vi "Q14070-Z060A.vi"() -> ()   [LabVIEW 2013]
uses:
  <vilib>/Utility/error.llb/whitespace.ctl
  <vilib>/Utility/file.llb/Read From Spreadsheet File (string).vi
  <vilib>/express/express arith-compare/Formula/XNode/ExpressFormulaBlockNode.xnode
  PCI8622_32.dll
  <vilib>/printing/EasyPrintingControls.llb/contents.ctl
  <vilib>/Utility/NIReport.llb/NI_ReportGenerationCore.lvlib
  <vilib>/printing/EasyPrintingControls.llb/report_type.ctl
  <vilib>/Utility/NIReport.llb/NI_report.lvclass
  <vilib>/printing/EasyPrinting.llb/Easy Print VI Panel or Documentation (path).vi
panel:
  in  "截取百分比":dbl=0.05
  in  "半行程":dbl=70.0
  in  "是否取消放行按钮":bool
  in  "齿条传动比":dbl=47.34 format="%#_13g"
  in  "机械间隙值":dbl=3.5
  out "最大轴向力标准(N)":dbl=200.0 caption="L+Lmax(mm)" format="%#.3f"
  out "右平均轴向力(N)":dbl caption="L+Lmax(mm)" format="%#.3f"
  out "左平均轴向力(N)":dbl caption="最大位移偏离Lmax(mm)" format="%#.3f"
  out "员工ID":string
  out "急停":bool
  out "报警":dbl
  out "报警提示":string
  out "DeviceHandle":u32
  in  "设定轴向力调整次数":dbl=6.0
  out "出支线工步号":u32
  in  "最小间隙(mm)":dbl=0.001 format="%#.3f"
  in  "测头气缸右移":bool
  in  "测头气缸左移":bool
  in  "轴向力已做次数":dbl
  out "全行程间隙及轴向力合格":bool
  out "轴向力启动":bool
  out "间隙启动":bool
  in  "夹头松开":bool
  in  "夹头夹紧":bool
  out "找帽扭矩":dbl=10.0 caption="压力传感器" format="%#.2f"
  out "error out":errorcluster
  out "型号数量":i32
  out "error out 4":errorcluster
  in  "设定间隙调整次数":dbl=6.0
  out "读取产品ID":string
  out "下工位备料":bool
  out "下工位测试":bool
  out "下工位自动":bool
  out "下工位备料H":bool
  out "下工位测试H":bool
  out "下工位自动H":bool
  out "FGCS":string
  out "KSJJ":string
  out "Z060ARFID":string
  out "轴向力Y":dbl[](array[numeric])
  out "轴向力X":dbl[](array[numeric])
  out "间隙X数组":dbl[](array[numeric])
  out "间隙Y数组":dbl[](array[numeric])
  out "error out 3":errorcluster caption="错误输出"
  out "rfid工步号":u32
  out "芯片ID":string="201209190001"
  out "rfid完成":bool
  out "rfid触发":bool
  out "本序已做":bool
  in  "回零完成":bool
  in  "电动缸回零":bool
  in  "已调试次数":dbl
  in  "需调整角度(度)":dbl
  in  "转向器中心":dbl
  out "扭矩到达":bool
  out "黄灯":bool
  out "红灯":bool
  in  "基准位移":dbl caption="压力传感器" format="%#.3f"
  out "上序不合格":bool
  out "单点间隙合格":bool
  out "上序合格":bool
  out "测头机构电机":u32
  out "复位":bool
  in  "型号选择":u16(ring)=1 items=["J709", "J728", "J706"]
  in  "联线按钮":bool
  in  "工步号":u32
  in  "产品ID":string="201209190001"
  out "间隙位移(mm)":dbl caption="压力传感器" format="%#.3f"
  out "齿条推拉力(N)":dbl format="%#.2f"
  out "齿条扭矩(Nm)":dbl format="%#.2f"
  out "通讯状态":bool
  out "员工姓名":string
  out "工步提示":string
  out "ADODB._Connection Out 2":refnum<k7>
  out "旋转齿条电机":u32
  out "电动缸电机":u32
  in  "停止":bool
  in  "参数加载":bool
  in  "选项卡控件":T1(tab)
  out "扭动曲线":cluster{"Y":dbl[], "Y":dbl[]}[](graph) caption="压球涨堵头1"
  out "中间位置间隙":dbl caption="间隙值L(mm)" format="%_2f"
  out "中间间隙标准(mm)":dbl=0.07 format="%#.3f"
  in  "找帽OK":bool
  out "全行程180°外间隙标准(mm)":dbl=0.1 format="%#.3f"
  out "右180°外全行程间隙":dbl caption="正向最大间隙L1(mm)" format="%_2f"
  out "左180°外全行程间隙":dbl caption="正向最大间隙L1(mm)" format="%_2f"
  out "右180°内全行程间隙":dbl caption="正向最大间隙L1(mm)" format="%_2f"
  out "左180°内全行程间隙":dbl caption="正向最大间隙L1(mm)" format="%_2f"
  out "全行程180°内间隙标准(mm)":dbl=0.07 format="%_1f"
  out "左全行程间隙":dbl caption="正向最大间隙L1(mm)" format="%#.3f"
  out "右全行程间隙":dbl caption="正向最大间隙L1(mm)" format="%#.3f"
  out "总圈数最大值":dbl format="%_3g"
  out "总圈数标准":dbl format="%_3g"
  out "总行程最大值":dbl
  out "总行程标准(mm)":dbl
  out "平均轴向力MAX(N)":dbl=200.0 caption="L+Lmax(mm)" format="%#.3f"
  out "力波动标准(N)":dbl=60.0 caption="L+Lmax(mm)" format="%#.3f"
  out "轴向力标准(N)":dbl=100.0 caption="L+Lmax(mm)" format="%#.3f"
  out "右最大轴向力(N)":dbl caption="L+Lmax(mm)" format="%#_5f"
  out "左轴向力波动(N)":dbl caption="最大位移偏离Lmax(mm)" format="%#_4f"
  out "左最大轴向力(N)":dbl caption="最大位移偏离Lmax(mm)" format="%#_5f"
  out "行程跳动曲线":cluster{"Y":dbl[], "Y":dbl[]}[](graph) caption="压球涨堵头1"
  out "右轴向力波动(N)":dbl format="%#_4f"
  out "总行程(mm)":dbl format="%#_5f"
  out "总圈数":dbl format="%.3g"
  in  "不合格品":bool
  in  "扭矩停止值":dbl=16.0
  in  "齿条右极限":dbl=-70.0 caption="压力传感器" format="%#.2f"
  in  "齿条左极限":dbl=-262.0 caption="压力传感器" format="%#.2f"
  in  "齿条移动速度":dbl=5.0 caption="压力传感器" format="%#.2f"
  in  "旋转伺服找帽转速":dbl=5.0 caption="压力传感器" format="%#.2f"
  in  "测量点扭矩":dbl=4.0 caption="压力传感器" format="%#.2f"
  in  "旋转伺服测量转速":dbl caption="压力传感器" format="%#.2f"
  in  "测头机构轴后退位":dbl=30.0 caption="压力传感器" format="%#.2f"
  in  "测头机构轴待检位":dbl caption="压力传感器" format="%#.2f"
  in  "测头机构轴检测位":dbl caption="压力传感器" format="%#.2f"
  in  "测头机构轴移动速度":dbl caption="压力传感器" format="%#.2f"
  out "点胶":bool
  in  "夹头松开":bool
  in  "夹头夹紧":bool
  in  "测头气缸右移":bool
  in  "测头气缸左移":bool
  in  "支线下降":bool
  in  "支线顶升":bool
  in  "出支线":bool
  in  "进支线":bool
  in  "主线下降":bool
  in  "主线顶升":bool
  in  "下阻挡器放行":bool
  in  "上阻挡器放行":bool
  out "夹头夹紧位":bool
  out "测头左位":bool
  out "测头右位":bool
  out "夹头松开":bool
  out "记号笔":bool
  in  "测头机构轴使能":bool
  in  "测头机构轴后退":bool
  in  "测头机构轴前进":bool
  in  "电动缸速度(mm/s)":dbl=10.0 format="%#.3f"
  out "电动缸位置(mm)":dbl=10000.0 format="%#.3f"
  in  "旋转伺服速度(°/s)":dbl=10.0 format="%#.3f"
  out "旋转伺服位置(°)":dbl=10000.0 format="%#.3f"
  in  "测头机构轴速度(mm/s)":dbl=10.0 format="%#.3f"
  out "测头机构轴位置(mm)":dbl=10000.0 format="%#.3f"
  in  "旋转齿条轴右转":bool
  in  "旋转齿条轴左转":bool
  in  "旋转齿条轴使能":bool
  in  "电动缸后退":bool
  in  "电动缸使能":bool
  in  "电动缸前进":bool
  in  "齿条扭矩比例偏移":dbl=1.0 format="%#.2f"
  in  "齿条扭矩零点偏移":dbl format="%#.2f"
  in  "齿条推拉力比例偏移":dbl=1.0 format="%#.2f"
  in  "齿条推拉力零点偏移":dbl format="%#.2f"
  in  "间隙位移比例偏移":dbl=1.0 format="%#.2f"
  in  "间隙位移零点偏移":dbl format="%#.2f"
  in  "传感器参数保存":bool
  in  "参数修改":bool
  in  "参数查询":bool
  in  "参数浏览表":string[][](table)
  # "芜湖机械转向器装配线"
  # "间隙及轴向力检测"
  # "Q14070机械转向器装配线"
  # "湖北唯思凌科装备制造有限公司 设计开发 (C)2015"
  # "≤"
  # "间隙测量判定值"
  # "间隙测量结果"
  # "≤"
  # "≤"
  # "≤"
  # "轴向力测量结果"
  # "轴向力测量标准"
  # "≤"
  # "≥"
  # "≤"
  # "≥"
  # "≤"
  # "≥"
  # "≤"
  # "不得大于20NM"
  # "传感器校验区"
  # "关于传感器校验：\n1、传感器校验需要由具备资质的单位或部门进行校验。\n2、具备权限的用户才能够修改传感器校验参数和试验参数。\n3、修改校验参数方法：先将比例偏移置为1，修改零点偏移，使零点值与校验的传感器一致；然后根据增幅调整比例偏移。"
  # "注意：\n具备权限的用户才能够修改传感器校验参数和试验参数！"
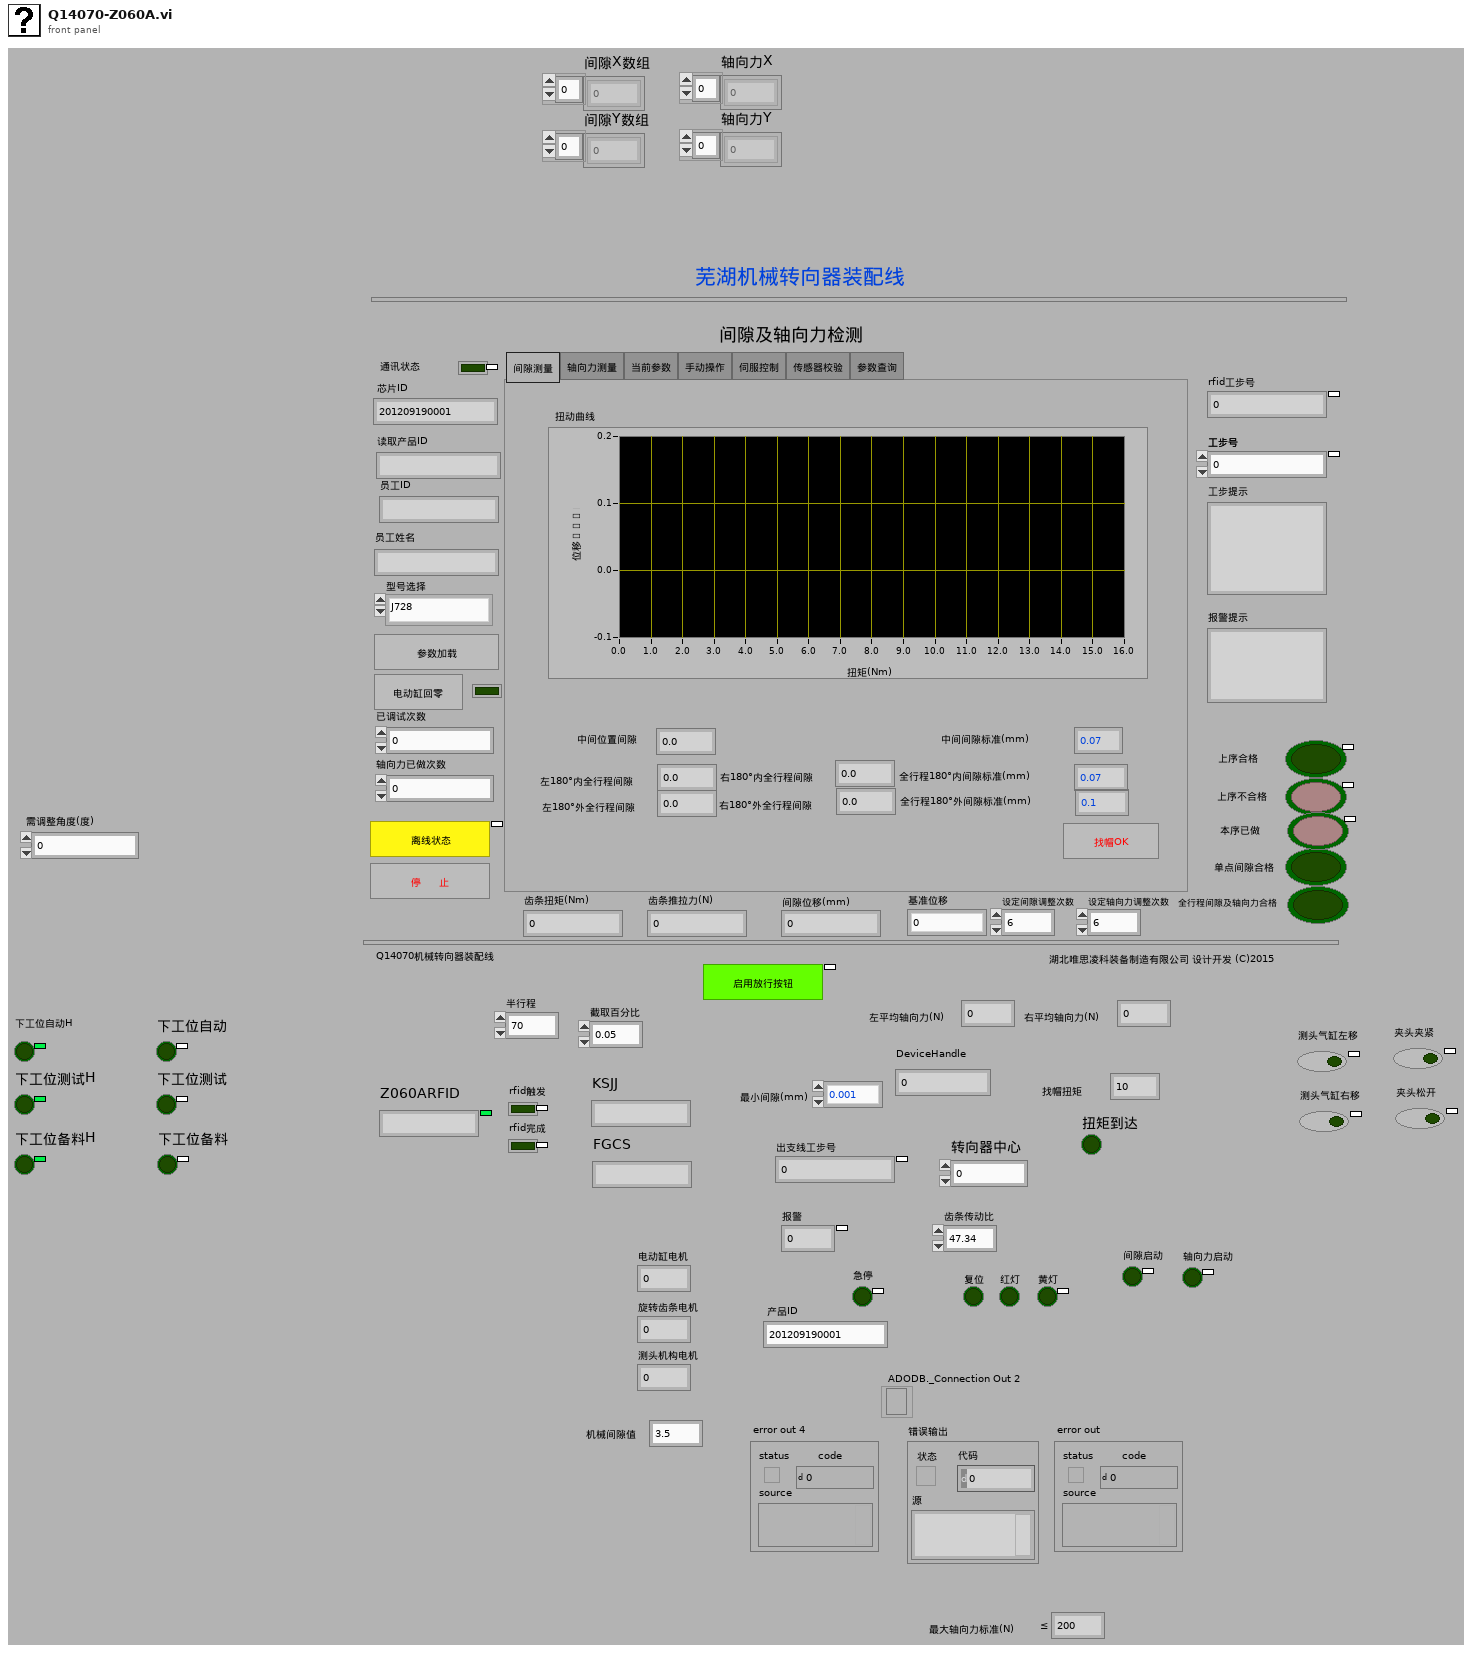
[diagram p1: front panel]
types:
  T1 = enum32{"间隙测量", "轴向力测量", "当前参数", "手动操作", "伺服控制", "传感器校验", "参数查询"}
  T2 = typedef "NI_ReportGenerationCore.lvlib/report_type.ctl" = u16
  T3 = typedef "NI_ReportGenerationCore.lvlib/contents.ctl" = u16
  T4 = typedef "imagedata.ctl" = cluster{"image type":i32, "image depth":i32, "image":u8[], "mask":u8[], "colors":u32[], "Rectangle":cluster{"left":i16, "top":i16, "right":i16, "bottom":i16}}
  T5 = enum8{"Enabled", "Disabled", "Disabled and Grayed Out"}
  T6 = typedef "whitespace.ctl" = u16
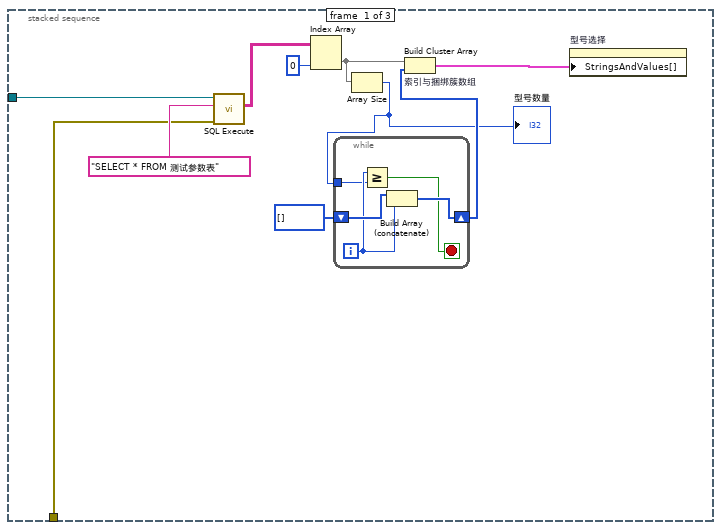
[diagram p4: hidden frame]
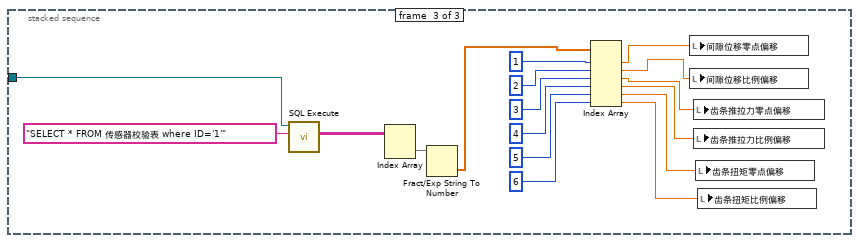
[diagram p5: hidden frame]
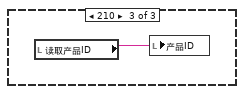
[diagram p7: hidden frame]
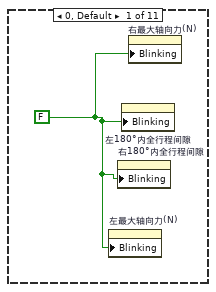
[diagram p8: hidden frame]
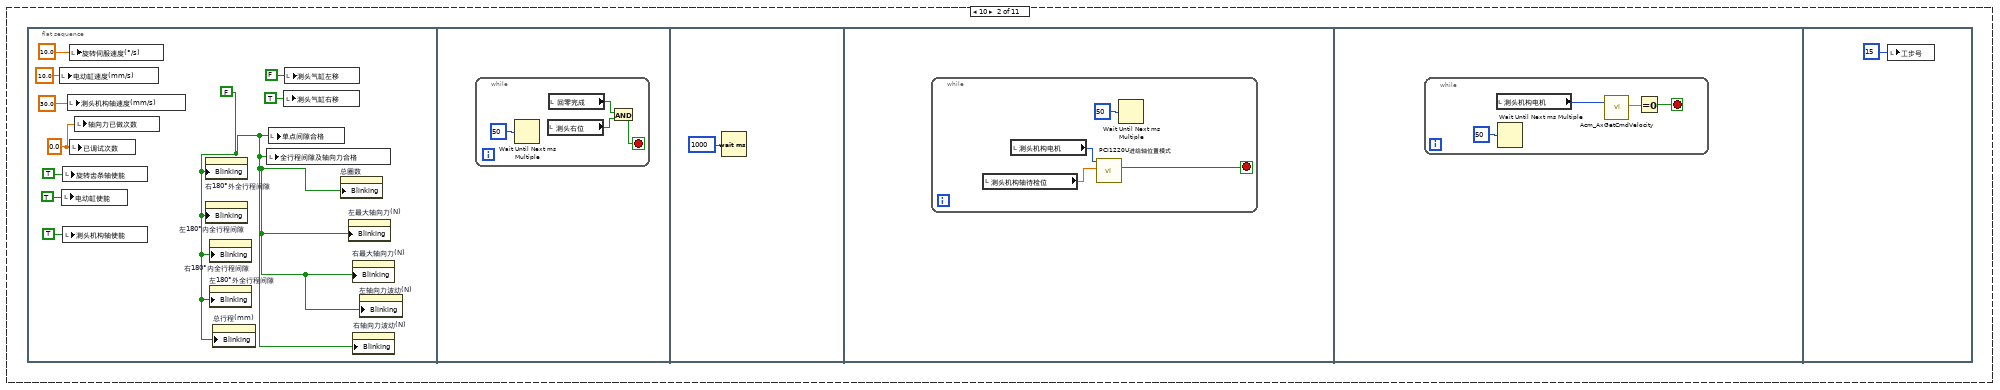
[diagram p9: hidden frame]
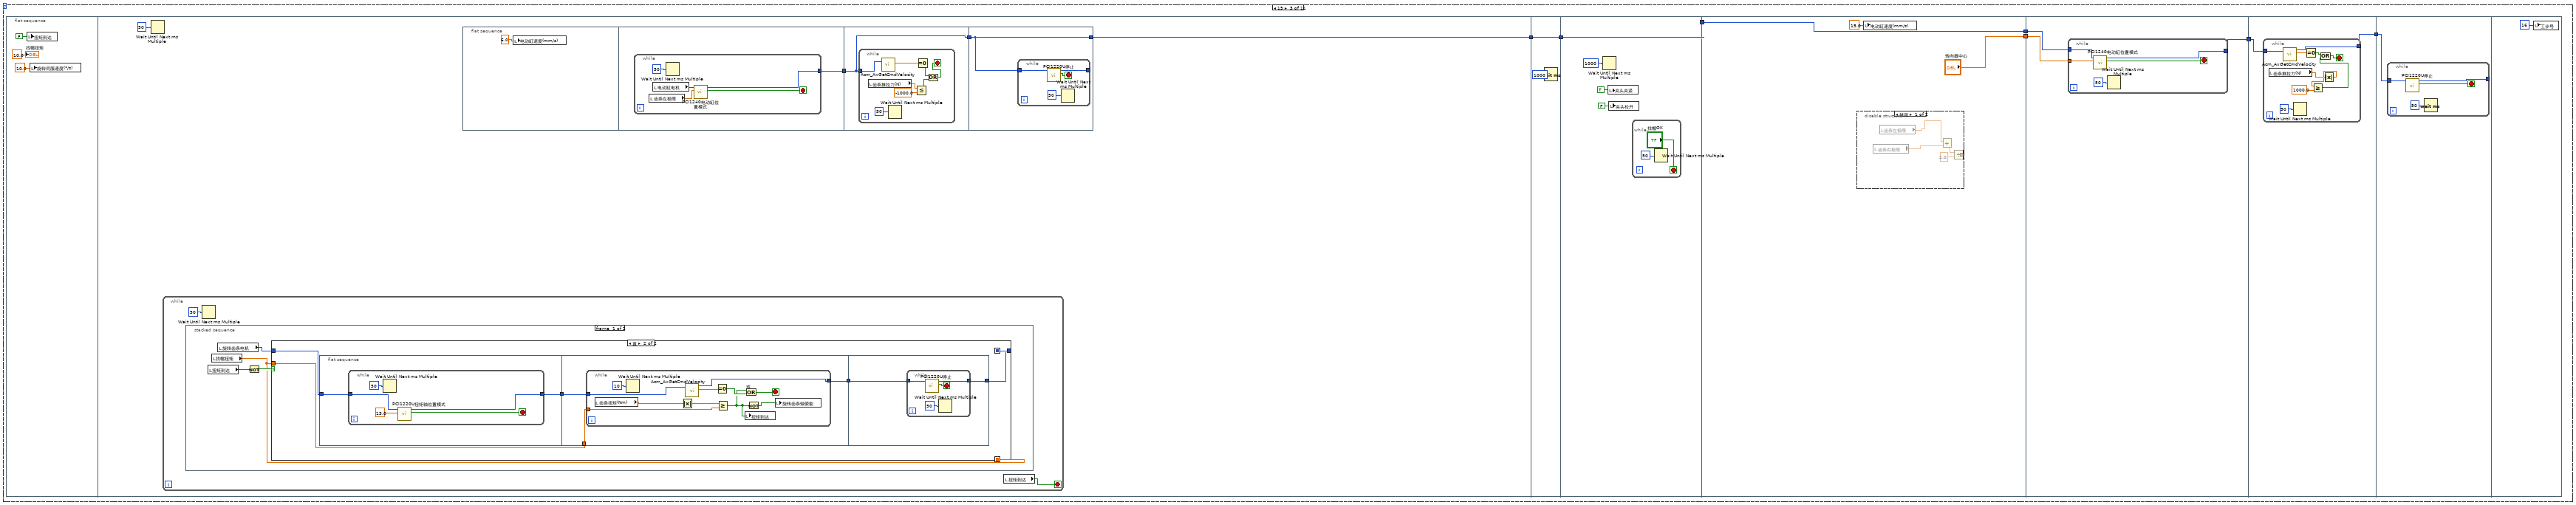
[diagram p10: hidden frame]
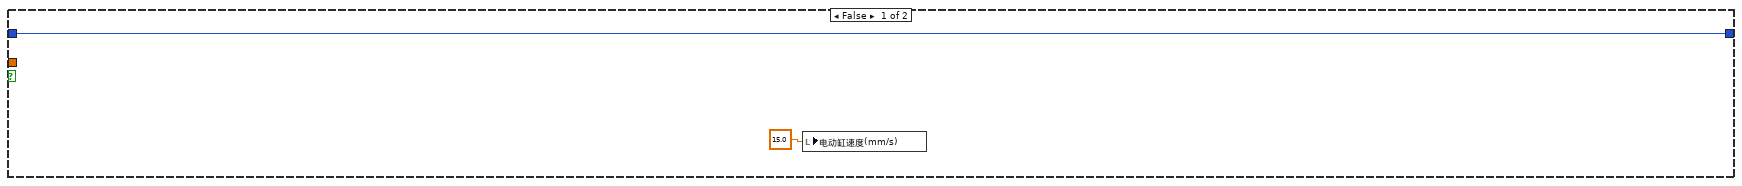
[diagram p11: hidden frame]
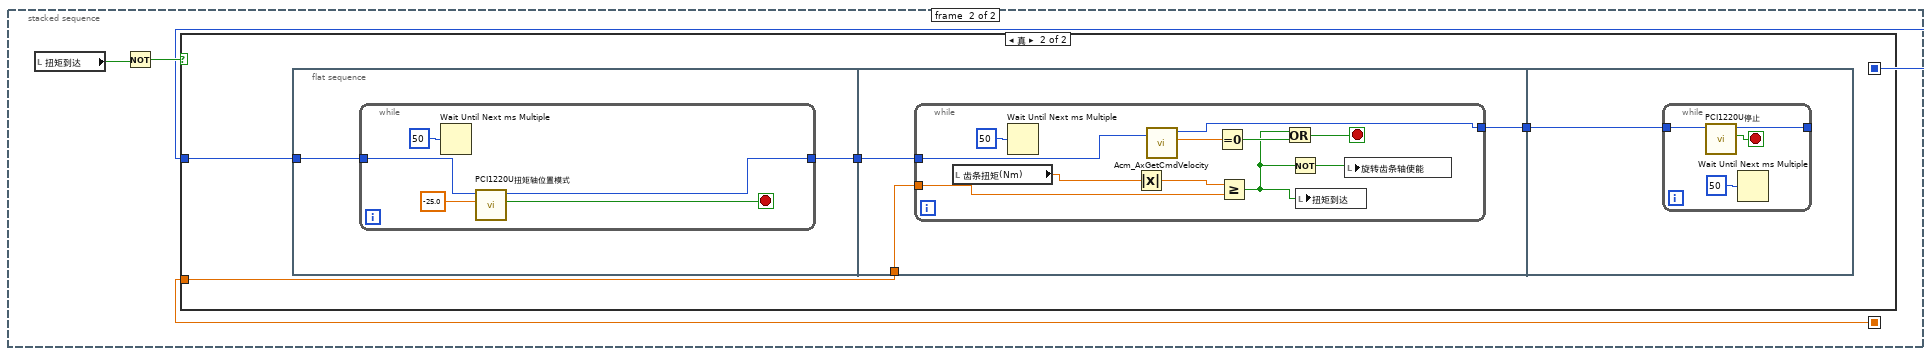
[diagram p12: hidden frame]
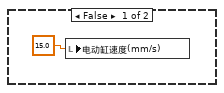
[diagram p13: hidden frame]
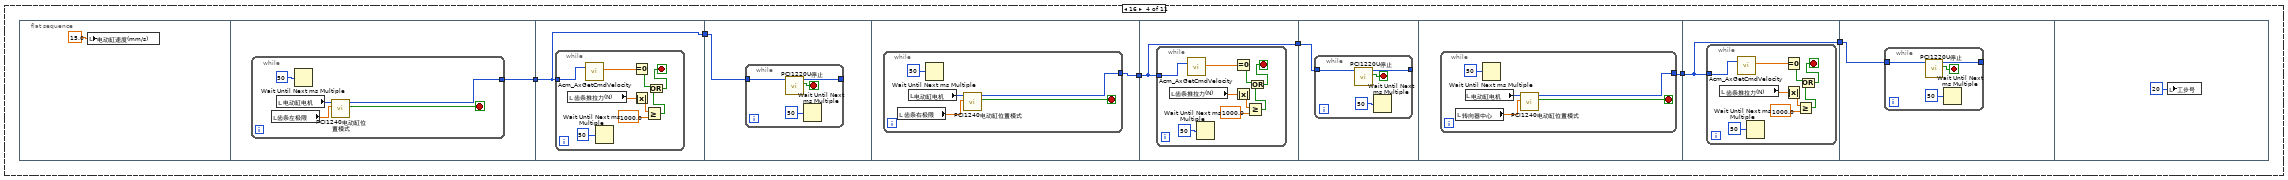
[diagram p15: hidden frame]
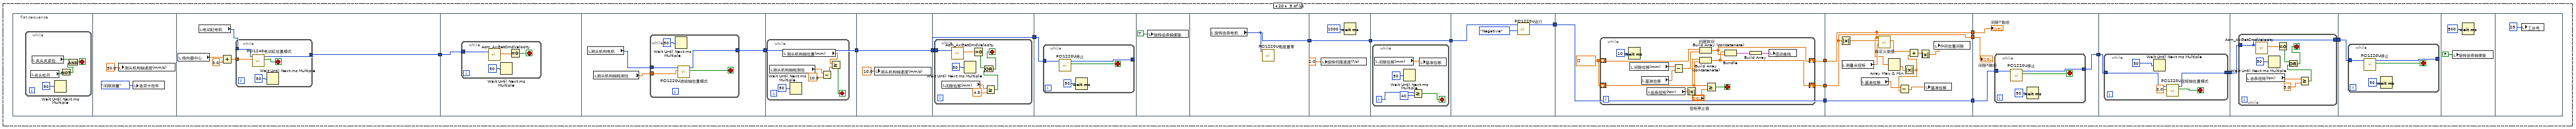
[diagram p16: hidden frame]
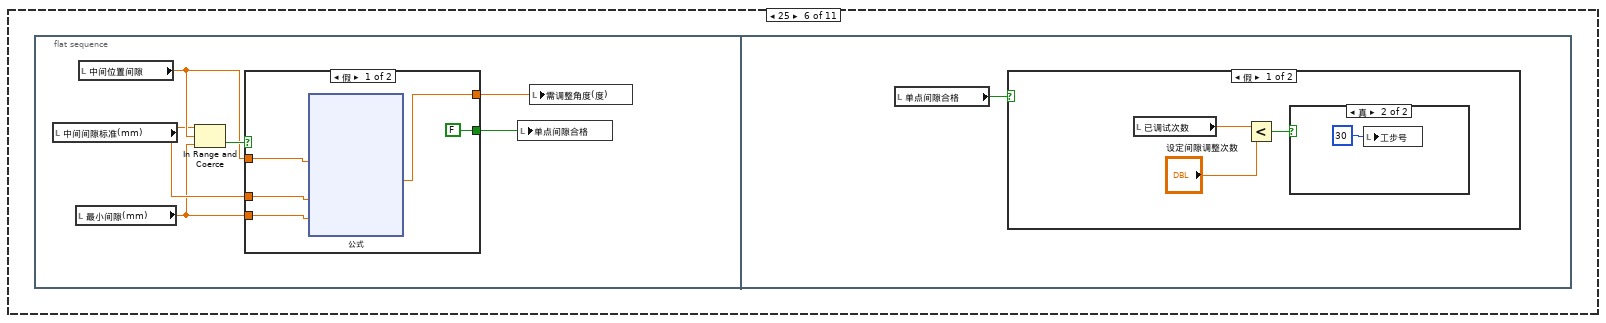
[diagram p17: hidden frame]
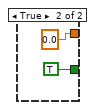
[diagram p18: hidden frame]
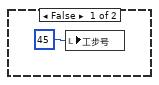
[diagram p19: hidden frame]
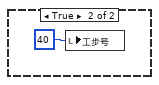
[diagram p20: hidden frame]
diagram:
  n1 = while {
    stop <- w7 stop-if-true
    n2 = local read "工步号"() -> (w5:u32)
    n3 = case shown="40" w5 {
      frame 0, Default {
        w8 = FALSE ("闪烁")
        n4 = property on="左最大轴向力(N)" class="DigNum (严格)"("Blinking"=w8) -> ()  [unwired: 2 in, 2 out]
        n5 = property on="右180°内全行程间隙" class="DigNum (严格)"("Blinking"=w8) -> ()  [unwired: 2 in, 2 out]
        n6 = property on="左180°内全行程间隙" class="DigNum (严格)"("Blinking"=w8) -> ()  [unwired: 2 in, 2 out]
        n7 = property on="右最大轴向力(N)" class="DigNum (严格)"("Blinking"=w8) -> ()  [unwired: 2 in, 2 out]
      }
      frame 10 {
        n8 = flat-sequence {
          frame #0 {
            w9 = FALSE ("单点间隙合格")
            w10 = 0.0 ("已调试次数")
            n9 = local write "电动缸速度(mm/s)"(10.0 ("电动缸速度(mm/s)")) -> ()
            n10 = local write "电动缸使能"(TRUE ("电动缸使能")) -> ()
            n11 = local write "旋转齿条轴使能"(TRUE ("旋转齿条轴使能")) -> ()
            n12 = local write "测头机构轴使能"(TRUE ("调整机构轴使能")) -> ()
            n13 = local write "测头机构轴速度(mm/s)"(30.0 ("调整机构轴速度(mm/s)")) -> ()
            n14 = local write "旋转伺服速度(°/s)"(10.0 ("旋转齿条轴速度(°/s)")) -> ()
            n15 = local write "已调试次数"(w10) -> ()
            n16 = local write "轴向力已做次数"(w10) -> ()
            n17 = property on="右180°外全行程间隙" class="DigNum (严格)"("Blinking"=w9) -> ()  [unwired: 2 in, 2 out]
            n18 = property on="左180°内全行程间隙" class="DigNum (严格)"("Blinking"=w9) -> ()  [unwired: 2 in, 2 out]
            n19 = property on="右180°内全行程间隙" class="DigNum (严格)"("Blinking"=w9) -> ()  [unwired: 2 in, 2 out]
            n20 = property on="左180°外全行程间隙" class="DigNum (严格)"("Blinking"=w9) -> ()  [unwired: 2 in, 2 out]
            n21 = property on="总行程(mm)" class="DigNum (严格)"("Blinking"=w9) -> ()  [unwired: 2 in, 2 out]
            n22 = local write "全行程间隙及轴向力合格"(w9) -> ()
            n23 = local write "单点间隙合格"(w9) -> ()
            n24 = local write "测头气缸右移"(TRUE ("测头气缸右移")) -> ()
            n25 = local write "测头气缸左移"(FALSE ("测头气缸左移")) -> ()
            n26 = property on="总圈数" class="DigNum (严格)"("Blinking"=w9) -> ()  [unwired: 2 in, 2 out]
            n27 = property on="左最大轴向力(N)" class="DigNum (严格)"("Blinking"=w9) -> ()  [unwired: 2 in, 2 out]
            n28 = property on="右最大轴向力(N)" class="DigNum (严格)"("Blinking"=w9) -> ()  [unwired: 2 in, 2 out]
            n29 = property on="右轴向力波动(N)" class="DigNum (严格)"("Blinking"=w9) -> ()  [unwired: 2 in, 2 out]
            n30 = property on="左轴向力波动(N)" class="DigNum (严格)"("Blinking"=w9) -> ()  [unwired: 2 in, 2 out]
          }
          frame #1 {
            n31 = while {
              stop <- w19 stop-if-true
              n32 = Wait Until Next ms Multiple(millisecond multiple=u32 50 ("毫秒倍数")) -> ()  [unwired: 1 out]
              n33 = local read "测头右位"() -> (w20:bool)
              n34 = local read "回零完成"() -> (w21:bool)
              n35 = And(x=w21, y=w20) -> (x .and. y?=w19:bool)
            }
          }
          frame #2 {
            n36 = Wait (ms)(milliseconds to wait=u32 1000 ("等待时间（毫秒）")) -> ()  [unwired: 1 out]
          }
          frame #3 {
            n37 = while {
              stop <- w27 stop-if-true
              n38 = local read "测头机构轴待检位"() -> (w24:dbl)
              n39 = local read "测头机构电机"() -> (w25:u32)
              n40 = call "PCI1220U进给轴位置模式.vi"("Distance"=w24, "AxisHandle IN"=w25) -> ("AbsSuccess"=w27:bool)  [unwired: 8 in, 1 out]
              n41 = Wait Until Next ms Multiple(millisecond multiple=u32 50 ("毫秒倍数")) -> ()  [unwired: 1 out]
            }
          }
          frame #4 {
            n42 = while {
              stop <- w30 stop-if-true
              n43 = local read "测头机构电机"() -> (w28:u32)
              n44 = Wait Until Next ms Multiple(millisecond multiple=u32 50 ("毫秒倍数")) -> ()  [unwired: 1 out]
              n45 = call <userlib>:"Acm_AxGetCmdVelocity.vi"("AxisHandle"=w28) -> ("Velocity"=w31:dbl)  [unwired: 1 in, 3 out]
              n46 = Equal To 0?(x=w31) -> (x = 0?=w30:bool)
            }
          }
          frame #5 {
            n47 = local write "工步号"(u32 15 ("工步号")) -> ()
          }
        }
      }
      frame 15 {
        n48 = flat-sequence {
          tunnel: [w44] -> w34
          tunnel: w34 -> [w145]
          tunnel: [w145] -> w33
          tunnel: w33 -> [w148]
          tunnel: [w148] -> w36
          tunnel: [w153] -> w39
          tunnel: ["转向器中心"] -> w38
          tunnel: w36 -> [w153]
          tunnel: w39 -> [w162]
          tunnel: w38 -> [w161]
          tunnel: [w160] -> w37
          tunnel: w37 -> [w169]
          tunnel: [w168] -> w35
          tunnel: w35 -> [w180]
          frame #0 {
            n49 = local write "扭矩到达"(FALSE ("扭矩到达")) -> ()
            n50 = local write "旋转伺服速度(°/s)"(10.0 ("旋转齿条轴速度(°/s)")) -> ()
            "找帽扭矩" <- 10.0 ("找帽扭矩")
          }
          frame #1 {
            n51 = Wait Until Next ms Multiple(millisecond multiple=u32 50 ("毫秒倍数")) -> ()  [unwired: 1 out]
            n52 = while {
              stop <- w47 stop-if-true
              n53 = stacked-sequence {
                seq-local: [w49 _] -> [_ w90]
                seq-local: [w53 _] -> [_ w89]
                frame #0 {
                  n54 = local read "扭矩到达"() -> (w51:bool)
                  n55 = local read "找帽扭矩"() -> (w49:dbl)
                  n56 = local read "旋转齿条电机"() -> (w50:u32)
                  n57 = Not(x=w51) -> (.not. x?=w52:bool)
                  n58 = case shown="真" w52 {
                    tunnel: [w55 w56] -> w53
                    tunnel: w50 -> [w55 w60]
                    tunnel: w49 -> [_ w58]
                    frame False {
                      n59 = local write "电动缸速度(mm/s)"(15.0 ("电动缸速度(mm/s)")) -> ()
                    }
                    frame True {
                      n60 = flat-sequence {
                        tunnel: w60 -> [w62]
                        tunnel: [w61] -> w59
                        tunnel: w59 -> [w70]
                        tunnel: w58 -> [w69]
                        tunnel: [w68] -> w57
                        tunnel: w57 -> [w83]
                        tunnel: [w82] -> w56
                        frame #0 {
                          n61 = while {
                            tunnel: [w66] -> w61
                            tunnel: w62 -> [w63]
                            stop <- w65 stop-if-true
                            n62 = Wait Until Next ms Multiple(millisecond multiple=u32 50 ("毫秒倍数")) -> ()  [unwired: 1 out]
                            n63 = call "PCI1220U扭矩轴位置模式.vi"("Distance"=13.0, "AxisHandle IN"=w63) -> ("AbsSuccess"=w65:bool, "AxisHandle OUT"=w66:u32)  [unwired: 8 in]
                          }
                        }
                        frame #1 {
                          n64 = while {
                            tunnel: w70 -> [w80]
                            tunnel: w69 -> [w75]
                            tunnel: [w74] -> w68
                            stop <- w76 stop-if-true
                            n65 = local read "齿条扭矩(Nm)"() -> (w73:dbl)
                            n66 = Wait Until Next ms Multiple(millisecond multiple=u32 10 ("毫秒倍数")) -> ()  [unwired: 1 out]
                            n67 = Absolute Value(x=w73) -> (abs(x)=w78:dbl)
                            n68 = call <userlib>:"Acm_AxGetCmdVelocity.vi"("AxisHandle"=w80) -> ("Velocity"=w79:dbl, "AxisHandle"=w74:u32)  [unwired: 1 in, 2 out]
                            n69 = Equal To 0?(x=w79) -> (x = 0?=w77:bool)
                            n70 = Greater Or Equal?(x=w78, y=w75) -> (x >= y?=w72:bool)
                            n71 = Or "或"(x=w72, y=w77) -> (x .or. y?=w76:bool)
                            n72 = local write "扭矩到达"(w72) -> ()
                            n73 = Not(x=w72) -> (.not. x?=w71:bool)
                            n74 = local write "旋转齿条轴使能"(w71) -> ()
                          }
                        }
                        frame #2 {
                          n75 = while {
                            tunnel: w83 -> [w87]
                            tunnel: [w84] -> w82
                            stop <- w86 stop-if-true
                            n76 = call "PCI1220U停止.vi"("AxisHandle IN"=w87) -> ("完成"=w86:bool, "AxisHandle OUT"=w84:u32)  [unwired: 9 in]
                            n77 = Wait Until Next ms Multiple(millisecond multiple=u32 50 ("毫秒倍数")) -> ()  [unwired: 1 out]
                          }
                        }
                      }
                    }
                  }
                }
                frame #1 {
                  n78 = local read "扭矩到达"() -> (w88:bool)
                  n79 = Not(x=w88) -> (.not. x?=w91:bool)
                  n80 = case shown="真" w91 {
                    tunnel: w89 -> [_ w96]
                    tunnel: w90 -> [_ w94]
                    frame False {
                      n81 = local write "电动缸速度(mm/s)"(15.0 ("电动缸速度(mm/s)")) -> ()
                    }
                    frame True {
                      n82 = flat-sequence {
                        tunnel: w96 -> [w97]
                        tunnel: [w98] -> w95
                        tunnel: w95 -> [w106]
                        tunnel: w94 -> [w105]
                        tunnel: [w104] -> w93
                        tunnel: w93 -> [w118]
                        frame #0 {
                          n83 = while {
                            tunnel: [w102] -> w98
                            tunnel: w97 -> [w99]
                            stop <- w101 stop-if-true
                            n84 = Wait Until Next ms Multiple(millisecond multiple=u32 50 ("毫秒倍数")) -> ()  [unwired: 1 out]
                            n85 = call "PCI1220U扭矩轴位置模式.vi"("Distance"=-25.0, "AxisHandle IN"=w99) -> ("AbsSuccess"=w101:bool, "AxisHandle OUT"=w102:u32)  [unwired: 8 in]
                          }
                        }
                        frame #1 {
                          n86 = while {
                            tunnel: w106 -> [w116]
                            tunnel: [w111] -> w104
                            tunnel: w105 -> [w110]
                            stop <- w112 stop-if-true
                            n87 = local read "齿条扭矩(Nm)"() -> (w109:dbl)
                            n88 = Wait Until Next ms Multiple(millisecond multiple=u32 50 ("毫秒倍数")) -> ()  [unwired: 1 out]
                            n89 = Absolute Value(x=w109) -> (abs(x)=w114:dbl)
                            n90 = call <userlib>:"Acm_AxGetCmdVelocity.vi"("AxisHandle"=w116) -> ("Velocity"=w115:dbl, "AxisHandle"=w111:u32)  [unwired: 1 in, 2 out]
                            n91 = Equal To 0?(x=w115) -> (x = 0?=w113:bool)
                            n92 = Greater Or Equal?(x=w114, y=w110) -> (x >= y?=w107:bool)
                            n93 = Or(x=w107, y=w113) -> (x .or. y?=w112:bool)
                            n94 = Not(x=w107) -> (.not. x?=w108:bool)
                            n95 = local write "扭矩到达"(w107) -> ()
                            n96 = local write "旋转齿条轴使能"(w108) -> ()
                          }
                        }
                        frame #2 {
                          n97 = while {
                            tunnel: w118 -> [w122]
                            tunnel: [w119] -> _
                            stop <- w121 stop-if-true
                            n98 = call "PCI1220U停止.vi"("AxisHandle IN"=w122) -> ("完成"=w121:bool, "AxisHandle OUT"=w119:u32)  [unwired: 9 in]
                            n99 = Wait Until Next ms Multiple(millisecond multiple=u32 50 ("毫秒倍数")) -> ()  [unwired: 1 out]
                          }
                        }
                      }
                    }
                  }
                }
              }
              n100 = Wait Until Next ms Multiple(millisecond multiple=u32 50 ("毫秒倍数")) -> ()  [unwired: 1 out]
              n101 = local read "扭矩到达"() -> (w47:bool)
            }
            n102 = flat-sequence {
              tunnel: [w124] -> w46
              tunnel: w46 -> [w130]
              tunnel: [w130] -> w43
              tunnel: [w139] -> w44
              tunnel: w43 -> [w139]
              frame #0 {
                n103 = local write "电动缸速度(mm/s)"(6.0 ("电动缸速度(mm/s)")) -> ()
              }
              frame #1 {
                n104 = while {
                  tunnel: [w128] -> w124
                  stop <- w127 stop-if-true
                  n105 = local read "齿条左极限"() -> (w125:dbl)
                  n106 = local read "电动缸电机"() -> (w129:u32)
                  n107 = Wait Until Next ms Multiple(millisecond multiple=u32 50 ("毫秒倍数")) -> ()  [unwired: 1 out]
                  n108 = call "PCI1240电动缸位置模式 .vi"("Distance"=w125, "AxisHandle IN"=w129) -> ("AbsSuccess"=w127:bool, "AxisHandle OUT"=w128:u32)  [unwired: 8 in]
                }
              }
              frame #2 {
                n109 = while {
                  tunnel: w130 -> [w137]
                  stop <- w134 stop-if-true
                  n110 = local read "齿条推拉力(N)"() -> (w133:dbl)
                  n111 = call <userlib>:"Acm_AxGetCmdVelocity.vi"("AxisHandle"=w137) -> ("Velocity"=w138:dbl)  [unwired: 1 in, 3 out]
                  n112 = Wait Until Next ms Multiple(millisecond multiple=u32 50 ("毫秒倍数")) -> ()  [unwired: 1 out]
                  n113 = Less Or Equal?(x=w133, y=-1000.0) -> (x <= y?=w131:bool)
                  n114 = Equal To 0?(x=w138) -> (x = 0?=w135:bool)
                  n115 = Or(x=w135, y=w131) -> (x .or. y?=w134:bool)
                }
              }
              frame #3 {
                n116 = while {
                  tunnel: w139 -> [w143]
                  tunnel: [w140] -> _
                  stop <- w142 stop-if-true
                  n117 = call "PCI1220U停止.vi"("AxisHandle IN"=w143) -> ("完成"=w142:bool, "AxisHandle OUT"=w140:u32)  [unwired: 9 in]
                  n118 = Wait Until Next ms Multiple(millisecond multiple=u32 50 ("毫秒倍数")) -> ()  [unwired: 1 out]
                }
              }
            }
          }
          frame #2 {
            n119 = Wait (ms)(milliseconds to wait=u32 1000 ("等待时间（毫秒）")) -> ()  [unwired: 1 out]
          }
          frame #3 {
            n120 = Wait Until Next ms Multiple(millisecond multiple=u32 1000 ("毫秒倍数")) -> ()  [unwired: 1 out]
            n121 = local write "夹头夹紧"(TRUE ("夹头夹紧")) -> ()
            n122 = local write "夹头松开"(FALSE ("夹头松开")) -> ()
            n123 = while {
              stop <- "找帽OK" stop-if-true
              n124 = Wait Until Next ms Multiple(millisecond multiple=u32 50 ("毫秒倍数")) -> ()  [unwired: 1 out]
            }
          }
          frame #4 {
            n125 = disable-structure shown="禁用" {
              disable-tunnel: [w157 _] -> _
              frame Disabled {
                n126 = local read "齿条右极限"() -> (w155:dbl)
                n127 = local read "齿条左极限"() -> (w156:dbl)
                n128 = Add(x=w156, y=w155) -> (x+y=w159:dbl)
                n129 = Divide(x=w159, y=2.0) -> (x/y=w157:dbl)
              }
              frame Enabled {
              }
            }
            n130 = local write "电动缸速度(mm/s)"(15.0 ("电动缸轴移动速度")) -> ()
          }
          frame #5 {
            n131 = while {
              tunnel: w162 -> [w167]
              tunnel: w161 -> [w166]
              tunnel: [w163] -> w160
              stop <- w165 stop-if-true
              n132 = call "PCI1240电动缸位置模式 .vi"("Distance"=w166, "AxisHandle IN"=w167) -> ("AbsSuccess"=w165:bool, "AxisHandle OUT"=w163:u32)  [unwired: 8 in]
              n133 = Wait Until Next ms Multiple(millisecond multiple=u32 50 ("毫秒倍数")) -> ()  [unwired: 1 out]
            }
          }
          frame #6 {
            n134 = while {
              tunnel: w169 -> [w179]
              tunnel: [w170] -> w168
              stop <- w171 stop-if-true
              n135 = local read "齿条推拉力(N)"() -> (w176:dbl)
              n136 = call <userlib>:"Acm_AxGetCmdVelocity.vi"("AxisHandle"=w179) -> ("Velocity"=w178:dbl, "AxisHandle"=w170:u32)  [unwired: 1 in, 2 out]
              n137 = Wait Until Next ms Multiple(millisecond multiple=u32 50 ("毫秒倍数")) -> ()  [unwired: 1 out]
              n138 = Equal To 0?(x=w178) -> (x = 0?=w173:bool)
              n139 = Absolute Value(x=w176) -> (abs(x)=w175:dbl)
              n140 = Greater Or Equal?(x=w175, y=1000.0) -> (x >= y?=w172:bool)
              n141 = Or(x=w173, y=w172) -> (x .or. y?=w171:bool)
            }
          }
          frame #7 {
            n142 = while {
              tunnel: w180 -> [w184]
              tunnel: [w183] -> _
              stop <- w182 stop-if-true
              n143 = call "PCI1220U停止.vi"("AxisHandle IN"=w184) -> ("完成"=w182:bool, "AxisHandle OUT"=w183:u32)  [unwired: 9 in]
              n144 = Wait (ms)(milliseconds to wait=u32 50 ("毫秒倍数")) -> ()  [unwired: 1 out]
            }
          }
          frame #8 {
            n145 = local write "工步号"(u32 16 ("工步号")) -> ()
          }
        }
      }
      frame 16 {
        n146 = flat-sequence {
          tunnel: [w193] -> w191
          tunnel: w191 -> [w199]
          tunnel: [w199] -> w190
          tunnel: w190 -> [w209]
          tunnel: [w214] -> w189
          tunnel: w189 -> [w220]
          tunnel: [w220] -> w188
          tunnel: w188 -> [w230]
          tunnel: [w235] -> w187
          tunnel: w187 -> [w241]
          tunnel: [w241] -> w186
          tunnel: w186 -> [w251]
          frame #0 {
            n147 = local write "电动缸速度(mm/s)"(15.0 ("电动缸速度(mm/s)")) -> ()
          }
          frame #1 {
            n148 = while {
              tunnel: [w197] -> w193
              stop <- w196 stop-if-true
              n149 = local read "齿条左极限"() -> (w194:dbl)
              n150 = local read "电动缸电机"() -> (w198:u32)
              n151 = Wait Until Next ms Multiple(millisecond multiple=u32 50 ("毫秒倍数")) -> ()  [unwired: 1 out]
              n152 = call "PCI1240电动缸位置模式 .vi"("Distance"=w194, "AxisHandle IN"=w198) -> ("AbsSuccess"=w196:bool, "AxisHandle OUT"=w197:u32)  [unwired: 8 in]
            }
          }
          frame #2 {
            n153 = while {
              tunnel: w199 -> [w207]
              stop <- w204 stop-if-true
              n154 = local read "齿条推拉力(N)"() -> (w203:dbl)
              n155 = call <userlib>:"Acm_AxGetCmdVelocity.vi"("AxisHandle"=w207) -> ("Velocity"=w208:dbl)  [unwired: 1 in, 3 out]
              n156 = Wait Until Next ms Multiple(millisecond multiple=u32 50 ("毫秒倍数")) -> ()  [unwired: 1 out]
              n157 = Equal To 0?(x=w208) -> (x = 0?=w205:bool)
              n158 = Absolute Value(x=w203) -> (abs(x)=w202:dbl)
              n159 = Greater Or Equal?(x=w202, y=1000.0) -> (x >= y?=w200:bool)
              n160 = Or(x=w205, y=w200) -> (x .or. y?=w204:bool)
            }
          }
          frame #3 {
            n161 = while {
              tunnel: w209 -> [w213]
              tunnel: [w210] -> _
              stop <- w212 stop-if-true
              n162 = call "PCI1220U停止.vi"("AxisHandle IN"=w213) -> ("完成"=w212:bool, "AxisHandle OUT"=w210:u32)  [unwired: 9 in]
              n163 = Wait Until Next ms Multiple(millisecond multiple=u32 50 ("毫秒倍数")) -> ()  [unwired: 1 out]
            }
          }
          frame #4 {
            n164 = while {
              tunnel: [w218] -> w214
              stop <- w217 stop-if-true
              n165 = local read "齿条右极限"() -> (w215:dbl)
              n166 = local read "电动缸电机"() -> (w219:u32)
              n167 = Wait Until Next ms Multiple(millisecond multiple=u32 50 ("毫秒倍数")) -> ()  [unwired: 1 out]
              n168 = call "PCI1240电动缸位置模式 .vi"("Distance"=w215, "AxisHandle IN"=w219) -> ("AbsSuccess"=w217:bool, "AxisHandle OUT"=w218:u32)  [unwired: 8 in]
            }
          }
          frame #5 {
            n169 = while {
              tunnel: w220 -> [w228]
              stop <- w225 stop-if-true
              n170 = local read "齿条推拉力(N)"() -> (w224:dbl)
              n171 = call <userlib>:"Acm_AxGetCmdVelocity.vi"("AxisHandle"=w228) -> ("Velocity"=w229:dbl)  [unwired: 1 in, 3 out]
              n172 = Wait Until Next ms Multiple(millisecond multiple=u32 50 ("毫秒倍数")) -> ()  [unwired: 1 out]
              n173 = Equal To 0?(x=w229) -> (x = 0?=w226:bool)
              n174 = Absolute Value(x=w224) -> (abs(x)=w223:dbl)
              n175 = Greater Or Equal?(x=w223, y=1000.0) -> (x >= y?=w221:bool)
              n176 = Or(x=w226, y=w221) -> (x .or. y?=w225:bool)
            }
          }
          frame #6 {
            n177 = while {
              tunnel: w230 -> [w234]
              tunnel: [w231] -> _
              stop <- w233 stop-if-true
              n178 = call "PCI1220U停止.vi"("AxisHandle IN"=w234) -> ("完成"=w233:bool, "AxisHandle OUT"=w231:u32)  [unwired: 9 in]
              n179 = Wait Until Next ms Multiple(millisecond multiple=u32 50 ("毫秒倍数")) -> ()  [unwired: 1 out]
            }
          }
          frame #7 {
            n180 = while {
              tunnel: [w239] -> w235
              stop <- w238 stop-if-true
              n181 = local read "转向器中心"() -> (w236:dbl)
              n182 = local read "电动缸电机"() -> (w240:u32)
              n183 = Wait Until Next ms Multiple(millisecond multiple=u32 50 ("毫秒倍数")) -> ()  [unwired: 1 out]
              n184 = call "PCI1240电动缸位置模式 .vi"("Distance"=w236, "AxisHandle IN"=w240) -> ("AbsSuccess"=w238:bool, "AxisHandle OUT"=w239:u32)  [unwired: 8 in]
            }
          }
          frame #8 {
            n185 = while {
              tunnel: w241 -> [w249]
              stop <- w246 stop-if-true
              n186 = local read "齿条推拉力(N)"() -> (w245:dbl)
              n187 = call <userlib>:"Acm_AxGetCmdVelocity.vi"("AxisHandle"=w249) -> ("Velocity"=w250:dbl)  [unwired: 1 in, 3 out]
              n188 = Wait Until Next ms Multiple(millisecond multiple=u32 50 ("毫秒倍数")) -> ()  [unwired: 1 out]
              n189 = Equal To 0?(x=w250) -> (x = 0?=w247:bool)
              n190 = Absolute Value(x=w245) -> (abs(x)=w244:dbl)
              n191 = Greater Or Equal?(x=w244, y=1000.0) -> (x >= y?=w242:bool)
              n192 = Or(x=w247, y=w242) -> (x .or. y?=w246:bool)
            }
          }
          frame #9 {
            n193 = while {
              tunnel: w251 -> [w255]
              tunnel: [w252] -> _
              stop <- w254 stop-if-true
              n194 = call "PCI1220U停止.vi"("AxisHandle IN"=w255) -> ("完成"=w254:bool, "AxisHandle OUT"=w252:u32)  [unwired: 9 in]
              n195 = Wait Until Next ms Multiple(millisecond multiple=u32 50 ("毫秒倍数")) -> ()  [unwired: 1 out]
            }
          }
          frame #10 {
            n196 = local write "工步号"(u32 20 ("工步号")) -> ()
          }
        }
      }
      frame 20 {
        n197 = flat-sequence {
          tunnel: [w286] -> w267
          tunnel: w267 -> [w292]
          tunnel: [w298] -> w259
          tunnel: w259 -> [w305]
          tunnel: [w305] -> w258
          tunnel: w258 -> [w313]
          tunnel: [w313] -> w257
          tunnel: w257 -> [w314]
          tunnel: [w314] -> w266
          tunnel: w266 -> [w323]
          tunnel: [w329] -> w264
          tunnel: [w331] -> w265
          tunnel: w264 -> [w331]
          tunnel: [w333] -> w260
          tunnel: w265 -> [w333]
          tunnel: w260 -> [w340]
          tunnel: [w339] -> w271
          tunnel: [w344] -> w270
          tunnel: [w343] -> w269
          tunnel: w271 -> [w342]
          tunnel: [w342] -> w268
          tunnel: [w371] -> w274
          tunnel: [w368] -> w273
          tunnel: w270 -> [w368]
          tunnel: [w367] -> w272
          tunnel: w269 -> [w367]
          tunnel: w268 -> [w371]
          tunnel: w274 -> [w375]
          tunnel: [w374] -> w263
          tunnel: w273 -> [w372]
          tunnel: w272 -> [w373]
          tunnel: w263 -> [w381]
          tunnel: [w380] -> w262
          tunnel: w262 -> [w388]
          tunnel: [w387] -> w261
          tunnel: w261 -> [w397]
          frame #0 {
            n198 = while {
              stop <- w277 stop-if-true
              n199 = local read "夹头松开"() -> (w278:bool)
              n200 = local read "夹头夹紧位"() -> (w276:bool)
              n201 = Wait Until Next ms Multiple(millisecond multiple=u32 50 ("毫秒倍数")) -> ()  [unwired: 1 out]
              n202 = Not(x=w278) -> (.not. x?=w275:bool)
              n203 = And(x=w276, y=w275) -> (x .and. y?=w277:bool)
            }
          }
          frame #1 {
            n204 = local write "测头机构轴速度(mm/s)"(30.0 ("测头机构轴速度(mm/s)")) -> ()
            n205 = local write "选项卡控件"(T1."间隙测量" ("选项卡控件")) -> ()
          }
          frame #2 {
            n206 = local read "转向器中心"() -> (w284:dbl)
            n207 = local read "电动缸电机"() -> (w285:u32)
            n208 = Add(x=w284, y=0.0) -> (x+y=w283:dbl)
            n209 = while {
              tunnel: w285 -> [w291]
              tunnel: w283 -> [w290]
              tunnel: [w287] -> w286
              stop <- w289 stop-if-true
              n210 = call "PCI1240电动缸位置模式 .vi"("Distance"=w290, "AxisHandle IN"=w291) -> ("AbsSuccess"=w289:bool, "AxisHandle OUT"=w287:u32)  [unwired: 8 in]
              n211 = Wait Until Next ms Multiple(millisecond multiple=u32 50 ("毫秒倍数")) -> ()  [unwired: 1 out]
            }
          }
          frame #3 {
            n212 = while {
              tunnel: w292 -> [w296]
              stop <- w294 stop-if-true
              n213 = call <userlib>:"Acm_AxGetCmdVelocity.vi"("AxisHandle"=w296) -> ("Velocity"=w295:dbl)  [unwired: 1 in, 3 out]
              n214 = Wait Until Next ms Multiple(millisecond multiple=u32 50 ("毫秒倍数")) -> ()  [unwired: 1 out]
              n215 = Equal To 0?(x=w295) -> (x = 0?=w294:bool)
            }
          }
          frame #4 {
            n216 = local read "测头机构电机"() -> (w299:u32)
            n217 = local read "测头机构轴检测位"() -> (w297:dbl)
            n218 = while {
              tunnel: w299 -> [w302]
              tunnel: w297 -> [w301]
              tunnel: [w300] -> w298
              stop <- w304 stop-if-true
              n219 = Wait Until Next ms Multiple(millisecond multiple=u32 50 ("毫秒倍数")) -> ()  [unwired: 1 out]
              n220 = call "PCI1220U进给轴位置模式.vi"("Distance"=w301, "AxisHandle IN"=w302) -> ("AbsSuccess"=w304:bool, "AxisHandle OUT"=w300:u32)  [unwired: 8 in]
            }
          }
          frame #5 {
            n221 = while {
              stop <- w306 stop-if-true
              n222 = local read "测头机构轴检测位"() -> (w310:dbl)
              n223 = local read "测头机构轴位置(mm)"() -> (w309:dbl)
              n224 = Wait Until Next ms Multiple(millisecond multiple=u32 50 ("毫秒倍数")) -> ()  [unwired: 1 out]
              n225 = Subtract(x=w310, y=10.0) -> (x-y=w307:dbl)
              n226 = Greater Or Equal?(x=w309, y=w307) -> (x >= y?=w306:bool)
            }
          }
          frame #6 {
            n227 = local write "测头机构轴速度(mm/s)"(10.0 ("测头机构轴速度(mm/s)")) -> ()
          }
          frame #7 {
            n228 = while {
              tunnel: w314 -> [w322]
              stop <- w316 stop-if-true
              n229 = local read "间隙位移(mm)"() -> (w319:dbl)
              n230 = call <userlib>:"Acm_AxGetCmdVelocity.vi"("AxisHandle"=w322) -> ("Velocity"=w321:dbl)  [unwired: 1 in, 3 out]
              n231 = Wait Until Next ms Multiple(millisecond multiple=u32 50 ("毫秒倍数")) -> ()  [unwired: 1 out]
              n232 = Equal To 0?(x=w321) -> (x = 0?=w317:bool)
              n233 = Greater Or Equal?(x=w319, y=4.5) -> (x >= y?=w315:bool)
              n234 = Or(x=w317, y=w315) -> (x .or. y?=w316:bool)
            }
          }
          frame #8 {
            n235 = while {
              tunnel: w323 -> [w327]
              tunnel: [w326] -> _
              stop <- w325 stop-if-true
              n236 = call "PCI1220U停止.vi"("AxisHandle IN"=w327) -> ("完成"=w325:bool, "AxisHandle OUT"=w326:u32)  [unwired: 9 in]
              n237 = Wait (ms)(milliseconds to wait=u32 50 ("毫秒倍数")) -> ()  [unwired: 1 out]
            }
          }
          frame #9 {
            n238 = local write "旋转齿条轴使能"(TRUE ("旋转齿条轴使能")) -> ()
          }
          frame #10 {
            n239 = local read "旋转齿条电机"() -> (w329:u32)
            n240 = call "PCI1220U角度置零.vi"("AxisHandle IN"=w329) -> ()  [unwired: 10 in, 1 out]
          }
          frame #11 {
            n241 = local write "旋转伺服速度(°/s)"(1.0 ("旋转齿条轴速度(°/s)")) -> ()
            n242 = Wait (ms)(milliseconds to wait=u32 1000 ("毫秒倍数")) -> ()  [unwired: 1 out]
          }
          frame #12 {
            n243 = while {
              i -> [w337]
              stop <- w334 stop-if-true
              n244 = local read "间隙位移(mm)"() -> (w338:dbl)
              n245 = Wait Until Next ms Multiple(millisecond multiple=u32 50 ("毫秒倍数")) -> ()  [unwired: 1 out]
              n246 = Greater Or Equal?(x=w337, y=40) -> (x >= y?=w334:bool)
              n247 = local write "基准位移"(w338) -> ()
            }
          }
          frame #13 {
            n248 = call "PCI1220U运行.vi"("方向"=enum32{"Negative", "Positive"}."Negative" ("Direction"), "AxisHandle IN"=w340) -> ("AxisHandle OUT"=w339:u32)  [unwired: 9 in]
          }
          frame #14 {
            w345 = dbl[] []
            n249 = while {
              shift-right: [w356] -> w344
              shift-left: w345 -> [w358]
              shift-right: [w355] -> w343
              shift-left: w345 -> [w357]
              stop <- w348 stop-if-true
              n250 = Wait (ms)(milliseconds to wait=u32 10 ("毫秒倍数")) -> ()  [unwired: 1 out]
              n251 = local read "间隙位移(mm)"() -> (w351:dbl)
              n252 = local read "基准位移"() -> (w349:dbl)
              n253 = local read "齿条扭矩(Nm)"() -> (w352:dbl)
              n254 = Subtract(x=w351, y=w349) -> (x-y=w350:dbl)
              n255 = Absolute Value(x=w352) -> (abs(x)=w347:dbl)
              n256 = Build Array (concatenate) "创建数组"(w357, w350) -> (w355:dbl[])
              n257 = Build Array (concatenate) ("创建数组")(w358, w347) -> (w356:dbl[])
              n258 = Greater Or Equal?(x=w347, y="扭矩停止值") -> (x >= y?=w348:bool)
              n259 = Bundle ("捆绑")(w356, w355) -> (w353:cluster{dbl[], dbl[]})  [unwired: 1 in]
              n260 = Build Array ("创建数组")(w353) -> (w354:cluster{dbl[], dbl[]}[])
              n261 = local write "扭动曲线"(w354) -> ()
            }
          }
          frame #15 {
            n262 = Absolute Value(x=w368) -> (abs(x)=w369:dbl[])
            n263 = local read "测量点扭矩"() -> (w370:dbl)
            n264 = local read "基准位移"() -> (w364:dbl)
            n265 = call "自定义插值.vi"("压力"=w370, "扭矩数组"=w369, "位移数组"=w367) -> ("扭矩值"=w365:dbl)  [unwired: 8 in]
            n266 = Array Max & Min(array=w367) -> (min value=w366:dbl)  [unwired: 3 out]
            n267 = Absolute Value(x=w366) -> (abs(x)=w363:dbl)
            n268 = Subtract(x=w364, y=w363) -> (x-y=w362:dbl)
            n269 = Add(x=w365, y=w363) -> (x+y=w361:dbl)
            n270 = Absolute Value(x=w361) -> (abs(x)=w360:dbl)
            n271 = local write "基准位移"(w362) -> ()
            n272 = local write "中间位置间隙"(w360) -> ()
          }
          frame #16 {
            n273 = while {
              tunnel: w375 -> [w379]
              tunnel: [w378] -> w374
              stop <- w377 stop-if-true
              n274 = call "PCI1220U停止.vi"("AxisHandle IN"=w379) -> ("完成"=w377:bool, "AxisHandle OUT"=w378:u32)  [unwired: 9 in]
              n275 = Wait (ms)(milliseconds to wait=u32 50 ("毫秒倍数")) -> ()  [unwired: 1 out]
            }
            "间隙Y数组" <- w373
            "间隙X数组" <- w372
          }
          frame #17 {
            n276 = while {
              tunnel: [w386] -> w380
              tunnel: w381 -> [w383]
              stop <- w385 stop-if-true
              n277 = Wait Until Next ms Multiple(millisecond multiple=u32 50 ("毫秒倍数")) -> ()  [unwired: 1 out]
              n278 = call "PCI1220U扭矩轴位置模式.vi"("Distance"=0.0, "AxisHandle IN"=w383) -> ("AbsSuccess"=w385:bool, "AxisHandle OUT"=w386:u32)  [unwired: 8 in]
            }
          }
          frame #18 {
            n279 = while {
              tunnel: w388 -> [w390]
              tunnel: [w390] -> w387
              stop <- w393 stop-if-true
              n280 = local read "齿条扭矩(Nm)"() -> (w389:dbl)
              n281 = call <userlib>:"Acm_AxGetCmdVelocity.vi"("AxisHandle"=w390) -> ("Velocity"=w396:dbl)  [unwired: 1 in, 3 out]
              n282 = Wait Until Next ms Multiple(millisecond multiple=u32 50 ("毫秒倍数")) -> ()  [unwired: 1 out]
              n283 = Equal To 0?(x=w396) -> (x = 0?=w394:bool)
              n284 = Greater Or Equal?(x=w389, y=3.0) -> (x >= y?=w391:bool)
              n285 = Or(x=w394, y=w391) -> (x .or. y?=w393:bool)
            }
          }
          frame #19 {
            n286 = while {
              tunnel: w397 -> [w401]
              tunnel: [w400] -> _
              stop <- w399 stop-if-true
              n287 = call "PCI1220U停止.vi"("AxisHandle IN"=w401) -> ("完成"=w399:bool, "AxisHandle OUT"=w400:u32)  [unwired: 9 in]
              n288 = Wait (ms)(milliseconds to wait=u32 50 ("毫秒倍数")) -> ()  [unwired: 1 out]
            }
          }
          frame #20 {
            n289 = local write "旋转齿条轴使能"(FALSE ("旋转齿条轴使能")) -> ()
            n290 = Wait (ms)(milliseconds to wait=u32 500 ("毫秒倍数")) -> ()  [unwired: 1 out]
          }
          frame #21 {
            n291 = local write "工步号"(u32 25 ("工步号")) -> ()
          }
        }
      }
      frame 25 {
        n292 = flat-sequence {
          frame #0 {
            n293 = local read "中间间隙标准(mm)"() -> (w406:dbl)
            n294 = local read "最小间隙(mm)"() -> (w405:dbl)
            n295 = local read "中间位置间隙"() -> (w407:dbl)
            n296 = In Range and Coerce(upper limit=w406, x=w407, lower limit=w405) -> (In Range?=w410:bool)  [unwired: 1 out]
            n297 = case shown="假" w410 {
              tunnel: [FALSE ("本序合格") TRUE ("本序合格")] -> w409
              tunnel: [w415 0.0 ("需调整角度(度)")] -> w408
              tunnel: w407 -> [w413 _]
              tunnel: w406 -> [w412 _]
              tunnel: w405 -> [w411 _]
              frame False {
                n298 = xnode "公式"("X"=w413, "Xmax"=w412, "Xmin"=w411) -> ("结果"=w415:dbl)  [unwired: 1 in, 1 out]
              }
              frame True {
              }
            }
            n299 = local write "单点间隙合格"(w409) -> ()
            n300 = local write "需调整角度(度)"(w408) -> ()
          }
          frame #1 {
            n301 = local read "单点间隙合格"() -> (w430:bool)
            n302 = case shown="假" w430 {
              frame False {
                n303 = local read "已调试次数"() -> (w433:dbl)
                n304 = Less?(x=w433, y="设定间隙调整次数") -> (x < y?=w432:bool)
                n305 = case shown="真" w432 {
                  frame False {
                    n306 = local write "工步号"(u32 45 ("变更工步号")) -> ()
                  }
                  frame True {
                    n307 = local write "工步号"(u32 30 ("变更工步号")) -> ()
                  }
                }
              }
              frame True {
                n308 = local write "工步号"(u32 40 ("变更工步号")) -> ()
              }
            }
          }
        }
      }
      frame 30 {
        # "人工调整"
        n309 = flat-sequence {
          tunnel: [w439] -> w437
          tunnel: w437 -> [w446]
          frame #0 {
            n310 = local write "测头机构轴速度(mm/s)"(30.0 ("测头机构轴速度(mm/s)")) -> ()
          }
          frame #1 {
            n311 = local read "测头机构电机"() -> (w440:u32)
            n312 = while {
              tunnel: w440 -> [w443]
              tunnel: [w442] -> w439
              stop <- w445 stop-if-true
              n313 = local read "测头机构轴待检位"() -> (w441:dbl)
              n314 = call "PCI1220U进给轴位置模式.vi"("Distance"=w441, "AxisHandle IN"=w443) -> ("AbsSuccess"=w445:bool, "AxisHandle OUT"=w442:u32)  [unwired: 8 in]
              n315 = Wait Until Next ms Multiple(millisecond multiple=u32 50 ("毫秒倍数")) -> ()  [unwired: 1 out]
            }
          }
          frame #2 {
            n316 = while {
              tunnel: w446 -> [w450]
              stop <- w448 stop-if-true
              n317 = call <userlib>:"Acm_AxGetCmdVelocity.vi"("AxisHandle"=w450) -> ("Velocity"=w449:dbl)  [unwired: 1 in, 3 out]
              n318 = Wait Until Next ms Multiple(millisecond multiple=u32 50 ("毫秒倍数")) -> ()  [unwired: 1 out]
              n319 = Equal To 0?(x=w449) -> (x = 0?=w448:bool)
            }
          }
          frame #3 {
            n320 = while {
              stop <- w452 stop-if-true
              n321 = local read "测头机构轴位置(mm)"() -> (w454:dbl)
              n322 = Wait Until Next ms Multiple(millisecond multiple=u32 50 ("毫秒倍数")) -> ()  [unwired: 1 out]
              n323 = Less Or Equal?(x=w454, y=35.0) -> (x <= y?=w452:bool)
            }
          }
          frame #4 {
            n324 = local write "测头气缸左移"(TRUE ("测头气缸左移")) -> ()
            n325 = local write "测头气缸右移"(FALSE ("测头气缸右移")) -> ()
          }
          frame #5 {
            n326 = while {
              stop <- w457 stop-if-true
              # "等待启动"
              n327 = local read "间隙启动"() -> (w457:bool)
              n328 = Wait Until Next ms Multiple(millisecond multiple=u32 50 ("毫秒倍数")) -> ()  [unwired: 1 out]
            }
          }
          frame #6 {
            n329 = local read "不合格品"() -> (w459:bool)
            n330 = case shown="假" w459 {
              frame False {
                n331 = flat-sequence {
                  frame #0 {
                    n332 = local read "已调试次数"() -> (w462:dbl)
                    n333 = local write "测头气缸左移"(FALSE ("测头气缸左移")) -> ()
                    n334 = local write "测头气缸右移"(TRUE ("测头气缸左移")) -> ()
                    n335 = Add(x=w462, y=1.0 ("已调试次数")) -> (x+y=w464:dbl)
                    n336 = local write "已调试次数"(w464) -> ()
                  }
                  frame #1 {
                    n337 = while {
                      stop <- w465 stop-if-true
                      n338 = Wait Until Next ms Multiple(millisecond multiple=u32 50 ("毫秒倍数")) -> ()  [unwired: 1 out]
                      n339 = local read "测头右位"() -> (w465:bool)
                    }
                  }
                  frame #2 {
                    n340 = local write "工步号"(u32 20 ("工步号")) -> ()
                  }
                }
              }
              frame True {
                n341 = local write "工步号"(u32 45 ("工步号")) -> ()
              }
            }
          }
        }
      }
      frame 40 {
        n342 = flat-sequence {
          tunnel: [w638] -> w634
          tunnel: w634 -> [w640]
          tunnel: [w639] -> w553
          tunnel: w553 -> [w646]
          tunnel: [w646] -> w552
          tunnel: w552 -> [w657]
          tunnel: [w657] -> w555
          tunnel: w555 -> [w658]
          tunnel: [w659] -> w554
          tunnel: w554 -> [w665]
          tunnel: [w665] -> w630
          tunnel: w630 -> [w674]
          tunnel: [w674] -> w629
          tunnel: w629 -> [w681]
          tunnel: [w681] -> w632
          tunnel: w632 -> [w683]
          tunnel: [w684] -> w551
          tunnel: [w682] -> w549
          tunnel: w551 -> [w693]
          tunnel: [w693] -> w550
          tunnel: w549 -> [w694]
          tunnel: [w694] -> w548
          tunnel: [w692] -> w545
          tunnel: [w691] -> w542
          tunnel: [w690] -> w539
          tunnel: w550 -> [w733]
          tunnel: [w733] -> w557
          tunnel: w548 -> [w732]
          tunnel: [w732] -> w556
          tunnel: [w730] -> w546
          tunnel: w545 -> [w730]
          tunnel: [w729] -> w543
          tunnel: w542 -> [w729]
          tunnel: [w728] -> w540
          tunnel: w539 -> [w728]
          tunnel: w557 -> [w739]
          tunnel: [w739] -> w559
          tunnel: w556 -> [w735]
          tunnel: [w734] -> w558
          tunnel: [w738] -> w547
          tunnel: w546 -> [w738]
          tunnel: [w737] -> w544
          tunnel: w543 -> [w737]
          tunnel: [w736] -> w541
          tunnel: w540 -> [w736]
          tunnel: [w753] -> w480
          tunnel: [w752] -> w478
          tunnel: [w751] -> w476
          tunnel: w559 -> [w750]
          tunnel: [w750] -> w474
          tunnel: [w749] -> w472
          tunnel: w558 -> [w748]
          tunnel: w547 -> [w747]
          tunnel: w544 -> [w746]
          tunnel: w541 -> [w745]
          tunnel: w480 -> [w791]
          tunnel: [w791] -> w479
          tunnel: w478 -> [w786]
          tunnel: [w786] -> w477
          tunnel: w476 -> [w790]
          tunnel: [w790] -> w475
          tunnel: w474 -> [w789]
          tunnel: [w789] -> w473
          tunnel: w472 -> [w788]
          tunnel: [w788] -> w471
          tunnel: [w787] -> w470
          tunnel: [w786] -> w469
          tunnel: w479 -> [w803]
          tunnel: [w803] -> w609
          tunnel: w477 -> [w808]
          tunnel: [w808] -> w607
          tunnel: w475 -> [w806]
          tunnel: [w806] -> w605
          tunnel: w473 -> [w807]
          tunnel: [w807] -> w603
          tunnel: [w805] -> w601
          tunnel: w471 -> [w805]
          tunnel: [w795] -> w599
          tunnel: [w797] -> w597
          tunnel: [w804] -> w595
          tunnel: [w798] -> w593
          tunnel: [w802] -> w591
          tunnel: [w801] -> w589
          tunnel: [w799] -> w588
          tunnel: [w800] -> w587
          tunnel: [w796] -> w564
          tunnel: w470 -> [w795]
          tunnel: w469 -> [w794]
          tunnel: w609 -> [w832]
          tunnel: [w832] -> w608
          tunnel: w607 -> [w831]
          tunnel: [w831] -> w606
          tunnel: w605 -> [w830]
          tunnel: [w830] -> w604
          tunnel: w603 -> [w829]
          tunnel: [w829] -> w602
          tunnel: w601 -> [w828]
          tunnel: [w828] -> w600
          tunnel: w599 -> [w827]
          tunnel: [w827] -> w598
          tunnel: w597 -> [w826]
          tunnel: [w826] -> w596
          tunnel: w595 -> [w825]
          tunnel: [w825] -> w594
          tunnel: w593 -> [w824]
          tunnel: [w824] -> w592
          tunnel: w591 -> [w823]
          tunnel: [w823] -> w590
          tunnel: w589 -> [w818]
          tunnel: w588 -> [w820]
          tunnel: w587 -> [w819]
          tunnel: w564 -> [w817]
          tunnel: [w815] -> w498
          tunnel: [w814] -> w481
          tunnel: w608 -> [w851]
          tunnel: [w851] -> w534
          tunnel: w606 -> [w850]
          tunnel: [w850] -> w533
          tunnel: w604 -> [w849]
          tunnel: [w849] -> w532
          tunnel: w602 -> [w848]
          tunnel: [w848] -> w531
          tunnel: [w847] -> w530
          tunnel: w600 -> [w847]
          tunnel: [w846] -> w529
          tunnel: w598 -> [w846]
          tunnel: w596 -> [w842]
          tunnel: w594 -> [w845]
          tunnel: w592 -> [w843]
          tunnel: w590 -> [w844]
          tunnel: [w844] -> w528
          tunnel: [w836] -> w527
          tunnel: [w835] -> w526
          tunnel: w498 -> [w834]
          tunnel: [w834] -> w497
          tunnel: [w833] -> w482
          tunnel: w481 -> [w833]
          tunnel: w534 -> [w866]
          tunnel: w533 -> [w865]
          tunnel: w532 -> [w864]
          tunnel: w531 -> [w859]
          tunnel: w530 -> [w863]
          tunnel: w529 -> [w870]
          tunnel: [w870] -> w525
          tunnel: w528 -> [w869]
          tunnel: [w869] -> w523
          tunnel: w527 -> [w868]
          tunnel: [w868] -> w521
          tunnel: w526 -> [w867]
          tunnel: [w867] -> w519
          tunnel: [w862] -> w516
          tunnel: [w861] -> w513
          tunnel: [w860] -> w510
          tunnel: [w859] -> w507
          tunnel: [w858] -> w503
          tunnel: w497 -> [w857]
          tunnel: [w857] -> w496
          tunnel: [w856] -> w483
          tunnel: w482 -> [w856]
          tunnel: w525 -> [w916]
          tunnel: [w916] -> w524
          tunnel: w523 -> [w915]
          tunnel: [w915] -> w522
          tunnel: w521 -> [w914]
          tunnel: [w914] -> w520
          tunnel: w519 -> [w913]
          tunnel: [w913] -> w518
          tunnel: [w911] -> w517
          tunnel: w516 -> [w911]
          tunnel: [w910] -> w514
          tunnel: w513 -> [w910]
          tunnel: [w909] -> w511
          tunnel: w510 -> [w909]
          tunnel: [w908] -> w508
          tunnel: w507 -> [w908]
          tunnel: [w907] -> w504
          tunnel: w503 -> [w907]
          tunnel: w496 -> [w906]
          tunnel: [w906] -> w495
          tunnel: [w905] -> w484
          tunnel: w483 -> [w905]
          tunnel: w524 -> [w927]
          tunnel: [w927] -> w538
          tunnel: w522 -> [w926]
          tunnel: [w926] -> w537
          tunnel: w520 -> [w925]
          tunnel: [w925] -> w536
          tunnel: w518 -> [w924]
          tunnel: [w924] -> w535
          tunnel: w517 -> [w921]
          tunnel: [w923] -> w515
          tunnel: w514 -> [w923]
          tunnel: [w922] -> w512
          tunnel: w511 -> [w922]
          tunnel: [w921] -> w509
          tunnel: w508 -> [w920]
          tunnel: [w920] -> w506
          tunnel: [w919] -> w505
          tunnel: w504 -> [w919]
          tunnel: w495 -> [w918]
          tunnel: [w918] -> w494
          tunnel: [w917] -> w485
          tunnel: w484 -> [w917]
          tunnel: [w946] -> w628
          tunnel: [w945] -> w627
          tunnel: [w944] -> w625
          tunnel: w538 -> [w942]
          tunnel: [w943] -> w623
          tunnel: [w942] -> w621
          tunnel: w537 -> [w941]
          tunnel: [w941] -> w612
          tunnel: w536 -> [w940]
          tunnel: w535 -> [w939]
          tunnel: [w940] -> w577
          tunnel: [w939] -> w576
          tunnel: w515 -> [w938]
          tunnel: w512 -> [w937]
          tunnel: w509 -> [w936]
          tunnel: w506 -> [w935]
          tunnel: w505 -> [w934]
          tunnel: w494 -> [w933]
          tunnel: [w933] -> w493
          tunnel: [w932] -> w486
          tunnel: w485 -> [w932]
          tunnel: w628 -> [w986]
          tunnel: w627 -> [w994]
          tunnel: [w994] -> w626
          tunnel: w625 -> [w991]
          tunnel: [w991] -> w624
          tunnel: w623 -> [w993]
          tunnel: [w993] -> w622
          tunnel: w621 -> [w992]
          tunnel: [w992] -> w620
          tunnel: [w988] -> w614
          tunnel: [w987] -> w613
          tunnel: w612 -> [w985]
          tunnel: [w986] -> w611
          tunnel: [w985] -> w610
          tunnel: w577 -> [w984]
          tunnel: w576 -> [w983]
          tunnel: [w984] -> w572
          tunnel: [w983] -> w569
          tunnel: w493 -> [w982]
          tunnel: [w982] -> w492
          tunnel: [w981] -> w487
          tunnel: w486 -> [w981]
          tunnel: w626 -> [w1000]
          tunnel: [w1044] -> w633
          tunnel: w624 -> [w1044]
          tunnel: w622 -> [w1043]
          tunnel: w620 -> [w999]
          tunnel: [w1042] -> w619
          tunnel: w614 -> [w1041]
          tunnel: w613 -> [w1040]
          tunnel: w611 -> [w1024]
          tunnel: w610 -> [w1023]
          tunnel: [w1032] -> w586
          tunnel: [w1031] -> w575
          tunnel: [w1030] -> w573
          tunnel: w572 -> [w1030]
          tunnel: [w1029] -> w570
          tunnel: w569 -> [w1029]
          tunnel: [w1028] -> w567
          tunnel: [w1027] -> w565
          tunnel: [w1010] -> w562
          tunnel: [w1011] -> w560
          tunnel: [w1009] -> w502
          tunnel: [w1008] -> w500
          tunnel: w492 -> [w1006]
          tunnel: [w1006] -> w491
          tunnel: [w1005] -> w488
          tunnel: w487 -> [w1005]
          tunnel: w633 -> [w1069]
          tunnel: [w1069] -> w585
          tunnel: [w1065] -> w583
          tunnel: w619 -> [w1067]
          tunnel: [w1064] -> w581
          tunnel: w586 -> [w1063]
          tunnel: [w1051] -> w579
          tunnel: [w1061] -> w578
          tunnel: w575 -> [w1060]
          tunnel: [w1055] -> w574
          tunnel: w573 -> [w1055]
          tunnel: [w1054] -> w571
          tunnel: w570 -> [w1054]
          tunnel: [w1053] -> w568
          tunnel: w567 -> [w1053]
          tunnel: [w1052] -> w566
          tunnel: w565 -> [w1052]
          tunnel: [w1050] -> w563
          tunnel: w562 -> [w1050]
          tunnel: [w1049] -> w561
          tunnel: w560 -> [w1049]
          tunnel: w502 -> [w1048]
          tunnel: [w1048] -> w501
          tunnel: w500 -> [w1047]
          tunnel: [w1047] -> w499
          tunnel: w491 -> [w1046]
          tunnel: [w1046] -> w490
          tunnel: [w1045] -> w489
          tunnel: w488 -> [w1045]
          tunnel: w585 -> [w1086]
          tunnel: [w1086] -> w584
          tunnel: w583 -> [w1085]
          tunnel: [w1085] -> w582
          tunnel: w581 -> [w1084]
          tunnel: [w1084] -> w580
          tunnel: w579 -> [w1080]
          tunnel: w578 -> [w1076]
          tunnel: w574 -> [w1079]
          tunnel: w571 -> [w1078]
          tunnel: w568 -> [w1082]
          tunnel: w566 -> [w1081]
          tunnel: w563 -> [w1075]
          tunnel: w561 -> [w1074]
          tunnel: w501 -> [w1073]
          tunnel: w499 -> [w1072]
          tunnel: w490 -> [w1071]
          tunnel: w489 -> [w1070]
          tunnel: w584 -> [w1090]
          tunnel: [w1089] -> w631
          tunnel: w582 -> [w1088]
          tunnel: [w1087] -> w615
          tunnel: w580 -> [w1087]
          tunnel: w631 -> [w1097]
          tunnel: [w1097] -> w618
          tunnel: [w1096] -> w616
          tunnel: w615 -> [w1096]
          tunnel: w618 -> [w1104]
          tunnel: [w1103] -> w617
          tunnel: w616 -> [w1102]
          tunnel: w617 -> [w1110]
          frame #0 {
            n343 = local write "电动缸速度(mm/s)"(15.0 ("电动缸速度(mm/s)")) -> ()
            n344 = local write "已调试次数"(0.0 ("已调试次数")) -> ()
            n345 = local write "选项卡控件"(T1."轴向力测量" ("选项卡控件")) -> ()
            n346 = local read "电动缸电机"() -> (w638:u32)
          }
          frame #1 {
            n347 = while {
              tunnel: w640 -> [w645]
              tunnel: [w644] -> w639
              stop <- w643 stop-if-true
              n348 = local read "齿条左极限"() -> (w641:dbl)
              n349 = Wait (ms)(milliseconds to wait=u32 50 ("毫秒倍数")) -> ()  [unwired: 1 out]
              n350 = call "PCI1240电动缸位置模式 .vi"("Distance"=w641, "AxisHandle IN"=w645) -> ("AbsSuccess"=w643:bool, "AxisHandle OUT"=w644:u32)  [unwired: 8 in]
            }
          }
          frame #2 {
            n351 = while {
              tunnel: w646 -> [w654]
              stop <- w647 stop-if-true
              n352 = local read "齿条推拉力(N)"() -> (w651:dbl)
              n353 = call <userlib>:"Acm_AxGetCmdVelocity.vi"("AxisHandle"=w654) -> ("Velocity"=w653:dbl)  [unwired: 1 in, 3 out]
              n354 = Wait (ms)(milliseconds to wait=u32 50 ("毫秒倍数")) -> ()  [unwired: 1 out]
              n355 = Equal To 0?(x=w653) -> (x = 0?=w649:bool)
              n356 = Less Or Equal?(x=w651, y=-500.0) -> (x <= y?=w648:bool)
              n357 = Or ("或")(x=w649, y=w648) -> (x .or. y?=w647:bool)
            }
          }
          frame #3 {
            n358 = local write "电动缸速度(mm/s)"(1.0 ("电动缸速度(mm/s)")) -> ()
            n359 = Wait Until Next ms Multiple(millisecond multiple=50 ("毫秒倍数")) -> ()  [unwired: 1 out]
          }
          frame #4 {
            n360 = while {
              tunnel: [w663] -> w659
              tunnel: w658 -> [w662]
              stop <- w664 stop-if-true
              n361 = Wait (ms)(milliseconds to wait=u32 50 ("毫秒倍数")) -> ()  [unwired: 1 out]
              n362 = call "PCI1240电动缸位置模式 .vi"("Distance"=118.0, "AxisHandle IN"=w662) -> ("AbsSuccess"=w664:bool, "AxisHandle OUT"=w663:u32)  [unwired: 8 in]
            }
          }
          frame #5 {
            n363 = while {
              tunnel: w665 -> [w673]
              stop <- w666 stop-if-true
              n364 = local read "齿条推拉力(N)"() -> (w670:dbl)
              n365 = call <userlib>:"Acm_AxGetCmdVelocity.vi"("AxisHandle"=w673) -> ("Velocity"=w672:dbl)  [unwired: 1 in, 3 out]
              n366 = Wait (ms)(milliseconds to wait=u32 50 ("毫秒倍数")) -> ()  [unwired: 1 out]
              n367 = Equal To 0?(x=w672) -> (x = 0?=w668:bool)
              n368 = Less Or Equal?(x=w670, y=-500.0) -> (x <= y?=w667:bool)
              n369 = Or ("或")(x=w668, y=w667) -> (x .or. y?=w666:bool)
            }
          }
          frame #6 {
            n370 = while {
              tunnel: w674 -> [w678]
              tunnel: [w677] -> _
              stop <- w676 stop-if-true
              n371 = call "PCI1220U停止.vi"("AxisHandle IN"=w678) -> ("完成"=w676:bool, "AxisHandle OUT"=w677:u32)  [unwired: 9 in]
              n372 = Wait (ms)(milliseconds to wait=u32 50 ("毫秒倍数")) -> ()  [unwired: 1 out]
            }
          }
          frame #7 {
            n373 = Wait Until Next ms Multiple(millisecond multiple=u32 50 ("毫秒倍数")) -> ()  [unwired: 1 out]
            n374 = local write "电动缸速度(mm/s)"(5.0 ("电动缸速度(mm/s)")) -> ()
          }
          frame #8 {
            n375 = while {
              tunnel: w683 -> [w689]
              tunnel: [w686] -> w682
              stop <- w687 stop-if-true
              n376 = local read "齿条右极限"() -> (w685:dbl)
              n377 = Wait (ms)(milliseconds to wait=u32 50 ("毫秒倍数")) -> ()  [unwired: 1 out]
              n378 = call "PCI1240电动缸位置模式 .vi"("Distance"=w685, "AxisHandle IN"=w689) -> ("AbsSuccess"=w687:bool, "AxisHandle OUT"=w686:u32)  [unwired: 8 in]
            }
            n379 = local read "转向器中心"() -> (w684:dbl)
          }
          frame #9 {
            w695 = dbl[] []
            n380 = while {
              shift-right: [w716] -> w691
              shift-left: w695 -> [w726]
              shift-right: [w724] -> w692
              shift-left: w695 -> [w725]
              tunnel: w694 -> [w721]
              tunnel: [w721] -> _
              tunnel: w693 -> [w719]
              shift-right: [w715] -> w690
              shift-left: w695 -> [w717]
              stop <- w709 stop-if-true
              n381 = local read "中间位置间隙"() -> (w706:dbl)
              n382 = local read "基准位移"() -> (w722:dbl)
              n383 = local read "间隙位移(mm)"() -> (w705:dbl)
              n384 = call <userlib>:"Acm_AxGetCmdVelocity.vi"("AxisHandle"=w721) -> ("Velocity"=w714:dbl)  [unwired: 1 in, 3 out]
              n385 = Wait (ms)(milliseconds to wait=u32 50 ("毫秒倍数")) -> ()  [unwired: 1 out]
              n386 = local read "齿条推拉力(N)"() -> (w712:dbl)
              n387 = call "PCI1240电动缸读取位置.vi"("AxisHandle IN"=w721) -> ("位置"=w720:dbl)  [unwired: 9 in, 1 out]
              n388 = Subtract(x=w705, y=w722) -> (x-y=w708:dbl)
              n389 = Subtract(x=w720, y=w719) -> (x-y=w699:dbl)
              n390 = Add(x=w708, y=w706) -> (x+y=w707:dbl)
              n391 = Multiply(x=w699, y=1.0) -> (x*y=w697:dbl)
              n392 = Build Array (concatenate) ("创建数组")(w725, w707) -> (w724:dbl[])
              n393 = Build Array (concatenate) ("创建数组")(w726, w697) -> (w716:dbl[])
              n394 = Build Array (concatenate) ("创建数组")(w717, w712) -> (w715:dbl[])
              n395 = Greater Or Equal?(x=w712, y=500.0) -> (x >= y?=w710:bool)
              n396 = Less Or Equal?(x=w705, y=0.0) -> (x <= y?=w704:bool)
              n397 = Greater Or Equal?(x=w705, y=4.0) -> (x >= y?=w703:bool)
              n398 = Equal To 0?(x=w714) -> (x = 0?=w711:bool)
              n399 = Or(x=w703, y=w704) -> (x .or. y?=w702:bool)
              n400 = Bundle ("捆绑")(w716, w724) -> (w696:cluster{dbl[], dbl[]})  [unwired: 1 in]
              n401 = Or(x=w711, y=w710) -> (x .or. y?=w709:bool)
              n402 = Bundle ("捆绑")(w716, w715) -> (w718:cluster{dbl[], dbl[]})  [unwired: 1 in]
              n403 = property on="间隙位移(mm)" class="DigNum (严格)"("Blinking"=w702) -> ()  [unwired: 2 in, 2 out]
              n404 = Build Array ("创建数组")(w696, w718) -> (w723:cluster{dbl[], dbl[]}[])
              n405 = local write "行程跳动曲线"(w723) -> ()
            }
          }
          frame #10 {
            n406 = local write "电动缸速度(mm/s)"(1.0 ("电动缸速度(mm/s)")) -> ()
          }
          frame #11 {
            n407 = while {
              tunnel: w735 -> [w742]
              tunnel: [w741] -> w734
              stop <- w744 stop-if-true
              n408 = Wait Until Next ms Multiple(millisecond multiple=u32 50 ("毫秒倍数")) -> ()  [unwired: 1 out]
              n409 = call "PCI1240电动缸位置模式 .vi"("Distance"=-50.0, "AxisHandle IN"=w742) -> ("AbsSuccess"=w744:bool, "AxisHandle OUT"=w741:u32)  [unwired: 8 in]
            }
          }
          frame #12 {
            n410 = while {
              shift-right: [w774] -> w752
              shift-left: w746 -> [w784]
              shift-right: [w782] -> w753
              shift-left: w747 -> [w783]
              tunnel: w748 -> [w779]
              tunnel: [w779] -> w751
              tunnel: w750 -> [w777]
              shift-right: [w773] -> w749
              shift-left: w745 -> [w775]
              stop <- w767 stop-if-true
              n411 = local read "中间位置间隙"() -> (w764:dbl)
              n412 = local read "基准位移"() -> (w780:dbl)
              n413 = local read "间隙位移(mm)"() -> (w763:dbl)
              n414 = call <userlib>:"Acm_AxGetCmdVelocity.vi"("AxisHandle"=w779) -> ("Velocity"=w772:dbl)  [unwired: 1 in, 3 out]
              n415 = Wait (ms)(milliseconds to wait=u32 45 ("毫秒倍数")) -> ()  [unwired: 1 out]
              n416 = local read "齿条推拉力(N)"() -> (w770:dbl)
              n417 = call "PCI1240电动缸读取位置.vi"("AxisHandle IN"=w779) -> ("位置"=w778:dbl)  [unwired: 9 in, 1 out]
              n418 = Subtract(x=w763, y=w780) -> (x-y=w766:dbl)
              n419 = Subtract(x=w778, y=w777) -> (x-y=w757:dbl)
              n420 = Add(x=w766, y=w764) -> (x+y=w765:dbl)
              n421 = Multiply(x=w757, y=1.0) -> (x*y=w755:dbl)
              n422 = Build Array (concatenate) ("创建数组")(w783, w765) -> (w782:dbl[])
              n423 = Build Array (concatenate) ("创建数组")(w784, w755) -> (w774:dbl[])
              n424 = Build Array (concatenate) ("创建数组")(w775, w770) -> (w773:dbl[])
              n425 = Greater Or Equal?(x=w770, y=500.0) -> (x >= y?=w768:bool)
              n426 = Less Or Equal?(x=w763, y=0.0) -> (x <= y?=w762:bool)
              n427 = Greater Or Equal?(x=w763, y=4.0) -> (x >= y?=w761:bool)
              n428 = Equal To 0?(x=w772) -> (x = 0?=w769:bool)
              n429 = Or(x=w761, y=w762) -> (x .or. y?=w760:bool)
              n430 = Bundle ("捆绑")(w774, w782) -> (w754:cluster{dbl[], dbl[]})  [unwired: 1 in]
              n431 = Or(x=w769, y=w768) -> (x .or. y?=w767:bool)
              n432 = Bundle ("捆绑")(w774, w773) -> (w776:cluster{dbl[], dbl[]})  [unwired: 1 in]
              n433 = property on="间隙位移(mm)" class="DigNum (严格)"("Blinking"=w760) -> ()  [unwired: 2 in, 2 out]
              n434 = Build Array ("创建数组")(w754, w776) -> (w781:cluster{dbl[], dbl[]}[])
              n435 = local write "行程跳动曲线"(w781) -> ()
            }
          }
          frame #13 {
            n436 = Array Size(array=w788) -> (size(s)=w787:i32)
          }
          frame #14 {
            n437 = while {
              tunnel: w806 -> [w813]
              tunnel: [w812] -> _
              stop <- w811 stop-if-true
              n438 = call "PCI1220U停止.vi"("AxisHandle IN"=w813) -> ("完成"=w811:bool, "AxisHandle OUT"=w812:u32)  [unwired: 9 in]
              n439 = Wait (ms)(milliseconds to wait=u32 50 ("毫秒倍数")) -> ()  [unwired: 1 out]
            }
            n440 = call "间隙计算.vi"("扭矩数组"=w803) -> ("峰值间隙1"=w799:dbl, "峰值间隙2"=w800:dbl)  [unwired: 6 in, 3 out]
            n441 = call "功能计算_何 截取位移左.vi"("位移数组"=w794, "拉压力数组"=w805, "半行程"="半行程", "截取百分比"="截取百分比") -> ("峰值扭矩"=w797:dbl, "平均扭矩"=w804:dbl, "扭差"=w798:dbl)  [unwired: 12 in, 1 out]
            n442 = Array Size(array=w803) -> (size(s)=w802:i32)
            n443 = disable-structure shown="禁用" {
              frame Disabled {
                n444 = Wait Until Next ms Multiple(millisecond multiple=u32 500 ("毫秒倍数")) -> ()  [unwired: 1 out]
              }
              frame Enabled {
              }
            }
            n445 = local read "全行程180°外间隙标准(mm)"() -> (w796:dbl)
            n446 = local read "全行程180°内间隙标准(mm)"() -> (w801:dbl)
            n447 = local write "左180°内全行程间隙"(w799) -> ()
            n448 = local write "左180°外全行程间隙"(w800) -> ()
            n449 = local write "左最大轴向力(N)"(w797) -> ()
            n450 = local write "左平均轴向力(N)"(w804) -> ()
            n451 = local write "左轴向力波动(N)"(w798) -> ()
          }
          frame #15 {
            n452 = Less?(x=w819, y=w817) -> (x < y?=w821:bool)
            n453 = Less?(x=w820, y=w818) -> (x < y?=w822:bool)
            n454 = Not(x=w821) -> (.not. x?=w814:bool)
            n455 = local write "电动缸速度(mm/s)"(5.0 ("电动缸速度(mm/s)")) -> ()
            n456 = Not(x=w822) -> (.not. x?=w815:bool)
            n457 = property on="左180°外全行程间隙" class="DigNum (严格)"("Blinking"=w814) -> ()  [unwired: 2 in, 2 out]
            n458 = property on="左180°内全行程间隙" class="DigNum (严格)"("Blinking"=w815) -> ()  [unwired: 2 in, 2 out]
          }
          frame #16 {
            n459 = local read "最大轴向力标准(N)"() -> (w840:dbl)
            n460 = while {
              tunnel: w849 -> [w855]
              tunnel: w848 -> [_]
              stop <- w854 stop-if-true
              n461 = local read "齿条左极限"() -> (w852:dbl)
              n462 = Wait Until Next ms Multiple(millisecond multiple=u32 50 ("毫秒倍数")) -> ()  [unwired: 1 out]
              n463 = call "PCI1240电动缸位置模式 .vi"("Distance"=w852, "AxisHandle IN"=w855) -> ("AbsSuccess"=w854:bool)  [unwired: 8 in, 1 out]
            }
            n464 = local read "轴向力标准(N)"() -> (w839:dbl)
            n465 = local read "平均轴向力MAX(N)"() -> (w838:dbl)
            n466 = local read "力波动标准(N)"() -> (w837:dbl)
            n467 = call "判断.vi"("y 3"=w837, "y2-2"=w838, "y2-1"=w839, "y"=w840, "x 3"=w843, "x 2"=w845, "x"=w842) -> ("非x? 3"=w835:bool, "非x? 2"=w841:bool, "非x?"=w836:bool)  [unwired: 2 in]
            n468 = property on="左最大轴向力(N)" class="DigNum (严格)"("Blinking"=w836) -> ()  [unwired: 2 in, 2 out]
            n469 = property on="左轴向力波动(N)" class="DigNum (严格)"("Blinking"=w835) -> ()  [unwired: 2 in, 2 out]
            n470 = property on="左平均轴向力(N)" class="DigNum (严格)"("Blinking"=w841) -> ()  [unwired: 2 in, 2 out]
          }
          frame #17 {
            n471 = while {
              shift-right: [w875] -> w860
              shift-left: w865 -> [w903]
              shift-right: [w901] -> w861
              shift-left: w866 -> [w902]
              tunnel: w864 -> [w898]
              tunnel: [w898] -> w862
              tunnel: w859 -> [w897]
              shift-right: [w894] -> w858
              shift-left: w863 -> [w895]
              stop <- w889 stop-if-true
              n472 = local read "间隙位移(mm)"() -> (w881:dbl)
              n473 = call <userlib>:"Acm_AxGetCmdVelocity.vi"("AxisHandle"=w898) -> ("Velocity"=w887:dbl)  [unwired: 1 in, 3 out]
              n474 = local read "基准位移"() -> (w899:dbl)
              n475 = Wait (ms)(milliseconds to wait=u32 50 ("毫秒倍数")) -> ()  [unwired: 1 out]
              n476 = local read "中间位置间隙"() -> (w886:dbl)
              n477 = local read "齿条推拉力(N)"() -> (w893:dbl)
              n478 = call "PCI1240电动缸读取位置.vi"("AxisHandle IN"=w898) -> ("位置"=w873:dbl)  [unwired: 9 in, 1 out]
              n479 = Subtract(x=w881, y=w899) -> (x-y=w900:dbl)
              n480 = Subtract(x=w873, y=2.7) -> (x-y=w871:dbl)
              n481 = Subtract(x=w871, y=w897) -> (x-y=w879:dbl)
              n482 = Add(x=w900, y=w886) -> (x+y=w888:dbl)
              n483 = Less Or Equal?(x=w893, y=-500.0) -> (x <= y?=w890:bool)
              n484 = Equal To 0?(x=w887) -> (x = 0?=w891:bool)
              n485 = Multiply(x=w879, y=1.0) -> (x*y=w877:dbl)
              n486 = Build Array (concatenate) ("创建数组")(w903, w877) -> (w875:dbl[])
              n487 = Build Array (concatenate) ("创建数组")(w895, w893) -> (w894:dbl[])
              n488 = Build Array (concatenate) ("创建数组")(w902, w888) -> (w901:dbl[])
              n489 = Or(x=w891, y=w890) -> (x .or. y?=w889:bool)
              n490 = Bundle ("捆绑")(w875, w901) -> (w876:cluster{dbl[], dbl[]})  [unwired: 1 in]
              n491 = Bundle ("捆绑")(w875, w894) -> (w896:cluster{dbl[], dbl[]})  [unwired: 1 in]
              n492 = Build Array ("创建数组")(w876, w896) -> (w874:cluster{dbl[], dbl[]}[])
              n493 = Less Or Equal?(x=w881, y=0.0) -> (x <= y?=w885:bool)
              n494 = Greater Or Equal?(x=w881, y=4.0) -> (x >= y?=w884:bool)
              n495 = Or(x=w884, y=w885) -> (x .or. y?=w880:bool)
              n496 = local write "行程跳动曲线"(w874) -> ()
              n497 = property on="间隙位移(mm)" class="DigNum (严格)"("Blinking"=w880) -> ()  [unwired: 2 in, 2 out]
            }
          }
          frame #18 {
            n498 = local write "电动缸速度(mm/s)"(1.0 ("电动缸速度(mm/s)")) -> ()
          }
          frame #19 {
            n499 = while {
              tunnel: w921 -> [w931]
              stop <- w930 stop-if-true
              n500 = Wait Until Next ms Multiple(millisecond multiple=u32 50 ("毫秒倍数")) -> ()  [unwired: 1 out]
              n501 = call "PCI1240电动缸位置模式 .vi"("Distance"=130.0, "AxisHandle IN"=w931) -> ("AbsSuccess"=w930:bool)  [unwired: 8 in, 1 out]
            }
          }
          frame #20 {
            n502 = while {
              shift-right: [w951] -> w945
              shift-left: w937 -> [w979]
              shift-right: [w977] -> w946
              shift-left: w938 -> [w978]
              tunnel: w936 -> [w974]
              tunnel: [w974] -> w944
              tunnel: w935 -> [w973]
              shift-right: [w970] -> w943
              shift-left: w934 -> [w971]
              stop <- w965 stop-if-true
              n503 = local read "间隙位移(mm)"() -> (w957:dbl)
              n504 = call <userlib>:"Acm_AxGetCmdVelocity.vi"("AxisHandle"=w974) -> ("Velocity"=w963:dbl)  [unwired: 1 in, 3 out]
              n505 = local read "基准位移"() -> (w975:dbl)
              n506 = Wait (ms)(milliseconds to wait=u32 45 ("毫秒倍数")) -> ()  [unwired: 1 out]
              n507 = local read "中间位置间隙"() -> (w962:dbl)
              n508 = local read "齿条推拉力(N)"() -> (w969:dbl)
              n509 = call "PCI1240电动缸读取位置.vi"("AxisHandle IN"=w974) -> ("位置"=w949:dbl)  [unwired: 9 in, 1 out]
              n510 = Subtract(x=w957, y=w975) -> (x-y=w976:dbl)
              n511 = Subtract(x=w949, y=2.7) -> (x-y=w947:dbl)
              n512 = Subtract(x=w947, y=w973) -> (x-y=w955:dbl)
              n513 = Add(x=w976, y=w962) -> (x+y=w964:dbl)
              n514 = Multiply(x=w955, y=1.0) -> (x*y=w953:dbl)
              n515 = Less Or Equal?(x=w969, y=-500.0) -> (x <= y?=w966:bool)
              n516 = Build Array (concatenate) ("创建数组")(w979, w953) -> (w951:dbl[])
              n517 = Build Array (concatenate) ("创建数组")(w971, w969) -> (w970:dbl[])
              n518 = Equal To 0?(x=w963) -> (x = 0?=w967:bool)
              n519 = Build Array (concatenate) ("创建数组")(w978, w964) -> (w977:dbl[])
              n520 = Bundle ("捆绑")(w951, w970) -> (w972:cluster{dbl[], dbl[]})  [unwired: 1 in]
              n521 = Or(x=w967, y=w966) -> (x .or. y?=w965:bool)
              n522 = Bundle ("捆绑")(w951, w977) -> (w952:cluster{dbl[], dbl[]})  [unwired: 1 in]
              n523 = Build Array ("创建数组")(w952, w972) -> (w950:cluster{dbl[], dbl[]}[])
              n524 = Less Or Equal?(x=w957, y=0.0) -> (x <= y?=w961:bool)
              n525 = Greater Or Equal?(x=w957, y=4.0) -> (x >= y?=w960:bool)
              n526 = Or(x=w960, y=w961) -> (x .or. y?=w956:bool)
              n527 = local write "行程跳动曲线"(w950) -> ()
              n528 = property on="间隙位移(mm)" class="DigNum (严格)"("Blinking"=w956) -> ()  [unwired: 2 in, 2 out]
            }
          }
          frame #21 {
            n529 = while {
              tunnel: w991 -> [w998]
              tunnel: [w997] -> _
              stop <- w996 stop-if-true
              n530 = call "PCI1220U停止.vi"("AxisHandle IN"=w998) -> ("完成"=w996:bool, "AxisHandle OUT"=w997:u32)  [unwired: 9 in]
              n531 = Wait (ms)(milliseconds to wait=u32 50 ("毫秒倍数")) -> ()  [unwired: 1 out]
            }
            n532 = Array Max & Min(array=w986) -> (max value=w990:dbl, min value=w989:dbl)  [unwired: 2 out]
            n533 = Absolute Value(x=w990) -> (abs(x)=w988:dbl)
            n534 = Absolute Value(x=w989) -> (abs(x)=w987:dbl)
            n535 = local write "右全行程间隙"(w987) -> ()
            n536 = local write "左全行程间隙"(w988) -> ()
          }
          frame #22 {
            (unwired) 46.996 ("y")
            n537 = local read "半行程"() -> (w1003:dbl)
            n538 = local read "全行程180°外间隙标准(mm)"() -> (w1039:dbl)
            n539 = Split 1D Array(array=w1000, index=w999) -> (second subarray=w1001:dbl[])  [unwired: 1 out]
            n540 = local read "截取百分比"() -> (w1002:dbl)
            n541 = local read "全行程180°外间隙标准(mm)"() -> (w1020:dbl)
            n542 = Split 1D Array(array=w1043, index=w999) -> (second subarray=w1004:dbl[])  [unwired: 1 out]
            n543 = local read "全行程180°内间隙标准(mm)"() -> (w1021:dbl)
            n544 = Array Max & Min(array=w1000) -> (max value=w1035:dbl, min value=w1034:dbl)  [unwired: 2 out]
            n545 = local read "总行程标准(mm)"() -> (w1015:dbl)
            n546 = call "功能计算_何 截取位移右.vi"("位移数组"=w1001, "拉压力数组"=w1004, "半行程"=w1003, "截取百分比"=w1002) -> ("峰值扭矩"=w1032:dbl, "平均扭矩"=w1042:dbl, "扭差"=w1031:dbl)  [unwired: 12 in, 1 out]
            n547 = Split 1D Array(array=w1024, index=w1023) -> (second subarray=w1022:dbl[])  [unwired: 1 out]
            n548 = Subtract(x=w1035, y=w1034) -> (x-y=w1026:dbl)
            n549 = Subtract(x=w1026, y="机械间隙值") -> (x-y=w1007:dbl)
            n550 = local write "总行程(mm)"(w1007) -> ()
            n551 = local write "右最大轴向力(N)"(w1032) -> ()
            n552 = Greater?(x=w1041, y=w1039) -> (0:w1028:bool)
            n553 = call "间隙计算.vi"("扭矩数组"=w1022) -> ("峰值间隙1"=w1038:dbl, "峰值间隙2"=w1037:dbl)  [unwired: 6 in, 3 out]
            n554 = Greater?(x=w1040, y=w1039) -> (0:w1027:bool)
            n555 = local write "右轴向力波动(N)"(w1031) -> ()
            n556 = local write "右平均轴向力(N)"(w1042) -> ()
            n557 = local read "总行程最大值"() -> (w1016:dbl)
            n558 = In Range and Coerce "判定范围并强制转换"(upper limit=w1016, x=w1007, lower limit=w1015) -> (In Range?=w1013:bool)  [unwired: 1 out]
            n559 = Less?(x=w1037, y=w1020) -> (x < y?=w1014:bool)
            n560 = Less?(x=w1038, y=w1021) -> (x < y?=w1036:bool)
            n561 = local write "右180°外全行程间隙"(w1037) -> ()
            n562 = local read "总圈数最大值"() -> (w1017:dbl)
            n563 = local write "右180°内全行程间隙"(w1038) -> ()
            n564 = property on="左全行程间隙" class="DigNum (严格)"("Blinking"=w1028) -> ()  [unwired: 2 in, 2 out]
            n565 = property on="右全行程间隙" class="DigNum (严格)"("Blinking"=w1027) -> ()  [unwired: 2 in, 2 out]
            n566 = Divide(x=w1007, y="齿条传动比") -> (x/y=w1019:dbl)
            n567 = Not(x=w1036) -> (.not. x?=w1009:bool)
            n568 = Not(x=w1014) -> (.not. x?=w1008:bool)
            n569 = property on="右180°外全行程间隙" class="DigNum (严格)"("Blinking"=w1008) -> ()  [unwired: 2 in, 2 out]
            n570 = local read "总圈数标准"() -> (w1018:dbl)
            n571 = In Range and Coerce(upper limit=w1017, x=w1019, lower limit=w1018) -> (In Range?=w1012:bool)  [unwired: 1 out]
            n572 = Not(x=w1013) -> (.not. x?=w1011:bool)
            n573 = local write "总圈数"(w1019) -> ()
            n574 = Not(x=w1012) -> (.not. x?=w1010:bool)
            n575 = property on="总行程(mm)" class="DigNum (严格)"("Blinking"=w1011) -> ()  [unwired: 2 in, 2 out]
            n576 = property on="右180°内全行程间隙" class="DigNum (严格)"("Blinking"=w1009) -> ()  [unwired: 2 in, 2 out]
            n577 = property on="总圈数" class="DigNum (严格)"("Blinking"=w1010) -> ()  [unwired: 2 in, 2 out]
            "轴向力X" <- w1000
            "轴向力Y" <- w1043
          }
          frame #23 {
            n578 = local read "最大轴向力标准(N)"() -> (w1059:dbl)
            n579 = local read "转向器中心"() -> (w1064:dbl)
            n580 = local read "平均轴向力MAX(N)"() -> (w1057:dbl)
            n581 = local read "轴向力标准(N)"() -> (w1058:dbl)
            n582 = local read "力波动标准(N)"() -> (w1056:dbl)
            n583 = call "判断.vi"("y 3"=w1056, "y2-2"=w1057, "y2-1"=w1058, "y"=w1059, "x 3"=w1060, "x 2"=w1067, "x"=w1063) -> ("非x? 3"=w1061:bool, "非x? 2"=w1062:bool, "非x?"=w1051:bool)  [unwired: 2 in]
            n584 = local write "电动缸速度(mm/s)"(15.0 ("电动缸速度(mm/s)")) -> ()
            n585 = property on="右最大轴向力(N)" class="DigNum (严格)"("Blinking"=w1051) -> ()  [unwired: 2 in, 2 out]
            n586 = property on="右平均轴向力(N)" class="DigNum (严格)"("Blinking"=w1062) -> ()  [unwired: 2 in, 2 out]
            n587 = Add(x=w1064, y=-10.0) -> (x+y=w1065:dbl)
          }
          frame #24 {
            n588 = Compound Arithmetic op=OR(w1075, w1082, w1081, w1080, w1073, w1072, w1076, w1079, w1078, w1074, w1071, w1070) -> (w1077:bool)
            n589 = property on="右轴向力波动(N)" class="DigNum (严格)"("Blinking"=w1076) -> ()  [unwired: 2 in, 2 out]
            n590 = Not(x=w1077) -> (.not. x?=w1083:bool)
            n591 = local write "全行程间隙及轴向力合格"(w1083) -> ()
          }
          frame #25 {
            n592 = while {
              tunnel: w1090 -> [w1094]
              tunnel: [w1092] -> w1089
              tunnel: w1088 -> [w1091]
              stop <- w1093 stop-if-true
              n593 = call "PCI1240电动缸位置模式 .vi"("Distance"=w1091, "AxisHandle IN"=w1094) -> ("AbsSuccess"=w1093:bool, "AxisHandle OUT"=w1092:u32)  [unwired: 8 in]
              n594 = Wait (ms)(milliseconds to wait=u32 50 ("毫秒倍数")) -> ()  [unwired: 1 out]
            }
          }
          frame #26 {
            n595 = while {
              tunnel: w1097 -> [w1101]
              stop <- w1099 stop-if-true
              n596 = call <userlib>:"Acm_AxGetCmdVelocity.vi"("AxisHandle"=w1101) -> ("Velocity"=w1100:dbl)  [unwired: 1 in, 3 out]
              n597 = Wait Until Next ms Multiple(millisecond multiple=u32 50 ("毫秒倍数")) -> ()  [unwired: 1 out]
              n598 = Equal To 0?(x=w1100) -> (x = 0?=w1099:bool)
            }
          }
          frame #27 {
            n599 = while {
              tunnel: w1104 -> [w1108]
              tunnel: [w1106] -> w1103
              tunnel: w1102 -> [w1105]
              stop <- w1107 stop-if-true
              n600 = call "PCI1240电动缸位置模式 .vi"("Distance"=w1105, "AxisHandle IN"=w1108) -> ("AbsSuccess"=w1107:bool, "AxisHandle OUT"=w1106:u32)  [unwired: 8 in]
              n601 = Wait (ms)(milliseconds to wait=u32 50 ("毫秒倍数")) -> ()  [unwired: 1 out]
            }
          }
          frame #28 {
            n602 = while {
              tunnel: w1110 -> [w1114]
              stop <- w1112 stop-if-true
              n603 = call <userlib>:"Acm_AxGetCmdVelocity.vi"("AxisHandle"=w1114) -> ("Velocity"=w1113:dbl)  [unwired: 1 in, 3 out]
              n604 = Wait Until Next ms Multiple(millisecond multiple=u32 50 ("毫秒倍数")) -> ()  [unwired: 1 out]
              n605 = Equal To 0?(x=w1113) -> (x = 0?=w1112:bool)
            }
          }
          frame #29 {
            n606 = local read "轴向力已做次数"() -> (w1117:dbl)
            n607 = Add(x=w1117, y=1.0) -> (x+y=w1115:dbl)
            n608 = local write "轴向力已做次数"(w1115) -> ()
          }
          frame #30 {
            n609 = local read "全行程间隙及轴向力合格"() -> (w1118:bool)
            n610 = case shown="假" w1118 {
              frame False {
                n611 = Less?(x="轴向力已做次数", y="设定轴向力调整次数") -> (x < y?=w1120:bool)
                n612 = case shown="真" w1120 {
                  frame False {
                    n613 = local write "工步号"(u32 45 ("工步号")) -> ()
                  }
                  frame True {
                    n614 = local write "工步号"(u32 30 ("工步号")) -> ()
                  }
                }
              }
              frame True {
                n615 = local write "工步号"(u32 45 ("工步号")) -> ()
              }
            }
          }
        }
      }
      frame 45 {
        # "测头退回"
        n616 = flat-sequence {
          tunnel: [w1128] -> w1125
          tunnel: w1125 -> [w1135]
          frame #0 {
            n617 = local write "测头机构轴速度(mm/s)"(30.0 ("测头机构轴速度(mm/s)")) -> ()
          }
          frame #1 {
            n618 = local read "测头机构轴后退位"() -> (w1127:dbl)
            n619 = local read "测头机构电机"() -> (w1129:u32)
            n620 = while {
              tunnel: w1129 -> [w1133]
              tunnel: w1127 -> [w1132]
              tunnel: [w1131] -> w1128
              stop <- w1134 stop-if-true
              n621 = Wait Until Next ms Multiple(millisecond multiple=u32 50 ("毫秒倍数")) -> ()  [unwired: 1 out]
              n622 = call "PCI1220U进给轴位置模式.vi"("Distance"=w1132, "AxisHandle IN"=w1133) -> ("AbsSuccess"=w1134:bool, "AxisHandle OUT"=w1131:u32)  [unwired: 8 in]
            }
          }
          frame #2 {
            n623 = while {
              tunnel: w1135 -> [w1139]
              stop <- w1137 stop-if-true
              n624 = call <userlib>:"Acm_AxGetCmdVelocity.vi"("AxisHandle"=w1139) -> ("Velocity"=w1138:dbl)  [unwired: 1 in, 3 out]
              n625 = Wait Until Next ms Multiple(millisecond multiple=u32 50 ("毫秒倍数")) -> ()  [unwired: 1 out]
              n626 = Equal To 0?(x=w1138) -> (x = 0?=w1137:bool)
            }
          }
          frame #3 {
            n627 = while {
              stop <- w1140 stop-if-true
              n628 = local read "测头机构轴位置(mm)"() -> (w1142:dbl)
              n629 = Wait Until Next ms Multiple(millisecond multiple=u32 50 ("毫秒倍数")) -> ()  [unwired: 1 out]
              n630 = Less Or Equal?(x=w1142, y=35.0) -> (x <= y?=w1140:bool)
            }
          }
          frame #4 {
            n631 = local write "测头气缸左移"(TRUE ("测头气缸左移")) -> ()
            n632 = local write "测头气缸右移"(FALSE ("测头气缸右移")) -> ()
          }
          frame #5 {
            n633 = Wait Until Next ms Multiple(millisecond multiple=u32 500 ("毫秒倍数")) -> ()  [unwired: 1 out]
          }
          frame #6 {
            n634 = local write "工步号"(u32 50 ("工步号")) -> ()
          }
        }
      }
      frame 50 {
        n635 = flat-sequence {
          tunnel: [w1169] -> w1158
          tunnel: w1158 -> [w1176]
          tunnel: [w1175] -> w1156
          tunnel: w1156 -> [w1187]
          tunnel: [w1194] -> w1150
          tunnel: [w1198] -> w1151
          tunnel: w1150 -> [w1198]
          tunnel: [w1201] -> w1153
          tunnel: w1151 -> [w1200]
          tunnel: w1153 -> [w1208]
          tunnel: [w1207] -> w1152
          tunnel: w1152 -> [w1210]
          tunnel: [w1209] -> w1148
          tunnel: [w1215] -> w1149
          tunnel: w1148 -> [w1215]
          tunnel: [w1218] -> w1157
          tunnel: w1149 -> [w1217]
          tunnel: w1157 -> [w1224]
          tunnel: [w1225] -> w1155
          tunnel: w1155 -> [w1234]
          tunnel: [w1233] -> w1154
          tunnel: w1154 -> [w1244]
          frame #0 {
            n636 = local write "旋转伺服速度(°/s)"(15.0 ("调整螺塞轴速度(°/s)")) -> ()
            n637 = local write "测头机构轴速度(mm/s)"(15.0 ("调整机构轴速度(mm/s)")) -> ()
            n638 = local write "电动缸速度(mm/s)"(15.0 ("电动缸速度(mm/s)")) -> ()
            n639 = local write "夹头松开"(TRUE ("夹头松开")) -> ()
            n640 = local write "夹头夹紧"(FALSE ("夹头夹紧")) -> ()
          }
          frame #1 {
            n641 = while {
              stop <- w1164 stop-if-true
              n642 = local read "夹头夹紧位"() -> (w1167:bool)
              n643 = local read "夹头松开"() -> (w1165:bool)
              n644 = Wait Until Next ms Multiple(millisecond multiple=u32 50 ("毫秒倍数")) -> ()  [unwired: 1 out]
              n645 = Not(x=w1167) -> (.not. x?=w1166:bool)
              n646 = And(x=w1166, y=w1165) -> (x .and. y?=w1164:bool)
            }
          }
          frame #2 {
            n647 = while {
              tunnel: [w1172] -> w1169
              stop <- w1171 stop-if-true
              n648 = local read "电动缸电机"() -> (w1173:u32)
              n649 = Wait Until Next ms Multiple(millisecond multiple=u32 50 ("毫秒倍数")) -> ()  [unwired: 1 out]
              n650 = local read "齿条右极限"() -> (w1170:dbl)
              n651 = call "PCI1240电动缸位置模式 .vi"("Distance"=w1170, "AxisHandle IN"=w1173) -> ("AbsSuccess"=w1171:bool, "AxisHandle OUT"=w1172:u32)  [unwired: 8 in]
            }
          }
          frame #3 {
            n652 = while {
              tunnel: w1176 -> [w1185]
              tunnel: [w1177] -> w1175
              stop <- w1178 stop-if-true
              n653 = local read "齿条推拉力(N)"() -> (w1183:dbl)
              n654 = Wait Until Next ms Multiple(millisecond multiple=u32 50 ("毫秒倍数")) -> ()  [unwired: 1 out]
              n655 = call <userlib>:"Acm_AxGetCmdVelocity.vi"("AxisHandle"=w1185) -> ("Velocity"=w1186:dbl, "AxisHandle"=w1177:u32)  [unwired: 1 in, 2 out]
              n656 = Equal To 0?(x=w1186) -> (x = 0?=w1180:bool)
              n657 = Absolute Value(x=w1183) -> (abs(x)=w1182:dbl)
              n658 = Greater Or Equal?(x=w1182, y=1000.0) -> (x >= y?=w1179:bool)
              n659 = Or(x=w1180, y=w1179) -> (x .or. y?=w1178:bool)
            }
          }
          frame #4 {
            n660 = while {
              tunnel: w1187 -> [w1191]
              tunnel: [w1190] -> _
              stop <- w1189 stop-if-true
              n661 = call "PCI1220U停止.vi"("AxisHandle IN"=w1191) -> ("完成"=w1189:bool, "AxisHandle OUT"=w1190:u32)  [unwired: 9 in]
              n662 = Wait (ms)(milliseconds to wait=u32 50 ("毫秒倍数")) -> ()  [unwired: 1 out]
            }
          }
          frame #5 {
            n663 = local write "旋转齿条轴使能"(TRUE ("旋转齿条轴使能")) -> ()
          }
          frame #6 {
            n664 = Wait Until Next ms Multiple(millisecond multiple=u32 500 ("毫秒倍数")) -> ()  [unwired: 1 out]
          }
          frame #7 {
            n665 = local read "旋转齿条电机"() -> (w1195:u32)
            n666 = call <userlib>:"Acm_AxHome.vi"("DirMode"=u32 0, "HomeMode"=u32 11, "AxisHandle"=w1195) -> ("AxisHandle"=w1194:u32)  [unwired: 1 in, 2 out]
          }
          frame #8 {
            n667 = Wait Until Next ms Multiple(millisecond multiple=u32 100 ("毫秒倍数")) -> ()  [unwired: 1 out]
          }
          frame #9 {
            n668 = while {
              tunnel: w1200 -> [w1204]
              tunnel: [w1203] -> w1201
              stop <- w1202 stop-if-true
              n669 = call <userlib>:"Acm_AxGetCmdVelocity.vi"("AxisHandle"=w1204) -> ("Velocity"=w1206:dbl, "AxisHandle"=w1203:u32)  [unwired: 1 in, 2 out]
              n670 = Equal To 0?(x=w1206) -> (x = 0?=w1202:bool)
              n671 = Wait Until Next ms Multiple(millisecond multiple=u32 50 ("毫秒倍数")) -> ()  [unwired: 1 out]
            }
          }
          frame #10 {
            n672 = call "PCI1220U角度置零.vi"("AxisHandle IN"=w1208) -> ("AxisHandle OUT"=w1207:u32)  [unwired: 10 in]
          }
          frame #11 {
            n673 = while {
              tunnel: [w1211] -> w1209
              tunnel: w1210 -> [w1211]
              stop <- w1214 stop-if-true
              n674 = Wait Until Next ms Multiple(millisecond multiple=u32 50 ("毫秒倍数")) -> ()  [unwired: 1 out]
              n675 = call "PCI1220U扭矩轴位置模式.vi"("Distance"=15.0, "AxisHandle IN"=w1211) -> ("AbsSuccess"=w1214:bool)  [unwired: 8 in, 1 out]
            }
          }
          frame #12 {
            n676 = Wait Until Next ms Multiple(millisecond multiple=u32 100 ("毫秒倍数")) -> ()  [unwired: 1 out]
          }
          frame #13 {
            n677 = while {
              tunnel: w1217 -> [w1221]
              tunnel: [w1220] -> w1218
              stop <- w1219 stop-if-true
              n678 = call <userlib>:"Acm_AxGetCmdVelocity.vi"("AxisHandle"=w1221) -> ("Velocity"=w1223:dbl, "AxisHandle"=w1220:u32)  [unwired: 1 in, 2 out]
              n679 = Equal To 0?(x=w1223) -> (x = 0?=w1219:bool)
              n680 = Wait Until Next ms Multiple(millisecond multiple=u32 50 ("毫秒倍数")) -> ()  [unwired: 1 out]
            }
          }
          frame #14 {
            n681 = call "PCI1220U角度置零.vi"("AxisHandle IN"=w1224) -> ()  [unwired: 10 in, 1 out]
          }
          frame #15 {
            n682 = while {
              tunnel: [w1230] -> w1225
              stop <- w1229 stop-if-true
              n683 = local read "电动缸电机"() -> (w1231:u32)
              n684 = Wait Until Next ms Multiple(millisecond multiple=u32 50 ("毫秒倍数")) -> ()  [unwired: 1 out]
              n685 = local read "齿条右极限"() -> (w1228:dbl)
              n686 = Add(x=w1228, y=-10.0) -> (x+y=w1226:dbl)
              n687 = call "PCI1240电动缸位置模式 .vi"("Distance"=w1226, "AxisHandle IN"=w1231) -> ("AbsSuccess"=w1229:bool, "AxisHandle OUT"=w1230:u32)  [unwired: 8 in]
            }
          }
          frame #16 {
            n688 = while {
              tunnel: w1234 -> [w1242]
              tunnel: [w1240] -> w1233
              stop <- w1235 stop-if-true
              n689 = local read "齿条推拉力(N)"() -> (w1239:dbl)
              n690 = Wait Until Next ms Multiple(millisecond multiple=u32 50 ("毫秒倍数")) -> ()  [unwired: 1 out]
              n691 = call <userlib>:"Acm_AxGetCmdVelocity.vi"("AxisHandle"=w1242) -> ("Velocity"=w1243:dbl, "AxisHandle"=w1240:u32)  [unwired: 1 in, 2 out]
              n692 = Equal To 0?(x=w1243) -> (x = 0?=w1236:bool)
              n693 = Greater Or Equal?(x=w1239, y=300.0) -> (x >= y?=w1237:bool)
              n694 = Or(x=w1236, y=w1237) -> (x .or. y?=w1235:bool)
            }
          }
          frame #17 {
            n695 = while {
              tunnel: w1244 -> [w1248]
              tunnel: [w1247] -> _
              stop <- w1246 stop-if-true
              n696 = call "PCI1220U停止.vi"("AxisHandle IN"=w1248) -> ("完成"=w1246:bool, "AxisHandle OUT"=w1247:u32)  [unwired: 9 in]
              n697 = Wait (ms)(milliseconds to wait=u32 50 ("毫秒倍数")) -> ()  [unwired: 1 out]
            }
          }
          frame #18 {
            n698 = local write "工步号"(u32 100 ("工步号")) -> ()
          }
        }
      }
      frame 100 {
        n699 = flat-sequence {
          tunnel: [w1283] -> w1273
          tunnel: [w1281] -> w1272
          tunnel: [w1275] -> w1259
          tunnel: [w1274] -> w1257
          tunnel: w1273 -> [w1290]
          tunnel: w1272 -> [w1287]
          tunnel: ["F:\\报表存储\\" ("字符串")] -> w1271
          tunnel: [w1290] -> w1260
          tunnel: w1259 -> [w1289]
          tunnel: [w1289] -> w1258
          tunnel: w1257 -> [w1288]
          tunnel: [w1288] -> w1256
          tunnel: [w1287] -> w1255
          tunnel: w1271 -> [w1301]
          tunnel: [w1309] -> w1270
          tunnel: [w1306] -> w1269
          tunnel: [w1305] -> w1268
          tunnel: [w1304] -> w1267
          tunnel: w1260 -> [w1300]
          tunnel: w1258 -> [w1299]
          tunnel: w1256 -> [w1298]
          tunnel: w1255 -> [w1292]
          tunnel: [w1294] -> w1254
          tunnel: w1270 -> [w1316]
          tunnel: [w1317] -> w1266
          tunnel: w1269 -> [w1317]
          tunnel: w1268 -> [w1315]
          tunnel: w1267 -> [w1314]
          tunnel: [w1313] -> w1265
          tunnel: [w1312] -> w1264
          tunnel: w1254 -> [w1311]
          tunnel: [w1311] -> w1253
          tunnel: [w1324] -> w1263
          tunnel: w1266 -> [w1324]
          tunnel: w1265 -> [w1323]
          tunnel: [w1323] -> w1262
          tunnel: [w1322] -> w1261
          tunnel: w1264 -> [w1322]
          tunnel: w1253 -> [w1320]
          tunnel: [w1320] -> w1252
          tunnel: w1263 -> [w1327]
          tunnel: w1262 -> [w1335]
          tunnel: w1261 -> [w1334]
          tunnel: w1252 -> [w1326]
          tunnel: [w1326] -> w1251
          tunnel: w1251 -> [w1343]
          tunnel: [w1343] -> w1250
          tunnel: w1250 -> [w1345]
          frame #0 {
            n700 = local read "产品ID"() -> (w1282:string)
            n701 = Format Date/Time String(time format string (%c)="%Y%m%d" ("时间格式字符串(%c)")) -> (date/time string=w1276:string)  [unwired: 2 in]
            n702 = String Subset(string=w1276, offset (0)=4 ("偏移量(0)"), length (rest)=2 ("长度（剩余）")) -> (substring=w1275:string)
            n703 = String Subset(string=w1276, offset (0)=6 ("偏移量(0)"), length (rest)=2 ("长度（剩余）")) -> (substring=w1274:string)
            n704 = call <vilib>:"Trim Whitespace.vi"("string"=w1282) -> ("trimmed string"=w1281:string)  [unwired: 1 in]
            n705 = String Subset(string=w1276, offset (0)=0 ("偏移量(0)"), length (rest)=4 ("长度（剩余）")) -> (substring=w1283:string)
          }
          frame #1 {
          }
          frame #2 {
            w1293 = "\\" ("字符串")
            n706 = Concatenate Strings(w1301, w1300, w1293, w1299, w1293, w1298, w1293, w1292, w1293) -> (w1296:string)
            n707 = Concatenate Strings(w1301, w1300, w1293, w1299, w1293, w1298, w1293, w1292, w1293) -> (w1310:string)
            n708 = String To Path(string=w1310) -> (path=w1309:path)
            n709 = Concatenate Strings(w1296, w1292, "间隙曲线.JPG" ("字符串")) -> (w1307:string)
            n710 = Concatenate Strings(w1296, "轴向力曲线数组.txt" ("字符串")) -> (w1304:string)
            n711 = Concatenate Strings(w1296, "扭动曲线数组.txt" ("字符串")) -> (w1305:string)
            n712 = Concatenate Strings(w1296, w1292, "轴向力曲线.JPG" ("字符串")) -> (w1297:string)
            n713 = String To Path(string=w1307) -> (path=w1306:path)
            n714 = String To Path(string=w1297) -> (path=w1294:path)
          }
          frame #3 {
            n715 = call <vilib>:"Check if File or Folder Exists.vi"("path"=w1316) -> ("file or folder exists?"=w1318:bool)  [unwired: 8 in, 2 out]
            n716 = String To Path(string=w1314) -> (path=w1312:path)
            n717 = String To Path(string=w1315) -> (path=w1313:path)
            n718 = case shown="假" w1318 {
              tunnel: w1316 -> [w1319 _]
              frame False {
                n719 = Create Folder(path (use dialog)=w1319) -> ()  [unwired: 2 in, 3 out]
              }
              frame True {
              }
            }
          }
          frame #4 {
            n720 = local write "选项卡控件"(T1."间隙测量" ("选项卡控件")) -> ()
            n721 = Wait Until Next ms Multiple(millisecond multiple=u32 1000 ("毫秒倍数")) -> ()  [unwired: 1 out]
          }
          frame #5 {
            n722 = disable-structure shown="禁用" {
              disable-tunnel: w1327 -> [w1336 _]
              frame Disabled {
                w1340 = T2 2 items=["快速打印", "标准报表", "HTML", "双字节", "Excel"] ("report type (Quick Print)")
                w1339 = T3 1 items=["完整前面板", "前面板可见部分", "图标、说明、前面板和程序框图", "说明信息: 使用前面板", "说明信息: 作为子VI使用", "说明信息: 完整", "说明信息: 自定义"] ("contents (complete front panel)")
                n723 = Current VI's Path() -> (path=w1338:path)
                n724 = call-poly <vilib>:"Easy Print VI Panel or Documentation.vi"("report type (Quick Print)"=w1340, "contents (complete front panel)"=w1339, "VI path"=w1338) -> ("error out"=w1342:errorcluster, "report out"=w1341:refnum<class "NI_report.lvclass">)  [unwired: 1 in, 6 out]
                n725 = call-dynamic "Save Report to File.vi"("report in"=w1341, "report file path"=w1336, "error in (no error)"=w1342) -> ("error out"=→"error out 3":errorcluster)  [unwired: 2 in, 10 out]
              }
              frame Enabled {
              }
            }
            n726 = local read "间隙Y数组"() -> (w1332:dbl[])
            n727 = local read "间隙X数组"() -> (w1333:dbl[])
            n728 = local read "轴向力Y"() -> (w1330:dbl[])
            n729 = local read "轴向力X"() -> (w1331:dbl[])
            n730 = call "导出曲线数组.vi"("file path (dialog if empty)"=w1335, "数组 2"=w1332, "数组"=w1333) -> ()  [unwired: 9 in]
            n731 = call "导出曲线数组.vi"("file path (dialog if empty)"=w1334, "数组 2"=w1330, "数组"=w1331) -> ()  [unwired: 9 in]
            n732 = control-ref of="本VI"() -> (w1329:refnum<vi>)
            n733 = invoke class="VI" method="FP.Get Image"(reference=w1329) -> ("image data"=w1328:T4)  [unwired: 5 in, 5 out]
            n734 = call <vilib>:"Write JPEG File.vi"("image data"=w1328, "path to JPEG file"=w1327) -> ()  [unwired: 8 in, 2 out]
          }
          frame #6 {
            n735 = local write "选项卡控件"(T1."轴向力测量" ("选项卡控件")) -> ()
          }
          frame #7 {
            n736 = control-ref of="本VI"() -> (w1346:refnum<vi>)
            n737 = invoke class="VI" method="FP.Get Image"(reference=w1346) -> ("image data"=w1347:T4)  [unwired: 5 in, 5 out]
            n738 = call <vilib>:"Write JPEG File.vi"("image data"=w1347, "path to JPEG file"=w1345) -> ()  [unwired: 8 in, 2 out]
          }
          frame #8 {
            n739 = local read "联线按钮"() -> (w1348:bool)
            n740 = case shown="真" w1348 {
              frame False {
              }
              frame True {
                n741 = flat-sequence {
                  tunnel: [w1375] -> w1349
                  tunnel: w1349 -> [w1390]
                  frame #0 {
                    w1368 = i16 3 ("精度(6)")
                    n742 = local read "全行程间隙及轴向力合格"() -> (w1370:bool)
                    n743 = local read "左180°外全行程间隙"() -> (w1367:dbl)
                    n744 = local read "右180°内全行程间隙"() -> (w1369:dbl)
                    n745 = local read "右180°外全行程间隙"() -> (w1366:dbl)
                    n746 = local read "左最大轴向力(N)"() -> (w1365:dbl)
                    n747 = local read "右最大轴向力(N)"() -> (w1364:dbl)
                    n748 = local read "左轴向力波动(N)"() -> (w1363:dbl)
                    n749 = local read "单点间隙合格"() -> (w1371:bool)
                    n750 = local read "右轴向力波动(N)"() -> (w1362:dbl)
                    n751 = local read "左180°内全行程间隙"() -> (w1378:dbl)
                    n752 = local read "总行程(mm)"() -> (w1361:dbl)
                    n753 = local read "总圈数"() -> (w1360:dbl)
                    n754 = local read "员工ID"() -> (w1350:string)
                    n755 = local read "中间位置间隙"() -> (w1380:dbl)
                    n756 = local read "FGCS"() -> (w1382:string)
                    n757 = And(x=w1371, y=w1370) -> (x .and. y?=w1372:bool)
                    n758 = local read "KSJJ"() -> (w1384:string)
                    n759 = local read "产品ID"() -> (w1387:string)
                    n760 = Boolean To (0,1)(Boolean=w1372) -> (0, 1=w1386:i16)
                    n761 = Number To Fractional String(number=w1361, precision (6)=w1368) -> (F-format string=w1352:string)  [unwired: 2 in]
                    n762 = Number To Fractional String(number=w1363, precision (6)=w1368) -> (F-format string=w1354:string)  [unwired: 2 in]
                    n763 = Number To Fractional String(number=w1362, precision (6)=w1368) -> (F-format string=w1353:string)  [unwired: 2 in]
                    n764 = Number To Fractional String(number=w1369, precision (6)=w1368) -> (F-format string=w1359:string)  [unwired: 2 in]
                    n765 = Number To Fractional String(number=w1367, precision (6)=w1368) -> (F-format string=w1358:string)  [unwired: 2 in]
                    n766 = Number To Fractional String(number=w1360, precision (6)=w1368) -> (F-format string=w1351:string)  [unwired: 2 in]
                    n767 = Number To Fractional String(number=w1378, precision (6)=w1368) -> (F-format string=w1376:string)  [unwired: 2 in]
                    n768 = Number To Fractional String(number=w1364, precision (6)=w1368) -> (F-format string=w1355:string)  [unwired: 2 in]
                    n769 = Number To Fractional String(number=w1366, precision (6)=w1368) -> (F-format string=w1357:string)  [unwired: 2 in]
                    n770 = Number To Fractional String(number=w1365, precision (6)=w1368) -> (F-format string=w1356:string)  [unwired: 2 in]
                    n771 = Number To Fractional String(number=w1380, precision (6)=i16 3 ("精度(6)")) -> (F-format string=w1377:string)  [unwired: 2 in]
                    n772 = Format Date/Time String(time format string (%c)="%Y%m%d%H%M" ("时间格式字符串(%c)")) -> (date/time string=w1383:string)  [unwired: 2 in]
                    n773 = Number To Decimal String(number=w1386, width (-)=i16 1 ("宽度(-)")) -> (decimal integer string=w1373:string)
                    n774 = Build Array(w1387, w1350, "1", w1373, w1384, w1383, w1382, "Q14070-Z060A", w1377, w1376, w1359, w1358, w1357, w1356, w1355, w1354, w1353, w1352, w1351) -> (w1375:string[])
                  }
                  frame #1 {
                    n775 = Wait (ms)(milliseconds to wait=u32 500 ("等待时间（毫秒）")) -> ()  [unwired: 1 out]
                    n776 = call "数据库更新.vi"("设备号"="06", "数据"=w1390) -> ()  [unwired: 13 in, 1 out]
                  }
                  frame #2 {
                  }
                }
              }
            }
          }
          frame #9 {
            n777 = local write "产品ID"("") -> ()
            n778 = local write "工步号"(u32 0 ("工步号")) -> ()
          }
        }
      }
    }
    n779 = Wait (ms)(milliseconds to wait=u32 50 ("毫秒倍数")) -> ()  [unwired: 1 out]
    n780 = local read "停止"() -> (w7:bool)
  }
  n781 = while {
    stop <- w1394 stop-if-true
    n782 = event shown="[3] \"参数查询\": 值改变" {
      selector: _ -> [_ _ _ _ _ _ _]
      dyn-events: _ -> [_ _ _ _ _ _ _]
      timeout: 500 -> [_ _ _ _ _ _ _]
      event Timeout {
        n783 = event-data() -> ()  [unwired: 3 out]
      }
      event "停止": Value Change {
        n784 = event-data() -> ()  [unwired: 6 out]
        n785 = flat-sequence {
          frame #0 {
            n786 = Wait (ms)(milliseconds to wait=u32 1000 ("毫秒倍数")) -> ()  [unwired: 1 out]
          }
          frame #1 {
            n787 = Quit LabVIEW(quit? (T)=TRUE ("停止？(T)")) -> ()
          }
        }
      }
      event "参数修改": Value Change {
        n788 = event-data() -> ()  [unwired: 6 out]
        n789 = while {
          i -> [w1446]
          stop <- w1445 stop-if-true
          n790 = local read "型号数量"() -> (w1447:i32)
          n791 = local read "参数浏览表"() -> (w1448:string[][])
          n792 = Greater Or Equal?(x=w1446, y=w1447) -> (x >= y?=w1445:bool)
          n793 = Wait Until Next ms Multiple(millisecond multiple=u32 50 ("毫秒倍数")) -> ()  [unwired: 1 out]
          n794 = Index Array(array=w1448, index (col)=w1446) -> (element=w1433:string[])  [unwired: 1 in]
          n795 = Index Array(array=w1433, index #1=0 ("索引"), index #2=2 ("索引"), index #3=3 ("索引"), index #4=4 ("索引"), index #5=5 ("索引"), index #6=6 ("索引"), index #7=7 ("索引"), index #8=8 ("索引"), index #9=9 ("索引"), index #10=10 ("索引"), index #11=11 ("索引"), index #12=12 ("索引"), index #13=13 ("索引"), index #14=14 ("索引"), index #15=15 ("索引"), index #16=16 ("索引"), index #17=17 ("索引"), index #18=18 ("索引"), index #19=19 ("索引"), index #20=20 ("索引")) -> (element #1=w1400:string, element #2=w1429:string, element #3=w1428:string, element #4=w1427:string, element #5=w1426:string, element #6=w1425:string, element #7=w1424:string, element #8=w1423:string, element #9=w1422:string, element #10=w1421:string, element #11=w1420:string, element #12=w1415:string, element #13=w1414:string, element #14=w1413:string, element #15=w1412:string, element #16=w1411:string, element #17=w1406:string, element #18=w1405:string, element #19=w1404:string, element #20=w1399:string)
          n796 = call "创建文本"("测头机构轴移动速度"=w1429, "测头机构轴检测位"=w1428, "测头机构轴待检位"=w1427, "测头机构轴后退位"=w1426, "齿条移动速度"=w1425, "齿条左极限"=w1424, "齿条右极限"=w1423, "旋转齿条轴找帽转速"=w1422, "旋转齿条轴测量转速"=w1421, "测量点扭矩"=w1420, "总行程最大值"=w1414, "总行程最小值"=w1415, "最大轴向力"=w1413, "轴向力波动"=w1412, "平均轴向力最小值"=w1411, "平均轴向力最大值"=w1406, "总圈数最小值"=w1405, "总圈数最大值"=w1404, "中间位置"=w1399, "产品型号"=w1400) -> ("Result"=w1419:string)  [unwired: 6 in, 1 out]
          n797 = local read "ADODB._Connection Out 2"() -> (w1418:refnum<k7>)
          n798 = call "SQL Execute.vi"("Command Text"=w1419, "ADODB._Connection In"=w1418) -> ("error out"=w1431:errorcluster, "ADODB._Connection Out"=w1432:refnum<k7>)  [unwired: 6 in, 2 out]
          n799 = call "ADO Connection Close.vi"("error in (no error)"=w1431, "ADODB._Connection In"=w1432) -> ("error out"=→"error out":errorcluster)  [unwired: 8 in, 1 out]
        }
      }
      event "参数查询": Value Change {
        n800 = event-data() -> ()  [unwired: 6 out]
        n801 = flat-sequence {
          tunnel: [w1461] -> w1454
          tunnel: [w1460] -> w1453
          tunnel: [w1459] -> w1450
          tunnel: w1454 -> [w1465]
          tunnel: w1453 -> [w1467]
          tunnel: [w1467] -> w1452
          tunnel: [w1466] -> w1451
          tunnel: w1450 -> [w1466]
          tunnel: w1452 -> [_]
          tunnel: w1451 -> [_]
          frame #0 {
            n802 = call-poly <vilib>:"Read From Spreadsheet File.vi"("file path (dialog if empty)"=path "D:/Q14070-Z060人机界面/参数/参数项.txt") -> ("first row"=w1455:string[])  [unwired: 6 in, 4 out]
            n803 = property on="参数浏览表" class="Tbl (严格)"("Row Headers[]"=w1455) -> ()  [unwired: 2 in, 2 out]
          }
          frame #1 {
            n804 = local read "ADODB._Connection Out 2"() -> (w1458:refnum<k7>)
            n805 = call "SQL Execute.vi"("Command Text"="SELECT * FROM 测试参数表;", "ADODB._Connection In"=w1458) -> ("error out"=w1459:errorcluster, "Data"=w1463:string[][], "ADODB._Connection Out"=w1460:refnum<k7>)  [unwired: 6 in, 1 out]
            n806 = Transpose 2D Array(2D array=w1463) -> (transposed array=w1461:string[][])
            n807 = Index Array(array=w1461, index (row)=0 ("索引 (行)")) -> (element=w1462:string[])  [unwired: 1 in]
            n808 = property on="参数浏览表" class="Tbl (严格)"("Column Headers[]"=w1462) -> ()  [unwired: 2 in, 2 out]
          }
          frame #2 {
            n809 = local write "参数浏览表"(w1465) -> ()
          }
          frame #3 {
          }
        }
      }
      event "传感器参数保存": Value Change {
        n810 = event-data() -> ()  [unwired: 6 out]
        n811 = flat-sequence {
          tunnel: [w1493] -> w1490
          tunnel: [w1492] -> w1489
          tunnel: [w1491] -> w1488
          tunnel: [w1499] -> w1487
          tunnel: w1490 -> [w1499]
          tunnel: [w1498] -> w1486
          tunnel: w1489 -> [w1498]
          tunnel: [w1497] -> w1485
          tunnel: w1488 -> [w1497]
          tunnel: [w1496] -> w1484
          tunnel: [w1495] -> w1483
          tunnel: [w1494] -> w1482
          tunnel: [w1500] -> w1481
          tunnel: [w1506] -> w1480
          tunnel: w1487 -> [w1506]
          tunnel: [w1505] -> w1479
          tunnel: w1486 -> [w1505]
          tunnel: w1485 -> [w1504]
          tunnel: [w1504] -> w1478
          tunnel: [w1503] -> w1477
          tunnel: w1484 -> [w1503]
          tunnel: [w1502] -> w1476
          tunnel: w1483 -> [w1502]
          tunnel: [w1501] -> w1475
          tunnel: w1482 -> [w1501]
          tunnel: w1481 -> [w1525]
          tunnel: [w1525] -> w1474
          tunnel: w1480 -> [w1524]
          tunnel: w1479 -> [w1517]
          tunnel: w1478 -> [w1516]
          tunnel: w1477 -> [w1510]
          tunnel: w1476 -> [w1509]
          tunnel: w1475 -> [w1515]
          tunnel: [w1514] -> w1473
          tunnel: [w1513] -> w1472
          tunnel: [w1512] -> w1471
          tunnel: [w1508] -> w1470
          tunnel: [w1507] -> w1469
          tunnel: [w1511] -> w1468
          tunnel: w1474 -> [w1533]
          tunnel: w1473 -> [w1532]
          tunnel: w1472 -> [w1531]
          tunnel: w1471 -> [w1530]
          tunnel: w1470 -> [w1529]
          tunnel: w1469 -> [w1528]
          tunnel: w1468 -> [w1527]
          frame #0 {
            n812 = local read "齿条推拉力零点偏移"() -> (w1492:dbl)
            n813 = local read "间隙位移零点偏移"() -> (w1493:dbl)
            n814 = local read "齿条扭矩零点偏移"() -> (w1491:dbl)
          }
          frame #1 {
            n815 = local read "齿条推拉力比例偏移"() -> (w1495:dbl)
            n816 = local read "间隙位移比例偏移"() -> (w1496:dbl)
            n817 = local read "齿条扭矩比例偏移"() -> (w1494:dbl)
          }
          frame #2 {
            n818 = local read "ADODB._Connection Out 2"() -> (w1500:refnum<k7>)
          }
          frame #3 {
            n819 = Number To Fractional String(number=w1524, precision (6)=i16 2 ("精度(6)")) -> (F-format string=w1514:string)  [unwired: 2 in]
            n820 = Number To Fractional String(number=w1516, precision (6)=i16 2 ("精度(6)")) -> (F-format string=w1512:string)  [unwired: 2 in]
            n821 = Number To Fractional String(number=w1515, precision (6)=i16 2 ("精度(6)")) -> (F-format string=w1511:string)  [unwired: 2 in]
            n822 = Number To Fractional String(number=w1517, precision (6)=i16 2 ("精度(6)")) -> (F-format string=w1513:string)  [unwired: 2 in]
            n823 = Number To Fractional String(number=w1510, precision (6)=i16 2 ("精度(6)")) -> (F-format string=w1508:string)  [unwired: 2 in]
            n824 = Number To Fractional String(number=w1509, precision (6)=i16 2 ("精度(6)")) -> (F-format string=w1507:string)  [unwired: 2 in]
          }
          frame #4 {
            n825 = call "创建文本3"("4"=w1529, "6"=w1527, "1"=w1532, "2"=w1531, "3"=w1530, "5"=w1528) -> ("Result"=w1534:string)  [unwired: 8 in, 1 out]
            n826 = call "SQL Execute.vi"("Command Text"=w1534, "ADODB._Connection In"=w1533) -> ("error out"=→"error out 4":errorcluster)  [unwired: 6 in, 3 out]
          }
        }
      }
      event "产品ID": Value Change {
        n827 = event-data() -> ()  [unwired: 7 out]
        n828 = Format Date/Time String(time format string (%c)="%Y%m%d%H%M" ("时间格式字符串(%c)")) -> (date/time string=w1535:string)  [unwired: 2 in]
        n829 = local write "KSJJ"(w1535) -> ()
      }
      event "电动缸回零": Mouse Down {
        n830 = event-data() -> ()  [unwired: 6 out]
        n831 = stacked-sequence {
          frame #0 {
            n832 = flat-sequence {
              tunnel: [w1555] -> w1544
              tunnel: [w1548] -> w1541
              tunnel: w1544 -> [w1558]
              tunnel: [w1558] -> w1543
              tunnel: [w1556] -> w1542
              tunnel: w1541 -> [w1556]
              tunnel: w1543 -> [w1560]
              tunnel: [w1560] -> w1545
              tunnel: w1542 -> [w1559]
              tunnel: [w1559] -> w1540
              tunnel: w1545 -> [w1571]
              tunnel: w1540 -> [w1570]
              tunnel: [w1569] -> w1539
              tunnel: w1539 -> [w1573]
              tunnel: [w1572] -> w1538
              tunnel: w1538 -> [w1581]
              frame #0 {
                n833 = local write "电动缸速度(mm/s)"(15.0 ("电动缸速度(mm/s)")) -> ()
                n834 = local write "测头机构轴速度(mm/s)"(10.0 ("电动缸速度(mm/s)")) -> ()
              }
              frame #1 {
                n835 = local read "测头机构电机"() -> (w1552:u32)
                n836 = local read "电动缸电机"() -> (w1549:u32)
                n837 = call <userlib>:"Acm_AxHome.vi"("DirMode"=u32 0, "HomeMode"=u32 11, "AxisHandle"=w1552) -> ("AxisHandle"=w1555:u32)  [unwired: 1 in, 2 out]
                n838 = call <userlib>:"Acm_AxHome.vi"("DirMode"=u32 1, "HomeMode"=u32 11, "AxisHandle"=w1549) -> ("AxisHandle"=w1548:u32)  [unwired: 1 in, 2 out]
              }
              frame #2 {
                n839 = Wait Until Next ms Multiple(millisecond multiple=u32 100 ("毫秒倍数")) -> ()  [unwired: 1 out]
              }
              frame #3 {
                n840 = while {
                  tunnel: w1560 -> [w1568]
                  stop <- w1566 stop-if-true
                  n841 = call <userlib>:"Acm_AxGetCmdVelocity.vi"("AxisHandle"=w1568) -> ("Velocity"=w1567:dbl)  [unwired: 1 in, 3 out]
                  n842 = Wait Until Next ms Multiple(millisecond multiple=u32 50 ("毫秒倍数")) -> ()  [unwired: 1 out]
                  n843 = Equal To 0?(x=w1567) -> (x = 0?=w1566:bool)
                }
                n844 = while {
                  tunnel: w1559 -> [w1564]
                  stop <- w1562 stop-if-true
                  n845 = call <userlib>:"Acm_AxGetCmdVelocity.vi"("AxisHandle"=w1564) -> ("Velocity"=w1563:dbl)  [unwired: 1 in, 3 out]
                  n846 = Wait Until Next ms Multiple(millisecond multiple=u32 50 ("毫秒倍数")) -> ()  [unwired: 1 out]
                  n847 = Equal To 0?(x=w1563) -> (x = 0?=w1562:bool)
                }
              }
              frame #4 {
                n848 = call "PCI1220U角度置零.vi"("AxisHandle IN"=w1571) -> ()  [unwired: 10 in, 1 out]
                n849 = call "PCI1220U角度置零.vi"("AxisHandle IN"=w1570) -> ("AxisHandle OUT"=w1569:u32)  [unwired: 10 in]
              }
              frame #5 {
                n850 = while {
                  tunnel: [w1579] -> w1572
                  tunnel: w1573 -> [w1574]
                  stop <- w1578 stop-if-true
                  n851 = Wait Until Next ms Multiple(millisecond multiple=u32 50 ("毫秒倍数")) -> ()  [unwired: 1 out]
                  n852 = local read "齿条右极限"() -> (w1577:dbl)
                  n853 = Add(x=w1577, y=-10.0) -> (x+y=w1575:dbl)
                  n854 = call "PCI1240电动缸位置模式 .vi"("Distance"=w1575, "AxisHandle IN"=w1574) -> ("AbsSuccess"=w1578:bool, "AxisHandle OUT"=w1579:u32)  [unwired: 8 in]
                }
              }
              frame #6 {
                n855 = while {
                  tunnel: w1581 -> [w1585]
                  stop <- w1583 stop-if-true
                  n856 = call <userlib>:"Acm_AxGetCmdVelocity.vi"("AxisHandle"=w1585) -> ("Velocity"=w1584:dbl)  [unwired: 1 in, 3 out]
                  n857 = Wait Until Next ms Multiple(millisecond multiple=u32 50 ("毫秒倍数")) -> ()  [unwired: 1 out]
                  n858 = Equal To 0?(x=w1584) -> (x = 0?=w1583:bool)
                }
              }
            }
          }
          frame #1 {
            n859 = flat-sequence {
              tunnel: [w1597] -> w1592
              tunnel: w1592 -> [w1599]
              tunnel: [w1599] -> w1591
              tunnel: w1591 -> [w1600]
              tunnel: [w1600] -> w1590
              tunnel: w1590 -> [w1606]
              tunnel: [w1605] -> w1587
              tunnel: w1587 -> [w1608]
              tunnel: [w1608] -> w1586
              tunnel: w1586 -> [w1610]
              tunnel: [w1609] -> w1589
              tunnel: w1589 -> [w1616]
              tunnel: [w1616] -> w1588
              tunnel: w1588 -> [w1621]
              frame #0 {
                n860 = local write "旋转伺服速度(°/s)"(5.0 ("电动缸速度(mm/s)")) -> ()
              }
              frame #1 {
                n861 = local read "旋转齿条电机"() -> (w1594:u32)
                n862 = call <userlib>:"Acm_AxHome.vi"("DirMode"=u32 0, "HomeMode"=u32 11, "AxisHandle"=w1594) -> ("AxisHandle"=w1597:u32)  [unwired: 1 in, 2 out]
              }
              frame #2 {
                n863 = Wait Until Next ms Multiple(millisecond multiple=u32 100 ("毫秒倍数")) -> ()  [unwired: 1 out]
              }
              frame #3 {
                n864 = while {
                  tunnel: w1600 -> [w1604]
                  stop <- w1602 stop-if-true
                  n865 = call <userlib>:"Acm_AxGetCmdVelocity.vi"("AxisHandle"=w1604) -> ("Velocity"=w1603:dbl)  [unwired: 1 in, 3 out]
                  n866 = Wait Until Next ms Multiple(millisecond multiple=u32 50 ("毫秒倍数")) -> ()  [unwired: 1 out]
                  n867 = Equal To 0?(x=w1603) -> (x = 0?=w1602:bool)
                }
              }
              frame #4 {
                n868 = call "PCI1220U角度置零.vi"("AxisHandle IN"=w1606) -> ("AxisHandle OUT"=w1605:u32)  [unwired: 10 in]
              }
              frame #5 {
                n869 = Wait (ms)(milliseconds to wait=u32 100 ("等待时间（毫秒）")) -> ()  [unwired: 1 out]
              }
              frame #6 {
                n870 = while {
                  tunnel: [w1614] -> w1609
                  tunnel: w1610 -> [w1611]
                  stop <- w1613 stop-if-true
                  n871 = Wait Until Next ms Multiple(millisecond multiple=u32 50 ("毫秒倍数")) -> ()  [unwired: 1 out]
                  n872 = call "PCI1220U扭矩轴位置模式.vi"("Distance"=15.0, "AxisHandle IN"=w1611) -> ("AbsSuccess"=w1613:bool, "AxisHandle OUT"=w1614:u32)  [unwired: 8 in]
                }
              }
              frame #7 {
                n873 = while {
                  tunnel: w1616 -> [w1619]
                  stop <- w1617 stop-if-true
                  n874 = call <userlib>:"Acm_AxGetCmdVelocity.vi"("AxisHandle"=w1619) -> ("Velocity"=w1620:dbl)  [unwired: 1 in, 3 out]
                  n875 = Wait Until Next ms Multiple(millisecond multiple=u32 50 ("毫秒倍数")) -> ()  [unwired: 1 out]
                  n876 = Equal To 0?(x=w1620) -> (x = 0?=w1617:bool)
                }
              }
              frame #8 {
                n877 = call "PCI1220U角度置零.vi"("AxisHandle IN"=w1621) -> ()  [unwired: 10 in, 1 out]
              }
            }
          }
          frame #2 {
            n878 = flat-sequence {
              frame #0 {
                n879 = while {
                  stop <- w1625 stop-if-true
                  n880 = local read "电动缸回零"() -> (w1626:bool)
                  n881 = local write "回零完成"(TRUE ("回零完成")) -> ()
                  n882 = local write "电动缸回零"(FALSE ("电动缸回零")) -> ()
                  n883 = Wait Until Next ms Multiple(millisecond multiple=u32 50 ("毫秒倍数")) -> ()  [unwired: 1 out]
                  n884 = Not(x=w1626) -> (.not. x?=w1625:bool)
                }
              }
            }
          }
        }
        n885 = Wait Until Next ms Multiple(millisecond multiple=u32 50 ("毫秒倍数")) -> ()  [unwired: 1 out]
      }
    }
    n886 = Wait (ms)(milliseconds to wait=u32 50 ("毫秒倍数")) -> ()  [unwired: 1 out]
    n887 = local read "停止"() -> (w1394:bool)
  }
  n888 = call "PCI1240电动缸位置模式 .vi"() -> ()  [unwired: 10 in, 2 out]
  n889 = while {
    stop <- w1628 stop-if-true
    n890 = stacked-sequence {
      frame #0 {
        n891 = flat-sequence {
          frame #0 {
          }
          frame #1 {
            n892 = First Call?() -> (First Call?: T/F=w1629:bool)
            n893 = case shown="真" w1629 {
              frame False {
              }
              frame True {
                n894 = call "员工管理测试程序.vi"() -> ("员工姓名"=w1631:string, "员工ID"=w1630:string)  [unwired: 10 in]
                n895 = local write "员工ID"(w1630) -> ()
                n896 = local write "员工姓名"(w1631) -> ()
              }
            }
          }
          frame #2 {
          }
          frame #3 {
          }
          frame #4 {
          }
          frame #5 {
          }
          frame #6 {
          }
        }
      }
      frame #1 {
        n897 = flat-sequence {
          frame #0 {
            n898 = property on="型号选择" class="Ring (严格)"() -> ("RingText.Text"=w1632:string)  [unwired: 2 in, 2 out]
            n899 = case shown="\"J706\"" w1632 {
              frame "J706" {
                w1633 = FALSE ("可见")
                w1634 = TRUE ("可见")
                n900 = property on="左180°内全行程间隙" class="DigNum (严格)"("Visible"=w1634) -> ()  [unwired: 2 in, 2 out]
                n901 = property on="左180°外全行程间隙" class="DigNum (严格)"("Visible"=w1634) -> ()  [unwired: 2 in, 2 out]
                n902 = property on="右180°外全行程间隙" class="DigNum (严格)"("Visible"=w1634) -> ()  [unwired: 2 in, 2 out]
                n903 = property on="右180°内全行程间隙" class="DigNum (严格)"("Visible"=w1634) -> ()  [unwired: 2 in, 2 out]
                n904 = property on="左全行程间隙" class="DigNum (严格)"("Visible"=w1633) -> ()  [unwired: 2 in, 2 out]
                n905 = property on="右全行程间隙" class="DigNum (严格)"("Visible"=w1633) -> ()  [unwired: 2 in, 2 out]
              }
              frame "J728" {
                w1635 = FALSE ("可见")
                w1636 = TRUE ("可见")
                n906 = property on="左180°内全行程间隙" class="DigNum (严格)"("Visible"=w1636) -> ()  [unwired: 2 in, 2 out]
                n907 = property on="左180°外全行程间隙" class="DigNum (严格)"("Visible"=w1636) -> ()  [unwired: 2 in, 2 out]
                n908 = property on="右180°外全行程间隙" class="DigNum (严格)"("Visible"=w1636) -> ()  [unwired: 2 in, 2 out]
                n909 = property on="右180°内全行程间隙" class="DigNum (严格)"("Visible"=w1636) -> ()  [unwired: 2 in, 2 out]
                n910 = property on="左全行程间隙" class="DigNum (严格)"("Visible"=w1635) -> ()  [unwired: 2 in, 2 out]
                n911 = property on="右全行程间隙" class="DigNum (严格)"("Visible"=w1635) -> ()  [unwired: 2 in, 2 out]
              }
              frame "J709", Default {
                w1637 = TRUE ("可见")
                w1638 = FALSE ("可见")
                n912 = property on="左180°内全行程间隙" class="DigNum (严格)"("Visible"=w1638) -> ()  [unwired: 2 in, 2 out]
                n913 = property on="左180°外全行程间隙" class="DigNum (严格)"("Visible"=w1638) -> ()  [unwired: 2 in, 2 out]
                n914 = property on="右180°外全行程间隙" class="DigNum (严格)"("Visible"=w1638) -> ()  [unwired: 2 in, 2 out]
                n915 = property on="右180°内全行程间隙" class="DigNum (严格)"("Visible"=w1638) -> ()  [unwired: 2 in, 2 out]
                n916 = property on="左全行程间隙" class="DigNum (严格)"("Visible"=w1637) -> ()  [unwired: 2 in, 2 out]
                n917 = property on="右全行程间隙" class="DigNum (严格)"("Visible"=w1637) -> ()  [unwired: 2 in, 2 out]
              }
            }
          }
          frame #1 {
            (unwired) string[] ["I急停按钮", "I自动旋钮", "I启动按钮", "I备用按钮", "I复位按钮", "I上阻挡器放行", "I下阻挡器放行", "I进支线按钮"] ("I0说明")
            (unwired) string[] ["I出支线按钮", "I主线顶升按钮", "I主线下降按钮", "I支线顶升按钮", "I支线下降按钮", "I气压报警", "未使用", "未使用"] ("I0说明")
            n918 = local read "间隙位移(mm)"() -> (w1641:dbl)
            n919 = Greater Or Equal?(x=w1641, y=7.0) -> (x >= y?=w1639:bool)
            n920 = case shown="真" w1639 {
              frame False {
              }
              frame True {
                n921 = local write "测头机构轴使能"(FALSE ("测头机构轴使能")) -> ()
              }
            }
          }
          frame #2 {
            (unwired) string[] ["I电动缸SRDY", "I电动缸ZSPD", "I电动缸ALRM", "I间隙进给SRDY", "I间隙进给ZSPD", "I间隙进给ALRM", "I间隙旋转SRPD", "I间隙旋转ZSPD"] ("I0说明")
            n922 = local read "测头机构轴位置(mm)"() -> (w1645:dbl)
            n923 = Greater Or Equal?(x=w1645, y=90.0) -> (x >= y?=w1643:bool)
            n924 = case shown="假" w1643 {
              frame False {
                w1646 = T5."Enabled" ("禁用")
                n925 = property on="测头气缸左移" class="Bool (严格)"("DisabledEnum"=w1646) -> ()  [unwired: 2 in, 2 out]
                n926 = property on="测头气缸右移" class="Bool (严格)"("DisabledEnum"=w1646) -> ()  [unwired: 2 in, 2 out]
                n927 = property on="测头气缸左移" class="Bool"("DisabledEnum"=w1646) -> ()  [unwired: 2 in, 2 out]
                n928 = property on="测头气缸右移" class="Bool"("DisabledEnum"=w1646) -> ()  [unwired: 2 in, 2 out]
              }
              frame True {
                w1647 = T5."Disabled" ("禁用")
                w1648 = FALSE ("测头气缸右移")
                n929 = local write "测头气缸右移"(w1648) -> ()
                n930 = local write "测头气缸左移"(w1648) -> ()
                n931 = property on="测头气缸左移" class="Bool (严格)"("DisabledEnum"=w1647) -> ()  [unwired: 2 in, 2 out]
                n932 = property on="测头气缸右移" class="Bool (严格)"("DisabledEnum"=w1647) -> ()  [unwired: 2 in, 2 out]
                n933 = property on="测头气缸左移" class="Bool"("DisabledEnum"=w1647) -> ()  [unwired: 2 in, 2 out]
                n934 = property on="测头气缸右移" class="Bool"("DisabledEnum"=w1647) -> ()  [unwired: 2 in, 2 out]
              }
            }
          }
          frame #3 {
            (unwired) string[] ["I间隙旋转ALRM", "I扭矩旋转SRPD", "I扭矩旋转ZSPD", "I扭矩旋转ALRM", "I拧紧机合格", "I拧紧机不合格", "I拧紧机报警", "未使用"] ("I0说明")
          }
        }
      }
      frame #2 {
        n935 = flat-sequence {
          frame #0 {
            (unwired) string[] ["I自制气缸进位", "I自制气缸原位", "I上工位检测", "I本工位检测", "I下工位检测", "I主线顶升上位", "I主线顶升下位", "I支线顶升上位"] ("I0说明")
          }
          frame #1 {
            (unwired) string[] ["I支线顶升下位", "I支线进到位", "I支线退到位", "I位移气缸原位", "I位移气缸进位", "I拧紧机在位", "I电动缸原位", "I电动缸进位"] ("I0说明")
          }
          frame #2 {
            (unwired) string[] ["未使用", "未使用", "未使用", "未使用", "未使用", "未使用", "未使用", "未使用"] ("I0说明")
          }
          frame #3 {
            (unwired) string[] ["未使用", "未使用", "未使用", "未使用", "未使用", "未使用", "未使用", "未使用"] ("I0说明")
          }
        }
        n936 = local read "下工位测试H"() -> (w1650:bool)
        n937 = local read "下工位备料H"() -> (w1649:bool)
        n938 = local read "下工位自动H"() -> (w1651:bool)
        n939 = local write "下工位备料"(w1649) -> ()
        n940 = local write "下工位测试"(w1650) -> ()
        n941 = local write "下工位自动"(w1651) -> ()
      }
      frame #3 {
        n942 = local read "工步号"() -> (w1655:u32)
        n943 = local read "报警"() -> (w1653:dbl)
        n944 = case shown="50" w1655 {
          tunnel: [w1666 "请取胶瓶" ("工步描述") "请取扳手加力" ("工步描述") "灵敏度测试中" ("工步描述") "有油刚度测试中" ("工步描述") "点击启动按钮进行测试" ("工步描述") "电动缸前进找中" ("工步描述") "气缸右移" ("工步描述") "电动缸前进找中" ("工步描述") "找中结束开始测间隙" ("工步描述") "力特性试验中" ("工步描述") "轴向力测试中" ("工步描述") "探头气缸左移，电动缸后退" ("工步描述") "等待放行" ("工步描述") "电动缸回零" ("工步描述") "力特性试验完成" ("工步描述") "套好输出轴把手，按启动按钮，做回正力试验" ("工步描述") "回正力试验中" ("工步描述") "试验完成，将把手拉回，取下油管，按顶升按钮" ("工步描述") "拆下锁紧螺母和输入轴万向节，按顶升按钮" ("工步描述")] -> w1654
          frame 0, Default {
            n945 = local read "联线按钮"() -> (w1665:bool)
            n946 = case shown="假" w1665 {
              tunnel: ["等待工件" ("工步描述") "等待扫描条码" ("工步描述")] -> w1666
              frame False {
              }
              frame True {
              }
            }
          }
          frame 1 {
          }
          frame 2 {
          }
          frame 3 {
          }
          frame 4 {
          }
          frame 6 {
          }
          frame 7 {
          }
          frame 10 {
          }
          frame 15 {
          }
          frame 20 {
          }
          frame 30 {
          }
          frame 40 {
          }
          frame 45 {
          }
          frame 100 {
          }
          frame 50 {
          }
          frame 55 {
          }
          frame 60 {
          }
          frame 70 {
          }
          frame 80 {
          }
          frame 56 {
          }
        }
        "工步提示" <- w1654
        n947 = case shown="9" w1653 {
          tunnel: [_ "探头气缸不在原位" "操作步骤错误请取胶瓶" "操作步骤错误请加力" "急停被按下" "气压报警" "电动缸伺服报警" "旋转伺服报警" "测头伺服报警" "操作步骤错误请点标后放行"] -> w1652
          frame 0, Default {
          }
          frame 1 {
          }
          frame 2 {
          }
          frame 3 {
          }
          frame 4 {
          }
          frame 5 {
          }
          frame 6 {
          }
          frame 7 {
          }
          frame 8 {
          }
          frame 9 {
          }
        }
        n948 = local write "报警提示"(w1652) -> ()
      }
      frame #4 {
        n949 = local read "急停"() -> (w1688:bool)
        n950 = local read "红灯"() -> (w1690:bool)
        n951 = local read "复位"() -> (w1691:bool)
        n952 = local read "复位"() -> (w1693:bool)
        n953 = local read "红灯"() -> (w1692:bool)
        n954 = case shown="真" w1688 {
          frame False {
            "红灯" <- TRUE ("红灯")
          }
          frame True {
            n955 = local write "红灯"(FALSE ("红灯")) -> ()
          }
        }
        n956 = Or(x=w1690, y=w1691) -> (x .or. y?=w1689:bool)
        n957 = case shown="真" w1689 {
          frame False {
          }
          frame True {
            n958 = local write "回零完成"(FALSE ("夹头夹紧控制")) -> ()
          }
        }
        n959 = local read "停止"() -> (w1695:bool)
        n960 = Compound Arithmetic op=OR(w1693, w1695, w1692) -> (w1694:bool)
        n961 = case shown="真" w1694 {
          frame False {
          }
          frame True {
            n962 = local read "测头机构电机"() -> (w1699:u32)
            n963 = local read "旋转齿条电机"() -> (w1700:u32)
            n964 = local read "电动缸电机"() -> (w1701:u32)
            n965 = call "PCI1220U停止.vi"("AxisHandle IN"=w1700) -> ()  [unwired: 9 in, 2 out]
            n966 = call "PCI1220U停止.vi"("AxisHandle IN"=w1701) -> ()  [unwired: 9 in, 2 out]
            n967 = call "PCI1220U停止.vi"("AxisHandle IN"=w1699) -> ()  [unwired: 9 in, 2 out]
          }
        }
      }
      frame #5 {
        n968 = local read "齿条扭矩(Nm)"() -> (w1704:dbl)
        n969 = local read "黄灯"() -> (w1702:bool)
        n970 = local read "旋转齿条轴左转"() -> (w1710:bool)
        n971 = Absolute Value(x=w1704) -> (abs(x)=w1709:dbl)
        n972 = local read "旋转齿条轴右转"() -> (w1705:bool)
        n973 = Not(x=w1710) -> (.not. x?=w1706:bool)
        n974 = Less?(x=w1709, y=20.0) -> (x < y?=w1707:bool)
        n975 = Compound Arithmetic op=AND(w1705, w1706, w1707, w1702) -> (w1703:bool)
        n976 = case shown="真" w1703 {
          frame False {
          }
          frame True {
            n977 = flat-sequence {
              tunnel: [w1714] -> w1712
              tunnel: w1712 -> [w1716]
              tunnel: [w1716] -> w1711
              tunnel: w1711 -> [w1727]
              frame #0 {
                n978 = local read "旋转齿条电机"() -> (w1713:u32)
                n979 = call "PCI1220U运行.vi"("方向"=enum32{"Negative", "Positive"}."Negative" ("Direction"), "AxisHandle IN"=w1713) -> ("AxisHandle OUT"=w1714:u32)  [unwired: 9 in]
              }
              frame #1 {
                n980 = while {
                  stop <- w1720 stop-if-true
                  n981 = Wait (ms)(milliseconds to wait=u32 50 ("毫秒倍数")) -> ()  [unwired: 1 out]
                  n982 = local read "齿条扭矩(Nm)"() -> (w1725:dbl)
                  n983 = local read "旋转齿条轴右转"() -> (w1722:bool)
                  n984 = local read "红灯"() -> (w1717:bool)
                  n985 = local read "复位"() -> (w1718:bool)
                  n986 = Absolute Value(x=w1725) -> (abs(x)=w1724:dbl)
                  n987 = Not(x=w1722) -> (.not. x?=w1719:bool)
                  n988 = Greater?(x=w1724, y=10.0) -> (0:w1721:bool)
                  n989 = Compound Arithmetic op=OR(w1721, w1719, w1718, w1717) -> (w1720:bool)
                }
              }
              frame #2 {
                n990 = call "PCI1220U停止.vi"("AxisHandle IN"=w1727) -> ()  [unwired: 9 in, 2 out]
              }
            }
          }
        }
      }
      frame #6 {
        n991 = local read "齿条扭矩(Nm)"() -> (w1732:dbl)
        n992 = local read "旋转齿条轴右转"() -> (w1736:bool)
        n993 = Absolute Value(x=w1732) -> (abs(x)=w1731:dbl)
        n994 = local read "旋转齿条轴左转"() -> (w1734:bool)
        n995 = local read "黄灯"() -> (w1728:bool)
        n996 = Not(x=w1736) -> (.not. x?=w1733:bool)
        n997 = Less?(x=w1731, y=20.0) -> (x < y?=w1729:bool)
        n998 = Compound Arithmetic op=AND(w1734, w1733, w1729, w1728) -> (w1735:bool)
        n999 = case shown="真" w1735 {
          frame False {
          }
          frame True {
            n1000 = flat-sequence {
              tunnel: [w1740] -> w1738
              tunnel: w1738 -> [w1742]
              tunnel: [w1742] -> w1737
              tunnel: w1737 -> [w1753]
              frame #0 {
                n1001 = local read "旋转齿条电机"() -> (w1739:u32)
                n1002 = call "PCI1220U运行.vi"("方向"=enum32{"Negative", "Positive"}."Positive" ("Direction"), "AxisHandle IN"=w1739) -> ("AxisHandle OUT"=w1740:u32)  [unwired: 9 in]
              }
              frame #1 {
                n1003 = while {
                  stop <- w1745 stop-if-true
                  n1004 = Wait (ms)(milliseconds to wait=u32 50 ("毫秒倍数")) -> ()  [unwired: 1 out]
                  n1005 = local read "齿条扭矩(Nm)"() -> (w1751:dbl)
                  n1006 = local read "旋转齿条轴左转"() -> (w1748:bool)
                  n1007 = local read "红灯"() -> (w1743:bool)
                  n1008 = local read "复位"() -> (w1744:bool)
                  n1009 = Absolute Value(x=w1751) -> (abs(x)=w1750:dbl)
                  n1010 = Not(x=w1748) -> (.not. x?=w1746:bool)
                  n1011 = Greater?(x=w1750, y=10.0) -> (0:w1747:bool)
                  n1012 = Compound Arithmetic op=OR(w1744, w1743, w1747, w1746) -> (w1745:bool)
                }
              }
              frame #2 {
                n1013 = call "PCI1220U停止.vi"("AxisHandle IN"=w1753) -> ()  [unwired: 9 in, 2 out]
              }
            }
          }
        }
      }
      frame #7 {
        n1014 = local read "齿条推拉力(N)"() -> (w1758:dbl)
        n1015 = local read "电动缸前进"() -> (w1755:bool)
        n1016 = local read "电动缸后退"() -> (w1754:bool)
        n1017 = Absolute Value(x=w1758) -> (abs(x)=w1762:dbl)
        n1018 = local read "黄灯"() -> (w1756:bool)
        n1019 = Not(x=w1754) -> (.not. x?=w1759:bool)
        n1020 = Less?(x=w1762, y=1000.0) -> (x < y?=w1760:bool)
        n1021 = Compound Arithmetic op=AND(w1755, w1759, w1756, w1760) -> (w1757:bool)
        n1022 = case shown="真" w1757 {
          frame False {
          }
          frame True {
            n1023 = flat-sequence {
              tunnel: [w1766] -> w1764
              tunnel: w1764 -> [w1768]
              tunnel: [w1768] -> w1763
              tunnel: w1763 -> [w1779]
              frame #0 {
                n1024 = local read "电动缸电机"() -> (w1765:u32)
                n1025 = call "PCI1220U运行.vi"("方向"=enum32{"Negative", "Positive"}."Positive" ("Direction"), "AxisHandle IN"=w1765) -> ("AxisHandle OUT"=w1766:u32)  [unwired: 9 in]
              }
              frame #1 {
                n1026 = while {
                  stop <- w1776 stop-if-true
                  n1027 = local read "电动缸前进"() -> (w1773:bool)
                  n1028 = local read "齿条推拉力(N)"() -> (w1770:dbl)
                  n1029 = Wait (ms)(milliseconds to wait=u32 50 ("毫秒倍数")) -> ()  [unwired: 1 out]
                  n1030 = Absolute Value(x=w1770) -> (abs(x)=w1772:dbl)
                  n1031 = local read "红灯"() -> (w1774:bool)
                  n1032 = local read "复位"() -> (w1775:bool)
                  n1033 = Greater?(x=w1772, y=1000.0) -> (0:w1769:bool)
                  n1034 = Not(x=w1773) -> (.not. x?=w1777:bool)
                  n1035 = Compound Arithmetic op=OR(w1775, w1774, w1777, w1769) -> (w1776:bool)
                }
              }
              frame #2 {
                n1036 = call "PCI1220U停止.vi"("AxisHandle IN"=w1779) -> ()  [unwired: 9 in, 2 out]
              }
            }
          }
        }
      }
      frame #8 {
        n1037 = local read "电动缸前进"() -> (w1780:bool)
        n1038 = local read "齿条推拉力(N)"() -> (w1784:dbl)
        n1039 = local read "电动缸后退"() -> (w1781:bool)
        n1040 = Absolute Value(x=w1784) -> (abs(x)=w1788:dbl)
        n1041 = local read "黄灯"() -> (w1782:bool)
        n1042 = Not(x=w1780) -> (.not. x?=w1785:bool)
        n1043 = Less?(x=w1788, y=1000.0) -> (x < y?=w1786:bool)
        n1044 = Compound Arithmetic op=AND(w1781, w1785, w1782, w1786) -> (w1783:bool)
        n1045 = case shown="真" w1783 {
          frame False {
          }
          frame True {
            n1046 = flat-sequence {
              tunnel: [w1792] -> w1790
              tunnel: w1790 -> [w1794]
              tunnel: [w1794] -> w1789
              tunnel: w1789 -> [w1805]
              frame #0 {
                n1047 = local read "电动缸电机"() -> (w1791:u32)
                n1048 = call "PCI1220U运行.vi"("方向"=enum32{"Negative", "Positive"}."Negative" ("Direction"), "AxisHandle IN"=w1791) -> ("AxisHandle OUT"=w1792:u32)  [unwired: 9 in]
              }
              frame #1 {
                n1049 = while {
                  stop <- w1802 stop-if-true
                  n1050 = local read "电动缸后退"() -> (w1799:bool)
                  n1051 = local read "齿条推拉力(N)"() -> (w1798:dbl)
                  n1052 = Wait (ms)(milliseconds to wait=u32 50 ("毫秒倍数")) -> ()  [unwired: 1 out]
                  n1053 = Absolute Value(x=w1798) -> (abs(x)=w1796:dbl)
                  n1054 = local read "红灯"() -> (w1801:bool)
                  n1055 = local read "复位"() -> (w1800:bool)
                  n1056 = Greater?(x=w1796, y=1000.0) -> (0:w1795:bool)
                  n1057 = Not(x=w1799) -> (.not. x?=w1803:bool)
                  n1058 = Compound Arithmetic op=OR(w1800, w1801, w1803, w1795) -> (w1802:bool)
                }
              }
              frame #2 {
                n1059 = call "PCI1220U停止.vi"("AxisHandle IN"=w1805) -> ()  [unwired: 9 in, 2 out]
              }
            }
          }
        }
      }
      frame #9 {
        n1060 = local read "测头机构轴后退"() -> (w1806:bool)
        n1061 = local read "测头机构轴前进"() -> (w1807:bool)
        n1062 = local read "黄灯"() -> (w1808:bool)
        n1063 = Not(x=w1806) -> (.not. x?=w1810:bool)
        n1064 = Compound Arithmetic op=AND(w1807, w1810, w1808) -> (w1809:bool)
        n1065 = case shown="真" w1809 {
          frame False {
          }
          frame True {
            n1066 = flat-sequence {
              tunnel: [w1814] -> w1812
              tunnel: w1812 -> [w1816]
              tunnel: [w1816] -> w1811
              tunnel: w1811 -> [w1823]
              frame #0 {
                n1067 = local read "测头机构电机"() -> (w1813:u32)
                n1068 = call "PCI1220U运行.vi"("方向"=enum32{"Negative", "Positive"}."Positive" ("Direction"), "AxisHandle IN"=w1813) -> ("AxisHandle OUT"=w1814:u32)  [unwired: 9 in]
              }
              frame #1 {
                n1069 = while {
                  stop <- w1820 stop-if-true
                  n1070 = local read "测头机构轴前进"() -> (w1817:bool)
                  n1071 = Wait (ms)(milliseconds to wait=u32 50 ("毫秒倍数")) -> ()  [unwired: 1 out]
                  n1072 = local read "红灯"() -> (w1818:bool)
                  n1073 = local read "复位"() -> (w1819:bool)
                  n1074 = Not(x=w1817) -> (.not. x?=w1821:bool)
                  n1075 = Compound Arithmetic op=OR(w1819, w1818, w1821) -> (w1820:bool)
                }
              }
              frame #2 {
                n1076 = call "PCI1220U停止.vi"("AxisHandle IN"=w1823) -> ()  [unwired: 9 in, 2 out]
              }
            }
          }
        }
      }
      frame #10 {
        n1077 = local read "测头机构轴前进"() -> (w1824:bool)
        n1078 = local read "测头机构轴后退"() -> (w1825:bool)
        n1079 = local read "黄灯"() -> (w1826:bool)
        n1080 = Not(x=w1824) -> (.not. x?=w1828:bool)
        n1081 = Compound Arithmetic op=AND(w1825, w1828, w1826) -> (w1827:bool)
        n1082 = case shown="真" w1827 {
          frame False {
          }
          frame True {
            n1083 = flat-sequence {
              tunnel: [w1832] -> w1830
              tunnel: w1830 -> [w1834]
              tunnel: [w1834] -> w1829
              tunnel: w1829 -> [w1841]
              frame #0 {
                n1084 = local read "测头机构电机"() -> (w1831:u32)
                n1085 = call "PCI1220U运行.vi"("方向"=enum32{"Negative", "Positive"}."Negative" ("Direction"), "AxisHandle IN"=w1831) -> ("AxisHandle OUT"=w1832:u32)  [unwired: 9 in]
              }
              frame #1 {
                n1086 = while {
                  stop <- w1838 stop-if-true
                  n1087 = local read "测头机构轴后退"() -> (w1835:bool)
                  n1088 = Wait (ms)(milliseconds to wait=u32 50 ("毫秒倍数")) -> ()  [unwired: 1 out]
                  n1089 = local read "红灯"() -> (w1837:bool)
                  n1090 = local read "复位"() -> (w1836:bool)
                  n1091 = Not(x=w1835) -> (.not. x?=w1839:bool)
                  n1092 = Compound Arithmetic op=OR(w1836, w1837, w1839) -> (w1838:bool)
                }
              }
              frame #2 {
                n1093 = call "PCI1220U停止.vi"("AxisHandle IN"=w1841) -> ()  [unwired: 9 in, 2 out]
              }
            }
          }
        }
      }
    }
    n1094 = Wait (ms)(milliseconds to wait=u32 50 ("毫秒倍数")) -> ()  [unwired: 1 out]
    n1095 = local read "停止"() -> (w1628:bool)
  }
  n1096 = flat-sequence {
    tunnel: [w1845] -> w2
    tunnel: [w1843] -> w1
    tunnel: w2 -> [w1855]
    tunnel: w1 -> [w1854]
    frame #0 {
      n1097 = First Call?() -> (First Call?: T/F=w1842:bool)
      n1098 = case shown="真" w1842 {
        frame False {
        }
        frame True {
          n1099 = while {
            i -> [w1849]
            stop <- w1850 stop-if-true
            w1853 = TRUE ("电动缸使能")
            n1100 = Wait Until Next ms Multiple(millisecond multiple=u32 50 ("毫秒倍数")) -> ()  [unwired: 1 out]
            n1101 = local write "回零完成"(FALSE ("回零完成")) -> ()
            n1102 = local write "测头机构轴使能"(w1853) -> ()
            n1103 = local write "旋转齿条轴使能"(w1853) -> ()
            n1104 = local write "电动缸使能"(w1853) -> ()
            n1105 = Greater Or Equal?(x=w1849, y=u32 30) -> (x >= y?=w1850:bool)
          }
        }
      }
      n1106 = call "ADO Connection Create.vi"() -> ("error out"=w1846:errorcluster, "ADODB._Connection Out"=w1847:refnum<k7>)  [unwired: 10 in]
      n1107 = call "ADO Connection Open.vi"("error in (no error)"=w1846, "ConnectionString"="Provider=Microsoft.Jet.OLEDB.4.0;Data Source=D:\\Q14070-Z060人机界面\\参数\\参数Z060.mdb;Persist Security Info=False;Jet OLEDB:Database Password=123;", "ADODB._Connection In"=w1847) -> ("error out"=w1843:errorcluster, "ADODB._Connection Out"=w1845:refnum<k7>)  [unwired: 7 in]
    }
    frame #1 {
      n1108 = while {
        tunnel: w1855 -> [w1857]
        tunnel: w1854 -> [w1856]
        stop <- w1861 stop-if-true
        n1109 = Wait (ms)(milliseconds to wait=u32 50 ("等待时间（毫秒）")) -> ()  [unwired: 1 out]
        n1110 = First Call?() -> (First Call?: T/F=w1860:bool)
        n1111 = Or(x=w1860, y="参数加载") -> (x .or. y?=w1859:bool)
        n1112 = case shown="真" w1859 {
          tunnel: w1857 -> [_ w1864]
          tunnel: w1856 -> [_ w1863]
          frame False {
          }
          frame True {
            n1113 = stacked-sequence {
              tunnel: w1864 -> [w1870 w1919 w1938]
              tunnel: w1863 -> [w1865 _ _]
              frame #0 {
                n1114 = call "SQL Execute.vi"("error in (no error)"=w1865, "Command Text"="SELECT * FROM 测试参数表", "ADODB._Connection In"=w1870) -> ("Data"=w1868:string[][])  [unwired: 5 in, 3 out]
                n1115 = Index Array(array=w1868, index (col)=0 ("索引 (行)")) -> (element=w1872:string[])  [unwired: 1 in]
                n1116 = Array Size(array=w1872) -> (size(s)=w1867:i32)
                "型号数量" <- w1867
                n1117 = while {
                  shift-right: [w1879] -> w1871
                  shift-left: i32[] [] -> [w1878]
                  tunnel: w1867 -> [w1876]
                  i -> [w1877]
                  stop <- w1875 stop-if-true
                  n1118 = Greater Or Equal?(x=w1877, y=w1876) -> (x >= y?=w1875:bool)
                  n1119 = Build Array (concatenate)(w1878, w1877) -> (w1879:i32[])
                }
                n1120 = Build Cluster Array "索引与捆绑簇数组"(w1872, w1871) -> (w1866:cluster{"String":string, i32}[])
                n1121 = property on="型号选择" class="Ring (严格)"("StringsAndValues[]"=w1866) -> ()  [unwired: 2 in, 2 out]
              }
              frame #1 {
                n1122 = property on="型号选择" class="Ring (严格)"() -> ("RingText.Text"=w1920:string)  [unwired: 2 in, 2 out]
                n1123 = call "创建文本2"("型号选择"=w1920) -> ("Result"=w1924:string)  [unwired: 13 in, 1 out]
                n1124 = call "SQL Execute.vi"("Command Text"=w1924, "ADODB._Connection In"=w1919) -> ("Data"=w1923:string[][])  [unwired: 6 in, 3 out]
                n1125 = Index Array(array=w1923, index (row)=0 ("索引 (行)")) -> (element=w1921:string[])  [unwired: 1 in]
                n1126 = Fract/Exp String To Number ("分数/指数字符串至数值转换")(string=w1921) -> (number=w1908:dbl[])  [unwired: 3 in, 1 out]
                n1127 = Index Array ("索引数组")(array=w1908, index #1=2 ("索引"), index #2=3 ("索引"), index #3=4 ("索引"), index #4=5 ("索引"), index #5=6 ("索引"), index #6=7 ("索引"), index #7=8 ("索引"), index #8=9 ("索引"), index #9=10 ("索引"), index #10=11 ("索引"), index #11=12 ("索引"), index #12=13 ("索引"), index #13=14 ("索引"), index #14=15 ("索引"), index #15=16 ("索引"), index #16=17 ("索引"), index #17=18 ("索引"), index #18=19 ("索引"), index #19=20 ("索引")) -> (element #1=w1907:dbl, element #2=w1906:dbl, element #3=w1905:dbl, element #4=w1904:dbl, element #5=w1903:dbl, element #6=w1902:dbl, element #7=w1901:dbl, element #8=w1900:dbl, element #9=w1899:dbl, element #10=w1898:dbl, element #11=w1897:dbl, element #12=w1896:dbl, element #13=w1880:dbl, element #14=w1890:dbl, element #15=w1889:dbl, element #16=w1888:dbl, element #17=w1884:dbl, element #18=w1883:dbl, element #19=w1881:dbl)
                n1128 = local write "测头机构轴移动速度"(w1907) -> ()
                n1129 = local write "测头机构轴检测位"(w1906) -> ()
                n1130 = local write "测头机构轴后退位"(w1904) -> ()
                n1131 = local write "测头机构轴待检位"(w1905) -> ()
                n1132 = local write "旋转伺服找帽转速"(w1900) -> ()
                n1133 = local write "旋转伺服测量转速"(w1899) -> ()
                n1134 = local write "总行程标准(mm)"(w1897) -> ()
                n1135 = local write "齿条移动速度"(w1903) -> ()
                n1136 = local write "平均轴向力MAX(N)"(w1888) -> ()
                n1137 = local write "齿条左极限"(w1902) -> ()
                n1138 = local write "总行程最大值"(w1896) -> ()
                n1139 = local write "齿条右极限"(w1901) -> ()
                n1140 = local write "转向器中心"(w1881) -> ()
                n1141 = local write "总圈数标准"(w1884) -> ()
                n1142 = local write "总圈数最大值"(w1883) -> ()
                n1143 = local write "测量点扭矩"(w1898) -> ()
                n1144 = local write "力波动标准(N)"(w1890) -> ()
                n1145 = local write "轴向力标准(N)"(w1889) -> ()
                n1146 = local write "齿条传动比"(w1880) -> ()
              }
              frame #2 {
                n1147 = call "SQL Execute.vi"("Command Text"="SELECT * FROM 传感器校验表 where ID='1'", "ADODB._Connection In"=w1938) -> ("Data"=w1940:string[][])  [unwired: 6 in, 3 out]
                n1148 = Index Array(array=w1940) -> (element=w1941:string[])  [unwired: 2 in]
                n1149 = Fract/Exp String To Number ("分数/指数字符串至数值转换")(string=w1941) -> (number=w1931:dbl[])  [unwired: 3 in, 1 out]
                n1150 = Index Array(array=w1931, index #1=1 ("索引"), index #2=2 ("索引"), index #3=3 ("索引"), index #4=4 ("索引"), index #5=5 ("索引"), index #6=6 ("索引")) -> (element #1=w1930:dbl, element #2=w1929:dbl, element #3=w1928:dbl, element #4=w1927:dbl, element #5=w1926:dbl, element #6=w1925:dbl)
                n1151 = local write "间隙位移零点偏移"(w1930) -> ()
                n1152 = local write "间隙位移比例偏移"(w1929) -> ()
                n1153 = local write "齿条推拉力零点偏移"(w1928) -> ()
                n1154 = local write "齿条推拉力比例偏移"(w1927) -> ()
                n1155 = local write "齿条扭矩零点偏移"(w1926) -> ()
                n1156 = local write "齿条扭矩比例偏移"(w1925) -> ()
              }
            }
          }
        }
        n1157 = local read "停止"() -> (w1861:bool)
        "ADODB._Connection Out 2" <- w1857
      }
    }
  }
  n1158 = while {
    stop <- w1943 stop-if-true
    n1159 = local read "rfid工步号"() -> (w1942:u32)
    n1160 = case shown="10" w1942 {
      frame 0, Default {
      }
      frame 10 {
        n1161 = flat-sequence {
          tunnel: [w1953] -> w1947
          tunnel: w1947 -> [w1957]
          tunnel: [w1954] -> w1946
          tunnel: w1946 -> [w1959]
          tunnel: [w1959] -> w1945
          tunnel: w1945 -> [w1962]
          frame #0 {
            n1162 = while {
              stop <- w1948 stop-if-true
              n1163 = local read "rfid触发"() -> (w1948:bool)
              n1164 = Wait Until Next ms Multiple(millisecond multiple=u32 50 ("毫秒倍数")) -> ()  [unwired: 1 out]
            }
          }
          frame #1 {
            n1165 = local write "芯片ID"("" ("随行板ID")) -> ()
            n1166 = local write "rfid完成"(FALSE ("RFID完成")) -> ()
            n1167 = local write "rfid触发"(FALSE ("RFID读取触发")) -> ()
          }
          frame #2 {
            n1168 = local read "Z060ARFID"() -> (w1953:string)
            n1169 = local write "芯片ID"(w1953) -> ()
          }
          frame #3 {
            w1955 = T6 0 items=["两端", "字符串首端", "字符串末端"] ("location (both)")
            n1170 = call "查询产品ID.vi"("芯片编码"=w1957) -> ("产品ID"=w1956:string)  [unwired: 8 in, 2 out]
            "读取产品ID" <- w1956
            n1171 = call <vilib>:"Trim Whitespace.vi"("string"=w1956, "location (both)"=w1955) -> ("trimmed string"=w1954:string)
          }
          frame #4 {
            n1172 = Wait Until Next ms Multiple(millisecond multiple=u32 500 ("毫秒倍数")) -> ()  [unwired: 1 out]
          }
          frame #5 {
            n1173 = call "查询上序合格.vi"("产品ID"=w1962) -> ("本序已做"=w1960:bool, "上序合格"=w1961:bool)  [unwired: 8 in, 1 out]
            n1174 = Not(x=w1961) -> (.not. x?=w1963:bool)
            n1175 = local write "上序不合格"(w1963) -> ()
            n1176 = local write "上序合格"(w1961) -> ()
            n1177 = local write "本序已做"(w1960) -> ()
          }
          frame #6 {
            n1178 = local write "rfid完成"(TRUE ("RFID读取完成")) -> ()
            n1179 = Wait Until Next ms Multiple(millisecond multiple=u32 500 ("毫秒倍数")) -> ()  [unwired: 1 out]
          }
          frame #7 {
            "rfid工步号" <- 15.0 ("工步号")
          }
        }
      }
      frame 210 {
        n1180 = local read "读取产品ID"() -> (w1967:string)
        n1181 = local write "产品ID"(w1967) -> ()
      }
    }
    n1182 = Wait Until Next ms Multiple(millisecond multiple=u32 50 ("毫秒倍数")) -> ()  [unwired: 1 out]
    n1183 = local read "停止"() -> (w1943:bool)
  }
  n1184 = flat-sequence {
    tunnel: [w1968] -> w4
    tunnel: w4 -> [w1974]
    tunnel: [w1973] -> w3
    tunnel: w3 -> [w2044]
    frame #0 {
      n1185 = call "PCI1240U初始化.vi"() -> ("旋转电机"=→"旋转齿条电机":u32, "电动缸电机"=→"电动缸电机":u32, "DeviceHandle"=→"DeviceHandle":u32, "进给电机"=→"测头机构电机":u32)  [unwired: 6 in, 2 out]
      n1186 = call "PCI8622配置.vi"() -> ("DeviceID"=w1968:i32)  [unwired: 11 in]
    }
    frame #1 {
      n1187 = while {
        tunnel: w1974 -> [w1976]
        tunnel: [w1975] -> w1973
        stop <- "停止" stop-if-true
        n1188 = stacked-sequence {
          tunnel: w1976 -> [_ _ w2020]
          tunnel: [_ _ w2020] -> w1975
          frame #0 {
            n1189 = local read "测头机构电机"() -> (w1985:u32)
            n1190 = Boolean To (0,1)(Boolean="测头机构轴使能") -> (0, 1=w1983:i16)
            n1191 = call <userlib>:"Acm_AxSetSvOn.vi"("OnOff"=w1983, "AxisHandle"=w1985) -> ("AxisHandle"=w1982:u32)  [unwired: 1 in, 2 out]
            n1192 = call "PCI1220U进给轴速度设置.vi"("Change Velocity"="测头机构轴速度(mm/s)", "AxisHandle IN"=w1982) -> ("AxisHandle OUT"=w1980:u32)  [unwired: 9 in]
            n1193 = call "PCI1220U进给轴读取位置.vi"("AxisHandle IN"=w1980) -> ("位置"=→"测头机构轴位置(mm)":dbl)  [unwired: 9 in, 1 out]
          }
          frame #1 {
            n1194 = local read "电动缸电机"() -> (w1995:u32)
            n1195 = local read "旋转齿条电机"() -> (w1994:u32)
            n1196 = Boolean To (0,1)(Boolean="电动缸使能") -> (0, 1=w1999:i16)
            n1197 = Boolean To (0,1)(Boolean="旋转齿条轴使能") -> (0, 1=w1993:i16)
            n1198 = call <userlib>:"Acm_AxSetSvOn.vi"("OnOff"=w1993, "AxisHandle"=w1994) -> ("AxisHandle"=w1996:u32)  [unwired: 1 in, 2 out]
            n1199 = call <userlib>:"Acm_AxSetSvOn.vi"("OnOff"=w1999, "AxisHandle"=w1995) -> ("AxisHandle"=w1998:u32)  [unwired: 1 in, 2 out]
            n1200 = call "PCI1220U扭矩轴速度设置.vi"("Change Velocity"="旋转伺服速度(°/s)", "AxisHandle IN"=w1996) -> ("AxisHandle OUT"=w1997:u32)  [unwired: 9 in]
            n1201 = call "PCI1240电动缸速度设置.vi"("Change Velocity"="电动缸速度(mm/s)", "AxisHandle IN"=w1998) -> ("AxisHandle OUT"=w1986:u32)  [unwired: 9 in]
            n1202 = call "PCI1220U扭矩轴读取位置.vi"("AxisHandle IN"=w1997) -> ("位置"=→"旋转伺服位置(°)":dbl)  [unwired: 9 in, 1 out]
            n1203 = call "PCI1240电动缸读取位置.vi"("AxisHandle IN"=w1986) -> ("位置"=→"电动缸位置(mm)":dbl)  [unwired: 9 in, 1 out]
          }
          frame #2 {
            w2036 = 0  # nRetSizeWords
            w2037 = 2048  # nReadSizeWords
            # "hDevice"
            n1204 = Initialize Array(u16 0, 2048 ("dimension size")) -> (w2027:u16[])
            n1205 = dll-call lib="PCI8622_32.dll" fn="PCI8622_ReadDeviceProAD_Npt" label="ReadDeviceProAD_Npt"("hDevice"=w2020, "ADBuffer[]"=w2027, "nReadSizeWords"=w2037, "nRetSizeWords"=w2036) -> ("ADBuffer[]"=w2030:u16[])  [unwired: 7 in, 2 out]
            n1206 = Divide(x=w2030, y=65536.01) -> (x/y=w2031:dbl[])
            n1207 = Multiply(x=w2031, y=20) -> (x*y=w2034:dbl[])
            n1208 = Subtract(x=w2034, y=10) -> (x-y=w2026:dbl[])
            n1209 = Decimate 1D Array ("抽取一维数组")(w2026) -> (w2014:dbl[], w2015:dbl[], w2013:dbl[])  [unwired: 5 out]
            n1210 = Add Array Elements(numeric array=w2014) -> (sum=w2023:dbl)
            n1211 = Add Array Elements(numeric array=w2013) -> (sum=w2024:dbl)
            n1212 = Array Size(array=w2014) -> (size(s)=w2022:i32)
            n1213 = Add Array Elements(numeric array=w2015) -> (sum=w2019:dbl)
            n1214 = Array Size(array=w2013) -> (size(s)=w2025:i32)
            n1215 = Array Size(array=w2015) -> (size(s)=w2021:i32)
            n1216 = Divide(x=w2023, y=w2022) -> (x/y=w2012:dbl)
            n1217 = Divide(x=w2024, y=w2025) -> (x/y=w2004:dbl)
            n1218 = Divide(x=w2019, y=w2021) -> (x/y=w2009:dbl)
            n1219 = Subtract(x=w2004, y=2.371) -> (x-y=w2002:dbl)
            n1220 = Multiply(x=w2012, y=2.0) -> (x*y=w2007:dbl)
            n1221 = Multiply(x=w2009, y=200.0) -> (x*y=w2008:dbl)
            n1222 = Subtract(x=w2007, y=-1.0) -> (x-y=w2005:dbl)
            n1223 = Multiply(x=w2002, y=0.75) -> (x*y=w2000:dbl)
            n1224 = local read "间隙位移比例偏移"() -> (w2041:dbl)
            n1225 = local read "间隙位移零点偏移"() -> (w2040:dbl)
            n1226 = local read "齿条扭矩零点偏移"() -> (w2042:dbl)
            n1227 = local read "齿条扭矩比例偏移"() -> (w2043:dbl)
            n1228 = local read "齿条推拉力比例偏移"() -> (w2039:dbl)
            n1229 = local read "齿条推拉力零点偏移"() -> (w2038:dbl)
            n1230 = call "传感器校订.vi"("零点"=w2042, "比例"=w2043, "传感器"=w2005) -> ("示值"=→"齿条扭矩(Nm)":dbl)  [unwired: 8 in]
            n1231 = call "传感器校订.vi"("零点"=w2040, "比例"=w2041, "传感器"=w2000) -> ("示值"=→"间隙位移(mm)":dbl)  [unwired: 8 in]
            n1232 = call "传感器校订.vi"("零点"=w2038, "比例"=w2039, "传感器"=w2008) -> ("示值"=→"齿条推拉力(N)":dbl)  [unwired: 8 in]
          }
        }
        n1233 = Wait Until Next ms Multiple(millisecond multiple=u32 50 ("毫秒倍数")) -> ()  [unwired: 1 out]
      }
    }
    frame #2 {
      n1234 = dll-call lib="PCI8622_32.dll" fn="PCI8622_StopDeviceProAD" label="StopDeviceProAD"("hDevice"=w2044) -> ("hDevice"=w2045:i32)  [unwired: 4 in, 2 out]
      n1235 = dll-call lib="PCI8622_32.dll" fn="PCI8622_ReleaseDeviceProAD" label="ReleaseDeviceProAD"("hDevice"=w2045) -> ()  [unwired: 5 in, 2 out]
      n1236 = dll-call lib="PCI8622_32.dll" fn="PCI8622_ReleaseDevice" label="ReleaseDevice"("hDevice"=w2044) -> ()  [unwired: 5 in, 2 out]
    }
  }
